vi "Run_old01.vi"(8 "error in (no error)":errorcluster, 11 "Channel in":refnum<class "Channel.lvclass">) -> (0 "error out":errorcluster, 3 "Channel out":refnum<class "Channel.lvclass">)   [LabVIEW 2018, in "Channel.lvclass"]
uses:
  Channel.lvclass
  C:/Users/observer/Desktop/Sparc4GUI/SPARC4_GUI/Device/Device.lvclass
  Channel.lvclass/Channel.ctl
  Interface/Interface.lvclass/Interface.ctl
  Device/Device.lvclass/Device.ctl
  StateMachine/State Machine.lvclass
  Interface/Interface.lvclass
  Device/Device.lvclass
panel:
  out "resp RESUME":string
  out "resp PAUSE":string
  out "error out 2":errorcluster
  out "x = y?":T1
  out "resp ABORT":string
  out "resp STOP":string
  out "resposta do STATUS":string
  out "resp INIT":string
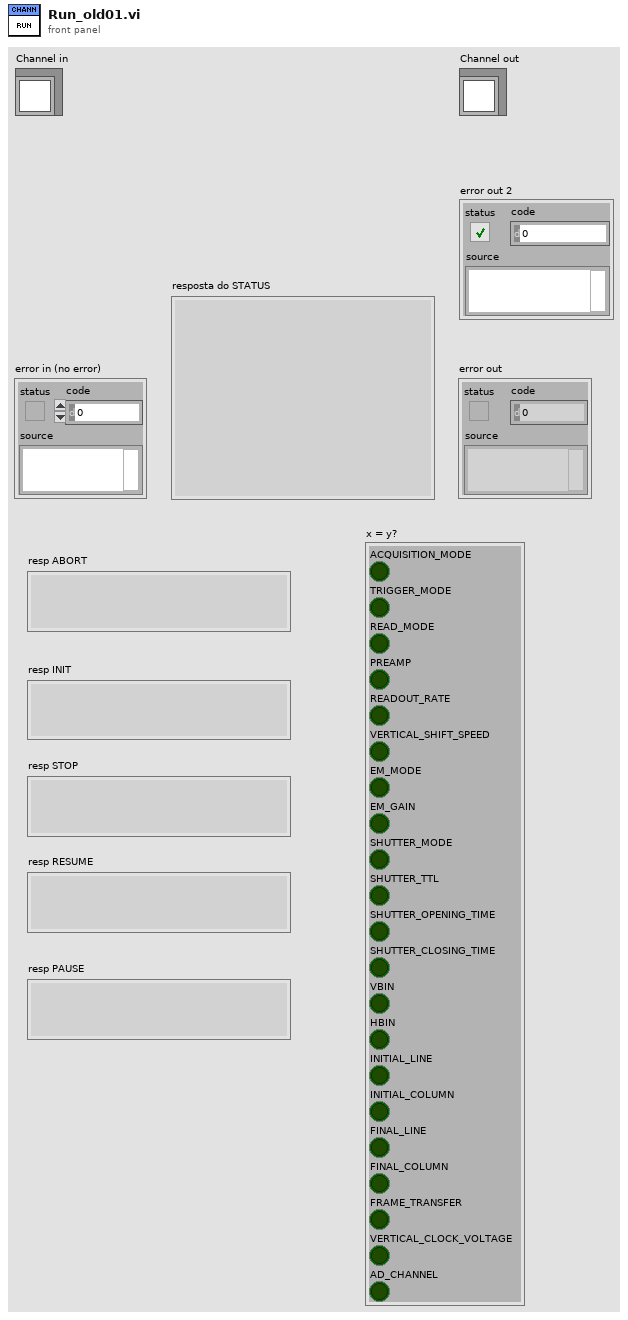
[diagram p1: front panel]
types:
  T1 = cluster{"ACQUISITION_MODE":bool, "TRIGGER_MODE":bool, "READ_MODE":bool, "PREAMP":bool, "READOUT_RATE":bool, "VERTICAL_SHIFT_SPEED":bool, "EM_MODE":bool, "EM_GAIN":bool, "SHUTTER_MODE":bool, "SHUTTER_TTL":bool, "SHUTTER_OPENING_TIME":bool, "SHUTTER_CLOSING_TIME":bool, "VBIN":bool, "HBIN":bool, "INITIAL_LINE":bool, "INITIAL_COLUMN":bool, "FINAL_LINE":bool, "FINAL_COLUMN":bool, "FRAME_TRANSFER":bool, "VERTICAL_CLOCK_VOLTAGE":bool, "AD_CHANNEL":bool}
  T2 = cluster{"ACQUISITION_MODE":u8, "TRIGGER_MODE":u8, "READ_MODE":u8, "PREAMP":u8, "READOUT_RATE":u8, "VERTICAL_SHIFT_SPEED":u8, "EM_MODE":u8, "EM_GAIN":u16, "SHUTTER_MODE":u8, "SHUTTER_TTL":u8, "SHUTTER_OPENING_TIME":u16, "SHUTTER_CLOSING_TIME":u16, "VBIN":u16, "HBIN":u16, "INITIAL_LINE":u16, "INITIAL_COLUMN":u16, "FINAL_LINE":u16, "FINAL_COLUMN":u16, "FRAME_TRANSFER":bool, "VERTICAL_CLOCK_VOLTAGE":u8, "AD_CHANNEL":u32}
  T3 = cluster{"Image Name":string, "Image Path":string, "#FRAMES":u32, "EXPTIME":dbl, "PREAMP":u8, "READOUT_RATE":u8, "VERTICAL_SHIFT_SPEED":u8, "ACQUISITION_MODE":u8, "READ_MODE":u8, "EM_MODE":u8, "EM_GAIN":u16, "SHUTTER_MODE":u8, "SHUTTER_TTL":u8, "SHUTTER_OPENNING_TIME":u16, "SHUTTER_CLOSING_TIME":u16, "VBIN":u16, "HBIN":u16, "INITIAL_LINE":u16, "INITIAL_COLUMN":u16, "FINAL_LINE":u16, "FINAL_COLUMN":u16, "Cooler ON/OFF":u16, "Set temperature":i8, "Exposições realizadas":u16, "Kinetic Serie Length":u32, "Number of Accumulations":u32, "Kinetic Cycle Time":u32, "FRAME_TRANSFER":bool, "VERTICAL_CLOCK_VOLTAGE":u8, "TRIGGER_MODE":u8, "Number of exp":u32, "AD_CHANNEL":u32}
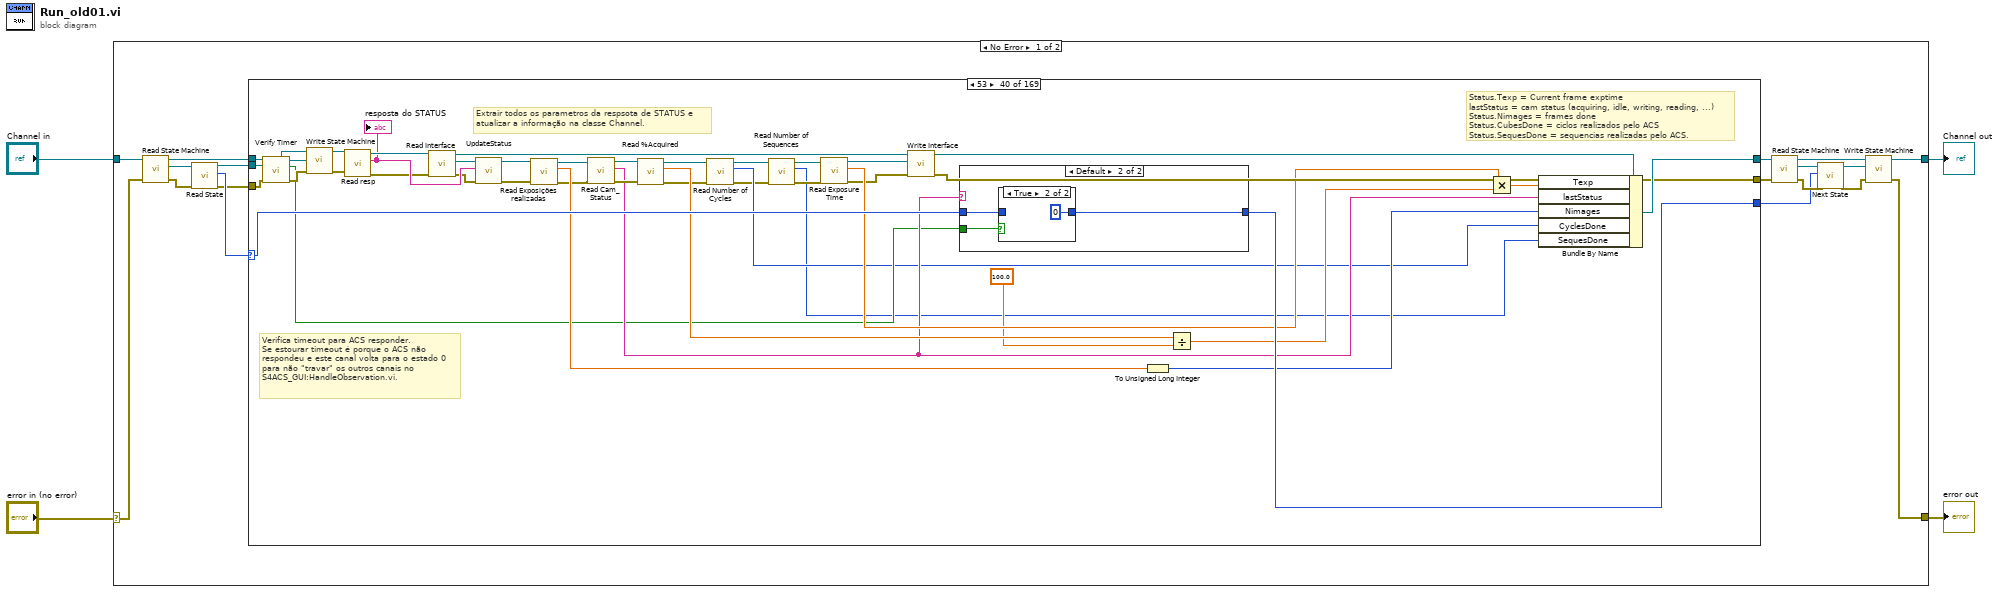
[diagram p0: block diagram]
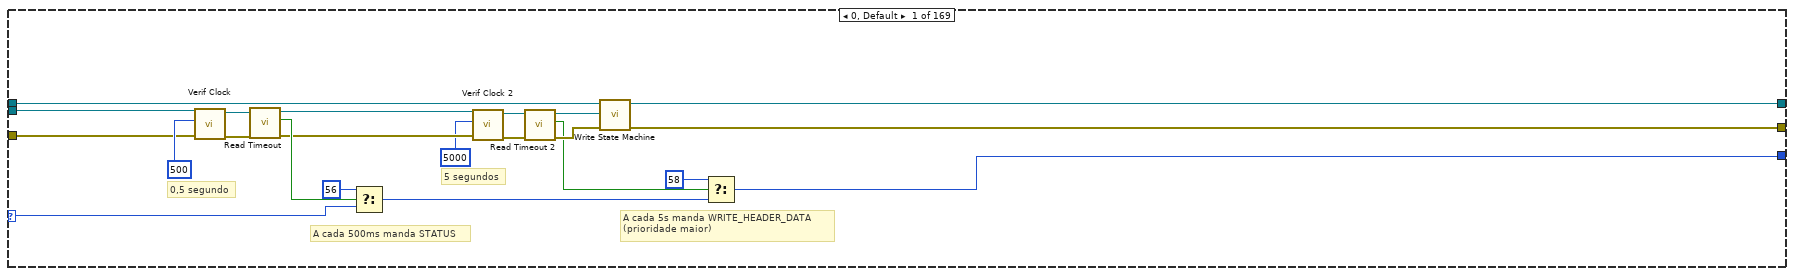
[diagram p2: hidden frame]
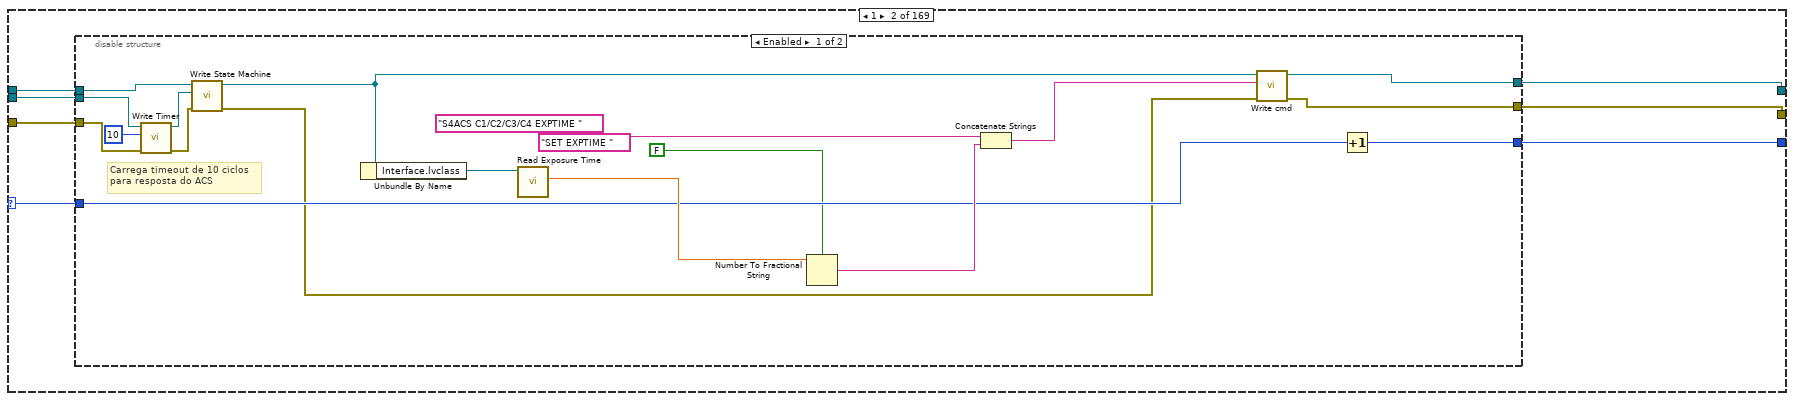
[diagram p3: hidden frame]
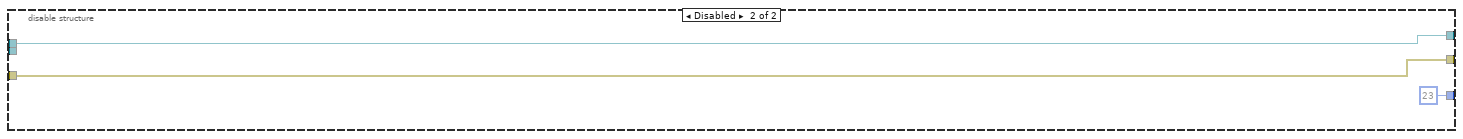
[diagram p4: hidden frame]
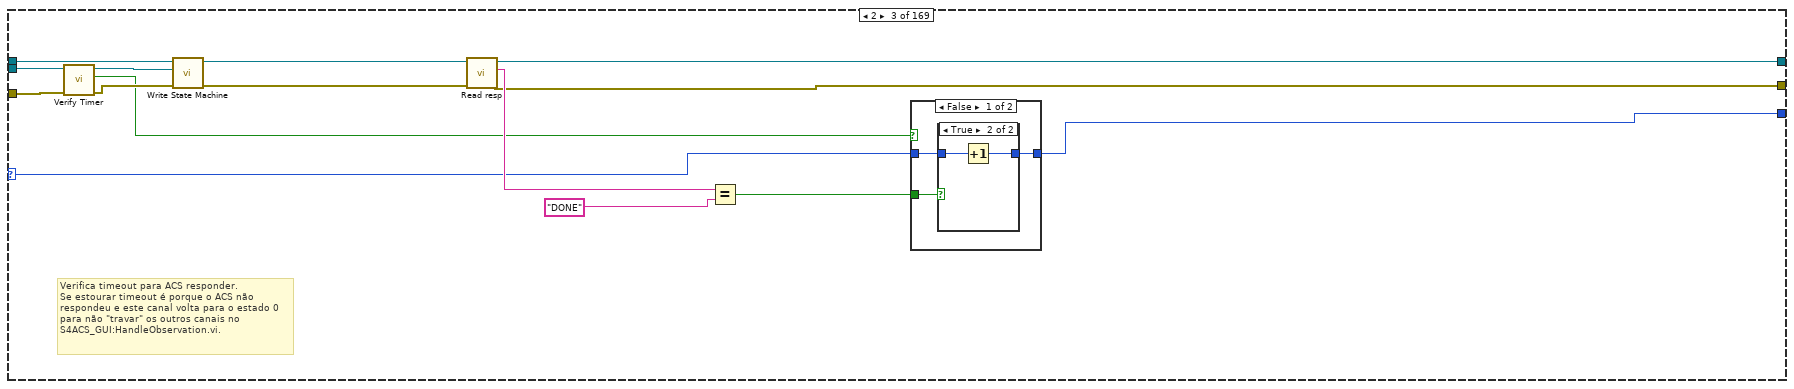
[diagram p5: hidden frame]
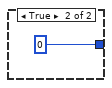
[diagram p7: hidden frame]
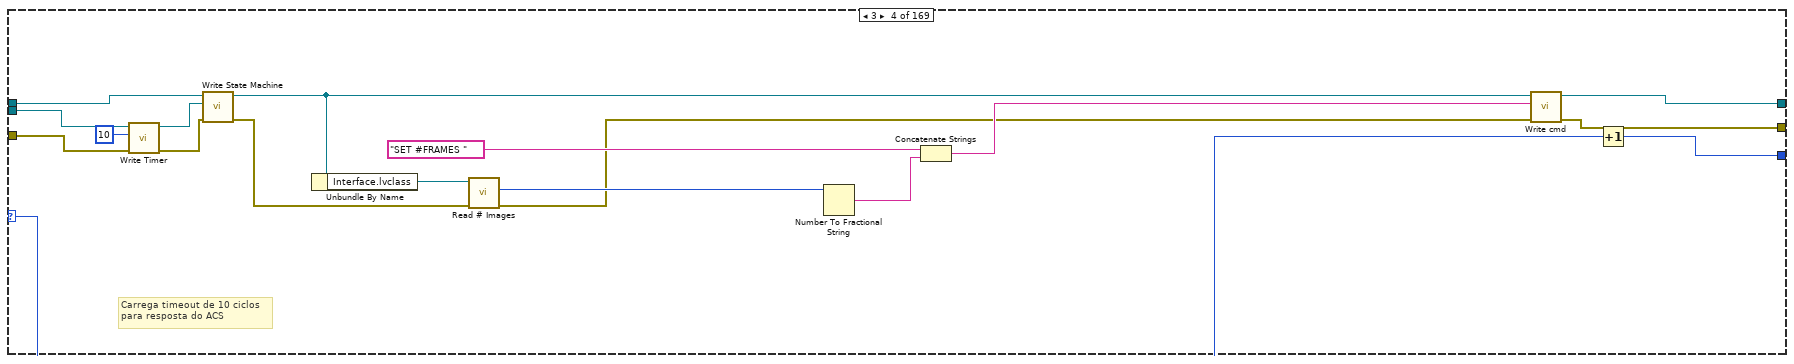
[diagram p8: hidden frame]
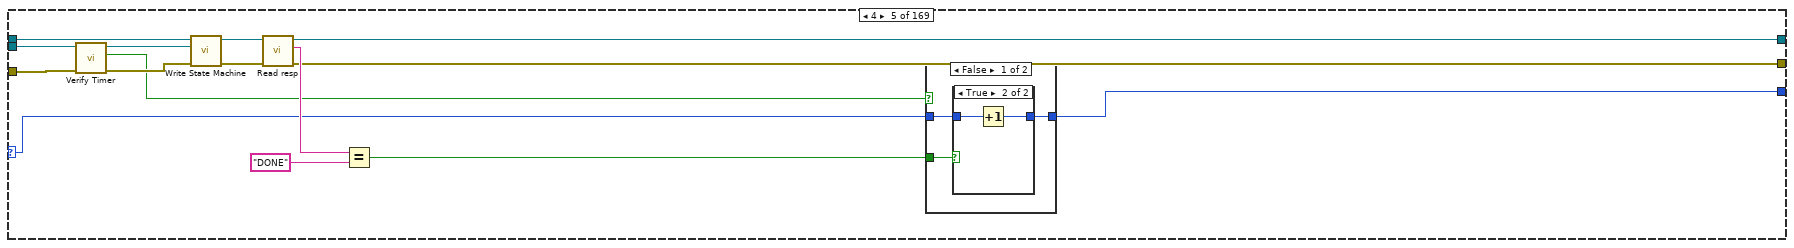
[diagram p9: hidden frame]
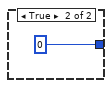
[diagram p11: hidden frame]
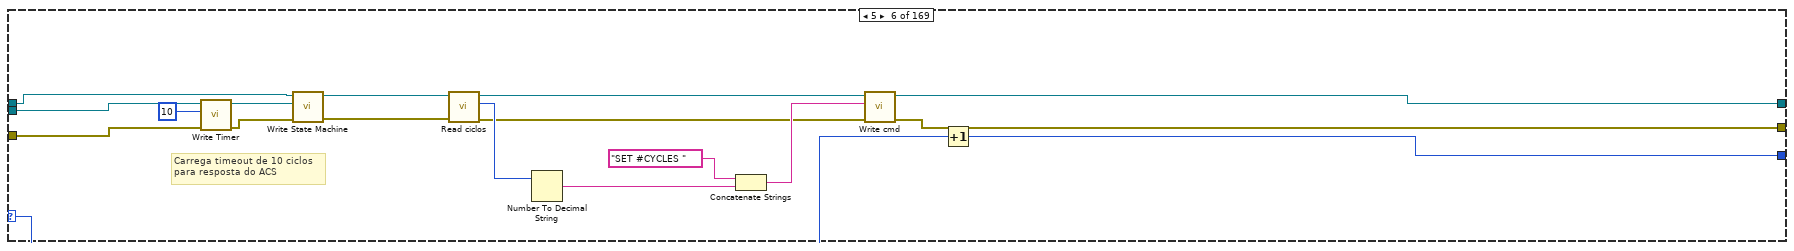
[diagram p12: hidden frame]
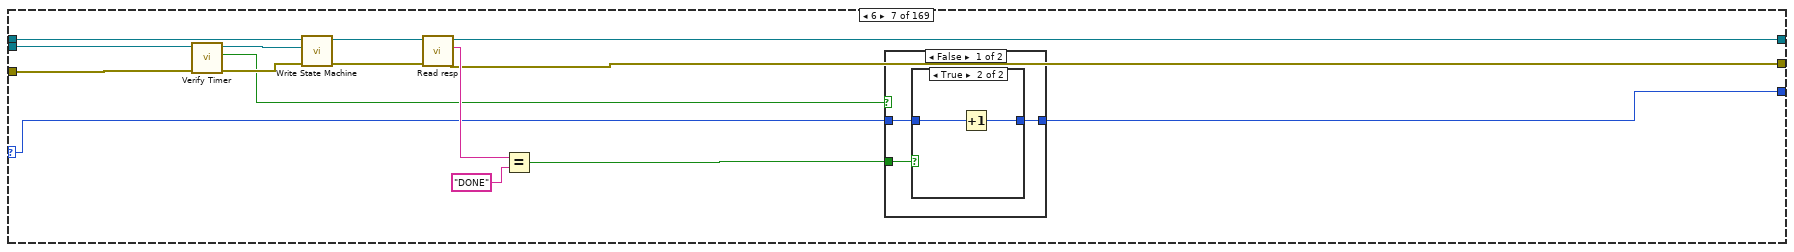
[diagram p13: hidden frame]
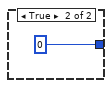
[diagram p15: hidden frame]
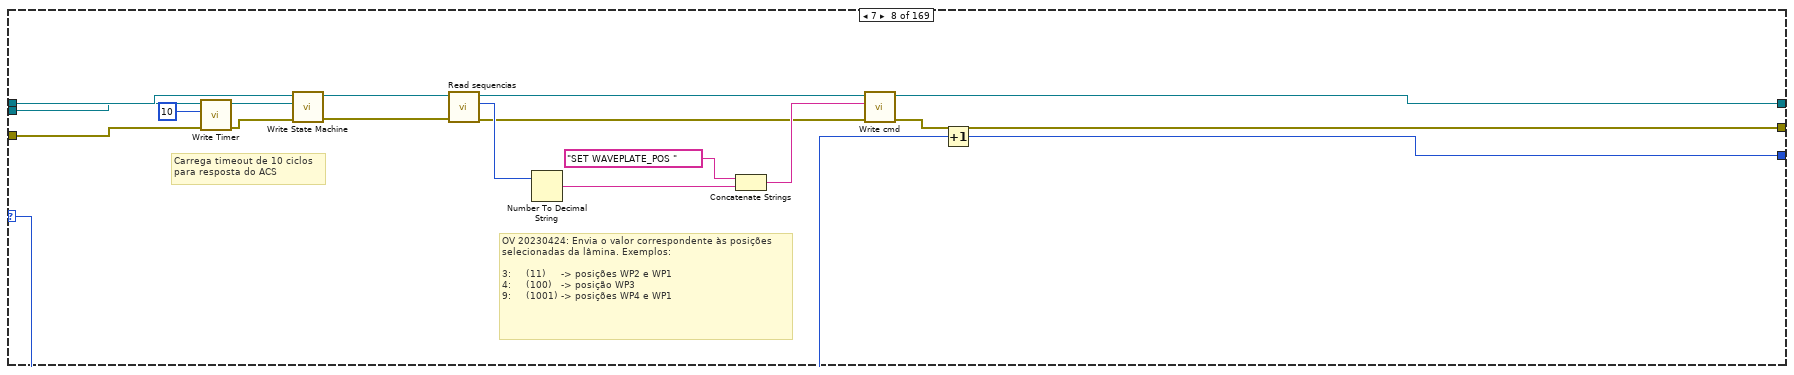
[diagram p16: hidden frame]
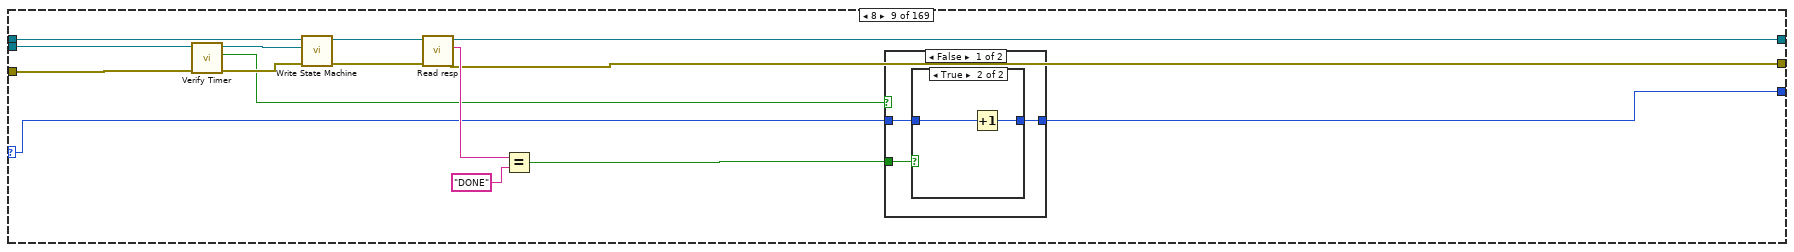
[diagram p17: hidden frame]
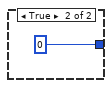
[diagram p19: hidden frame]
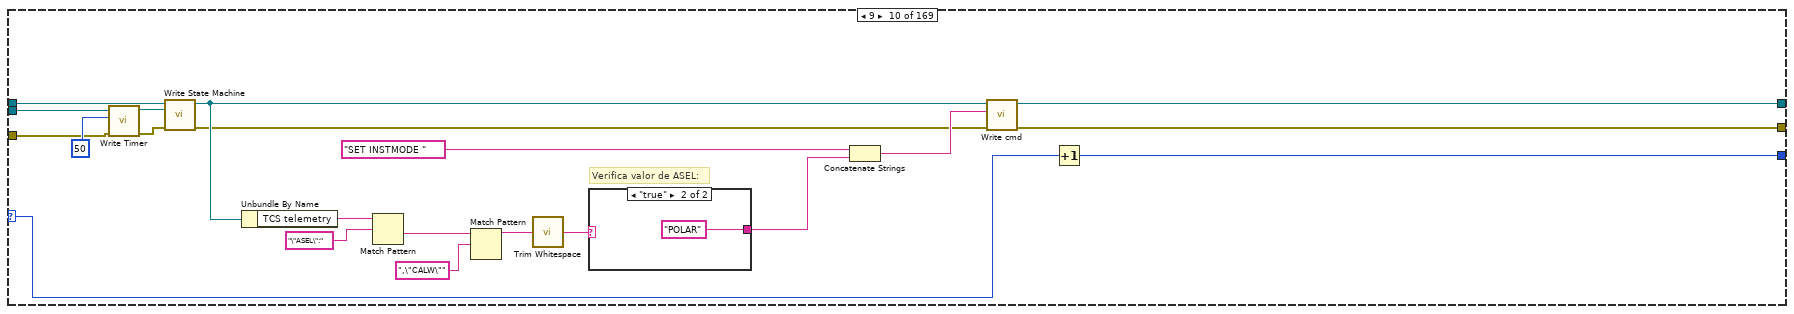
[diagram p20: hidden frame]
diagram:
  n1 = case shown="No Error" "error in (no error)" {
    selector: "error in (no error)" -> [w21 w2733]
    tunnel: [w6 w2733] -> w3
    tunnel: [w11 w2732] -> w1
    tunnel: "Channel in" -> [w22 w2732]
    frame No Error {
      n2 = call-dynamic "Read State Machine.vi"("error in (no error)"=w21, "Device in"=w22) -> ("error out"=w18:errorcluster, "State Machine.lvclass"=w20:refnum<class "State Machine.lvclass">, "Device out"=w16:refnum<class "Channel.lvclass">)  [unwired: 7 in]
      n3 = call-dynamic "Read State.vi"("error in (no error)"=w18, "State Machine in"=w20) -> ("error out"=w17:errorcluster, "State"=w19:i32, "State Machine out"=w5:refnum<class "State Machine.lvclass">)  [unwired: 7 in]
      n4 = case shown="53" w19 {
        selector: w19 -> [w39 w48 w74 w97 w114 w143 w155 w183 w195 w232 w240 w273 w288 w312 w320 w351 w359 w390 w398 w429 w437 w468 w481 w510 w516 w542 w554 w576 w592 w608 w633 w646 w682 w701 _ _ w763 w774 w788 w833 w851 w915 w973 w1021 _ _ w1112 w1144 w1173 w1185 w1199 w1204 w1264 w1286 w1322 w1328 w1342 w1350 w1364 w1371 w1382 _ w1397 w1408 w1428 w1448 w1468 w1488 w1508 w1528 w1548 w1568 _ w1588 w1596 w1609 w1622 w1638 w1646 w1659 w1673 w1685 w1693 w1706 w1719 w1731 w1739 w1752 w1765 w1777 w1785 w1798 w1811 w1823 w1831 w1844 w1857 w1869 w1877 w1890 w1903 w1915 w1923 w1936 w1949 w1961 w1969 w1982 w1995 w2011 w2019 w2032 w2045 w2057 w2065 w2078 w2091 w2103 w2111 w2124 w2137 w2149 w2157 w2170 w2183 w2195 w2203 w2216 w2229 w2241 w2249 w2262 w2275 w2287 w2295 w2308 w2321 w2333 w2341 w2354 w2367 w2379 w2387 w2400 w2413 w2425 w2433 w2446 w2459 w2471 w2479 w2492 w2505 w2521 w2529 w2542 w2555 w2567 w2577 w2590 w2603 w2617 w2625 w2638 w2651 w2664 w2676 w2701 w2713]
        tunnel: w17 -> [w35 w47 w80 w99 w118 w145 w157 w185 w197 w217 w242 w265 w286 w304 w326 w344 w365 w383 w404 w422 w443 w462 w487 w504 w522 w544 w556 w574 w584 w607 w628 w640 w692 w700 w722 w739 w756 w770 w782 w800 w847 w887 w965 w993 w1055 w1087 w1120 w1132 w1167 w1180 w1193 w1221 w1261 w1281 w1315 w1332 w1345 w1354 w1367 w1374 w1385 w1394 w1401 w1412 w1423 w1443 w1463 w1483 w1503 w1523 w1543 w1563 w1581 w1594 w1603 w1613 w1625 w1644 w1653 w1663 w1676 w1691 w1700 w1710 w1722 w1737 w1746 w1756 w1768 w1783 w1792 w1802 w1814 w1829 w1838 w1848 w1860 w1875 w1884 w1894 w1906 w1921 w1930 w1940 w1952 w1967 w1976 w1986 w1998 w2017 w2026 w2036 w2048 w2063 w2072 w2082 w2094 w2109 w2118 w2128 w2140 w2155 w2164 w2174 w2186 w2201 w2210 w2220 w2232 w2247 w2256 w2266 w2278 w2293 w2302 w2312 w2324 w2339 w2348 w2358 w2370 w2385 w2394 w2404 w2416 w2431 w2440 w2450 w2462 w2477 w2486 w2496 w2508 w2527 w2536 w2546 w2558 w2573 w2584 w2594 w2606 w2623 w2632 w2642 w2654 w2666 w2678 w2703 w2715]
        tunnel: [w34 w50 w84 w111 w124 w151 w164 w191 w204 w234 w249 w277 w289 w316 w329 w355 w368 w394 w407 w433 w446 w471 w490 w512 w525 w550 w563 w574 w596 w609 w635 w648 w691 w702 w727 w743 w764 w766 w790 w825 w853 w888 w960 w994 w1067 w1098 w1119 w1145 w1175 w1177 w1201 w1205 w1266 w1287 w1302 w1329 w1338 w1351 w1360 w1372 w1378 w1387 w1400 w1409 w1423 w1443 w1463 w1483 w1503 w1523 w1543 w1563 w1581 w1593 w1597 w1612 w1623 w1643 w1647 w1662 w1674 w1690 w1694 w1709 w1720 w1736 w1740 w1755 w1766 w1782 w1786 w1801 w1812 w1828 w1832 w1847 w1858 w1874 w1878 w1893 w1904 w1920 w1924 w1939 w1950 w1966 w1970 w1985 w1996 w2016 w2020 w2035 w2046 w2062 w2066 w2081 w2092 w2108 w2112 w2127 w2138 w2154 w2158 w2173 w2184 w2200 w2204 w2219 w2230 w2246 w2250 w2265 w2276 w2292 w2296 w2311 w2322 w2338 w2342 w2357 w2368 w2384 w2388 w2403 w2414 w2430 w2434 w2449 w2460 w2476 w2480 w2495 w2506 w2526 w2530 w2545 w2556 w2572 w2578 w2593 w2604 w2622 w2626 w2641 w2652 w2672 w2685 w2709 w2722] -> w7
        tunnel: w16 -> [w38 w45 w83 w100 w122 w146 w161 w186 w201 w219 w246 w267 w285 w306 w327 w346 w366 w385 w405 w424 w444 w464 w488 w506 w523 w545 w560 w573 w587 w606 w630 w643 w690 w699 w725 w740 w758 w773 w784 w803 w850 w885 w967 w987 w1066 w1097 w1114 w1136 w1168 w1181 w1194 w1222 w1260 w1284 w1316 w1333 w1344 w1355 w1366 w1375 w1384 w1395 w1399 w1413 w1421 w1441 w1461 w1481 w1501 w1521 w1541 w1561 w1583 w1592 w1604 w1611 w1626 w1642 w1654 w1661 w1677 w1689 w1701 w1708 w1723 w1735 w1747 w1754 w1769 w1781 w1793 w1800 w1815 w1827 w1839 w1846 w1861 w1873 w1885 w1892 w1907 w1919 w1931 w1938 w1953 w1965 w1977 w1984 w1999 w2015 w2027 w2034 w2049 w2061 w2073 w2080 w2095 w2107 w2119 w2126 w2141 w2153 w2165 w2172 w2187 w2199 w2211 w2218 w2233 w2245 w2257 w2264 w2279 w2291 w2303 w2310 w2325 w2337 w2349 w2356 w2371 w2383 w2395 w2402 w2417 w2429 w2441 w2448 w2463 w2475 w2487 w2494 w2509 w2525 w2537 w2544 w2559 w2571 w2585 w2592 w2607 w2621 w2633 w2640 w2655 w2667 w2682 w2704 w2719]
        tunnel: [w37 w51 w85 w112 w125 w152 w165 w192 w205 w235 w250 w278 w290 w317 w330 w356 w369 w395 w408 w434 w447 w472 w491 w513 w526 w551 w564 w573 w597 w610 w636 w651 w683 w703 w728 w744 w765 w767 w791 w832 w854 w914 w961 w1020 w1068 w1099 w1121 w1146 w1176 w1178 w1202 w1217 w1267 w1288 w1308 w1330 w1337 w1352 w1359 w1373 w1377 w1393 w1402 w1405 w1425 w1445 w1465 w1485 w1505 w1525 w1545 w1565 w1583 w1595 w1598 w1614 w1621 w1645 w1648 w1664 w1672 w1692 w1695 w1711 w1718 w1738 w1741 w1757 w1764 w1784 w1787 w1803 w1810 w1830 w1833 w1849 w1856 w1876 w1879 w1895 w1902 w1922 w1925 w1941 w1948 w1968 w1971 w1987 w1994 w2018 w2021 w2037 w2044 w2064 w2067 w2083 w2090 w2110 w2113 w2129 w2136 w2156 w2159 w2175 w2182 w2202 w2205 w2221 w2228 w2248 w2251 w2267 w2274 w2294 w2297 w2313 w2320 w2340 w2343 w2359 w2366 w2386 w2389 w2405 w2412 w2432 w2435 w2451 w2458 w2478 w2481 w2497 w2504 w2528 w2531 w2547 w2554 w2574 w2579 w2595 w2602 w2624 w2627 w2643 w2650 w2673 w2686 w2710 w2723] -> w14
        tunnel: [w33 w49 w73 w106 w113 w150 w156 w190 w196 w233 w241 w274 w291 w313 w318 w352 w357 w391 w396 w430 w435 w469 w479 w511 w514 w549 w555 w577 w593 w611 w634 w647 w684 w704 31 ("State") 0 ("State") w752 w775 w789 w834 w852 w916 w974 w1022 0 ("State") 54 ("State") w1111 w1147 w1174 w1186 w1200 w1203 w1265 w1289 w1323 w1331 w1343 w1353 w1365 w1371 w1383 w1386 w1398 w1410 w1420 w1440 w1460 w1480 w1500 w1520 w1540 w1560 u8 0 ("State") w1589 w1599 w1610 w1624 w1639 w1649 w1660 w1675 w1686 w1696 w1707 w1721 w1732 w1742 w1753 w1767 w1778 w1788 w1799 w1813 w1824 w1834 w1845 w1859 w1870 w1880 w1891 w1905 w1916 w1926 w1937 w1951 w1962 w1972 w1983 w1997 w2012 w2022 w2033 w2047 w2058 w2068 w2079 w2093 w2104 w2114 w2125 w2139 w2150 w2160 w2171 w2185 w2196 w2206 w2217 w2231 w2242 w2252 w2263 w2277 w2288 w2298 w2309 w2323 w2334 w2344 w2355 w2369 w2380 w2390 w2401 w2415 w2426 w2436 w2447 w2461 w2472 w2482 w2493 w2507 w2522 w2532 w2543 w2557 w2568 w2580 w2591 w2605 w2618 w2628 w2639 w2653 w2671 w2677 w2708 w2714] -> w8
        tunnel: w5 -> [w36 w46 w82 w101 w123 w144 w158 w184 w198 w215 w243 w269 w287 w301 w324 w340 w363 w379 w402 w418 w441 w460 w485 w503 w520 w543 w557 _ w586 w604 w629 w644 _ w697 w724 w741 w759 w772 w783 w805 w848 w886 w969 w992 w1056 w1088 w1116 w1137 w1170 w1182 w1196 w1223 w1262 w1285 w1317 _ _ _ _ _ _ w1389 _ _ _ _ _ _ _ _ _ _ _ _ _ _ _ _ _ _ _ _ _ _ _ _ _ _ _ _ _ _ _ _ _ _ _ _ _ _ _ _ _ _ _ _ _ _ _ _ _ _ _ _ _ _ _ _ _ _ _ _ _ _ _ _ _ _ _ _ _ _ _ _ _ _ _ _ _ _ _ _ _ _ _ _ _ _ _ _ _ _ _ _ _ _ _ _ _ _ _ _ _ _ _ w2665 w2679 w2702 w2716]
        frame 0, Default {
          # "5 segundos"
          # "A cada 5s manda WRITE_HEADER_DATA\n(prioridade maior)"
          # "A cada 500ms manda STATUS"
          # "0,5 segundo"
          n5 = call-dynamic "Verif Clock.vi"("error in (no error)"=w35, "period"=u32 500, "State Machine in"=w36) -> ("error out"=w42:errorcluster, "State Machine out"=w41:refnum<class "State Machine.lvclass">)  [unwired: 7 in]
          n6 = call-dynamic "Read Timeout.vi"("error in (no error)"=w42, "State Machine in"=w41) -> ("error out"=w27:errorcluster, "Timeout"=w43:bool, "State Machine out"=w30:refnum<class "State Machine.lvclass">)  [unwired: 7 in]
          n7 = Select(t=56 ("State"), s=w43, f=w39) -> (s? t:f=w31:i32)
          n8 = call-dynamic "Verif Clock 2.vi"("error in (no error)"=w27, "period"=u32 5000, "State Machine in"=w30) -> ("error out"=w26:errorcluster, "State Machine out"=w29:refnum<class "State Machine.lvclass">)  [unwired: 7 in]
          n9 = call-dynamic "Read Timeout 2.vi"("error in (no error)"=w26, "State Machine in"=w29) -> ("error out"=w25:errorcluster, "Timeout 2"=w23:bool, "State Machine out"=w28:refnum<class "State Machine.lvclass">)  [unwired: 7 in]
          n10 = call-dynamic "Write State Machine.vi"("error in (no error)"=w25, "State Machine.lvclass"=w28, "Device in"=w38) -> ("error out"=w34:errorcluster, "Device out"=w37:refnum<class "Channel.lvclass">)  [unwired: 7 in]
          n11 = Select(t=58 ("f"), s=w23, f=w31) -> (s? t:f=w33:i32)
        }
        frame 1 {
          n12 = disable-structure shown="Enabled" {
            disable-tunnel: [w69 w72] -> w51
            disable-tunnel: [w68 w71] -> w50
            disable-tunnel: [w63 23] -> w49
            disable-tunnel: w48 -> [w62 _]
            disable-tunnel: w47 -> [w59 w71]
            disable-tunnel: w46 -> [w58 _]
            disable-tunnel: w45 -> [w57 w72]
            frame Enabled {
              (unwired) "S4ACS C1/C2/C3/C4 EXPTIME " ("cmd")
              # "Carrega timeout de 10 ciclos\npara resposta do ACS"
              n13 = call-dynamic "Write Timer.vi"("error in (no error)"=w59, "Timer"=u32 10, "State Machine in"=w58) -> ("error out"=w53:errorcluster, "State Machine out"=w56:refnum<class "State Machine.lvclass">)  [unwired: 7 in]
              n14 = call-dynamic "Write State Machine.vi"("error in (no error)"=w53, "State Machine.lvclass"=w56, "Device in"=w57) -> ("error out"=w52:errorcluster, "Device out"=w55:refnum<class "Channel.lvclass">)  [unwired: 7 in]
              n15 = Unbundle By Name(w55) -> ("Interface.lvclass"=w67:refnum<class "Interface.lvclass">)
              n16 = call "Read Exposure Time.vi"("Interface in"=w67) -> ("Exposure Time"=w66:dbl)  [unwired: 8 in, 2 out]
              n17 = Number To Fractional String(use system decimal point (T)=FALSE, number=w66) -> (F-format string=w65:string)  [unwired: 2 in]
              n18 = Concatenate Strings("SET EXPTIME " ("cmd"), w65) -> (w64:string)
              n19 = call-dynamic "Write cmd.vi"("error in (no error)"=w52, "cmd"=w64, "Device in"=w55) -> ("error out"=w68:errorcluster, "Device out"=w69:refnum<class "Channel.lvclass">)  [unwired: 7 in]
              n20 = Increment(x=w62) -> (x+1=w63:i32)
            }
            frame Disabled {
            }
          }
        }
        frame 2 {
          # "Verifica timeout para ACS responder.\nSe estourar timeout é porque o ACS não \nrespondeu e este canal volta para o estado 0\npara não \"travar\" os outros canais no \nS4ACS_GUI:HandleObservation.vi."
          n21 = call "Verify Timer.vi"("error in (no error)"=w80, "State Machine in"=w82) -> ("error out"=w79:errorcluster, "timeout"=w75:bool, "State Machine out"=w81:refnum<class "State Machine.lvclass">)  [unwired: 7 in]
          n22 = call-dynamic "Write State Machine.vi"("error in (no error)"=w79, "State Machine.lvclass"=w81, "Device in"=w83) -> ("error out"=w78:errorcluster, "Device out"=w77:refnum<class "Channel.lvclass">)  [unwired: 7 in]
          n23 = call-dynamic "Read resp.vi"("error in (no error)"=w78, "Device in"=w77) -> ("error out"=w84:errorcluster, "resp"=w87:string, "Device out"=w85:refnum<class "Channel.lvclass">)  [unwired: 7 in]
          n24 = Equal?(x=w87, y="DONE") -> (x = y?=w76:bool)
          n25 = case shown="False" w75 {
            tunnel: [w89 0] -> w73
            tunnel: w74 -> [w90 _]
            tunnel: w76 -> [w88 _]
            frame False {
              n26 = case shown="True" w88 {
                tunnel: [w91 w92] -> w89
                tunnel: w90 -> [w91 w93]
                frame False {
                }
                frame True {
                  n27 = Increment(x=w93) -> (x+1=w92:i32)
                }
              }
            }
            frame True {
            }
          }
        }
        frame 3 {
          # "Carrega timeout de 10 ciclos\npara resposta do ACS"
          n28 = call-dynamic "Write Timer.vi"("error in (no error)"=w99, "Timer"=u32 10, "State Machine in"=w101) -> ("error out"=w102:errorcluster, "State Machine out"=w104:refnum<class "State Machine.lvclass">)  [unwired: 7 in]
          n29 = call-dynamic "Write State Machine.vi"("error in (no error)"=w102, "State Machine.lvclass"=w104, "Device in"=w100) -> ("error out"=w96:errorcluster, "Device out"=w98:refnum<class "Channel.lvclass">)  [unwired: 7 in]
          n30 = Unbundle By Name(w98) -> ("Interface.lvclass"=w110:refnum<class "Interface.lvclass">)
          n31 = call-dynamic "Read # Images.vi"("error in (no error)"=w96, "Interface in"=w110) -> ("error out"=w95:errorcluster, "# Images"=w109:u32)  [unwired: 7 in, 1 out]
          n32 = Number To Fractional String(number=w109) -> (F-format string=w108:string)  [unwired: 3 in]
          n33 = Concatenate Strings("SET #FRAMES " ("cmd"), w108) -> (w107:string)
          n34 = call-dynamic "Write cmd.vi"("error in (no error)"=w95, "cmd"=w107, "Device in"=w98) -> ("error out"=w111:errorcluster, "Device out"=w112:refnum<class "Channel.lvclass">)  [unwired: 7 in]
          n35 = Increment(x=w97) -> (x+1=w106:i32)
        }
        frame 4 {
          n36 = call "Verify Timer.vi"("error in (no error)"=w118, "State Machine in"=w123) -> ("error out"=w117:errorcluster, "timeout"=w116:bool, "State Machine out"=w119:refnum<class "State Machine.lvclass">)  [unwired: 7 in]
          n37 = call-dynamic "Write State Machine.vi"("error in (no error)"=w117, "State Machine.lvclass"=w119, "Device in"=w122) -> ("error out"=w120:errorcluster, "Device out"=w121:refnum<class "Channel.lvclass">)  [unwired: 7 in]
          n38 = call-dynamic "Read resp.vi"("error in (no error)"=w120, "Device in"=w121) -> ("error out"=w124:errorcluster, "resp"=w127:string, "Device out"=w125:refnum<class "Channel.lvclass">)  [unwired: 7 in]
          n39 = Equal?(x=w127, y="DONE") -> (x = y?=w115:bool)
          n40 = case shown="False" w116 {
            tunnel: [w129 0] -> w113
            tunnel: w114 -> [w130 _]
            tunnel: w115 -> [w128 _]
            frame False {
              n41 = case shown="True" w128 {
                tunnel: [w131 w132] -> w129
                tunnel: w130 -> [w131 w133]
                frame False {
                }
                frame True {
                  n42 = Increment(x=w133) -> (x+1=w132:i32)
                }
              }
            }
            frame True {
            }
          }
        }
        frame 5 {
          # "Carrega timeout de 10 ciclos\npara resposta do ACS"
          n43 = call-dynamic "Write Timer.vi"("error in (no error)"=w145, "Timer"=u32 10, "State Machine in"=w144) -> ("error out"=w147:errorcluster, "State Machine out"=w149:refnum<class "State Machine.lvclass">)  [unwired: 7 in]
          n44 = call-dynamic "Write State Machine.vi"("error in (no error)"=w147, "State Machine.lvclass"=w149, "Device in"=w146) -> ("error out"=w141:errorcluster, "Device out"=w142:refnum<class "Channel.lvclass">)  [unwired: 7 in]
          n45 = call-dynamic "Read ciclos.vi"("error in (no error)"=w141, "Channel in"=w142) -> ("error out"=w135:errorcluster, "ciclos"=w139:u32, "Channel out"=w140:refnum<class "Channel.lvclass">)  [unwired: 7 in]
          n46 = Number To Decimal String(number=w139) -> (decimal integer string=w137:string)  [unwired: 1 in]
          n47 = Concatenate Strings("SET #CYCLES " ("cmd"), w137) -> (w136:string)
          n48 = call-dynamic "Write cmd.vi"("error in (no error)"=w135, "cmd"=w136, "Device in"=w140) -> ("error out"=w151:errorcluster, "Device out"=w152:refnum<class "Channel.lvclass">)  [unwired: 7 in]
          n49 = Increment(x=w143) -> (x+1=w150:i32)
        }
        frame 6 {
          n50 = call "Verify Timer.vi"("error in (no error)"=w157, "State Machine in"=w158) -> ("error out"=w162:errorcluster, "timeout"=w154:bool, "State Machine out"=w163:refnum<class "State Machine.lvclass">)  [unwired: 7 in]
          n51 = call-dynamic "Write State Machine.vi"("error in (no error)"=w162, "State Machine.lvclass"=w163, "Device in"=w161) -> ("error out"=w159:errorcluster, "Device out"=w160:refnum<class "Channel.lvclass">)  [unwired: 7 in]
          n52 = call-dynamic "Read resp.vi"("error in (no error)"=w159, "Device in"=w160) -> ("error out"=w164:errorcluster, "resp"=w167:string, "Device out"=w165:refnum<class "Channel.lvclass">)  [unwired: 7 in]
          n53 = Equal?(x=w167, y="DONE") -> (x = y?=w153:bool)
          n54 = case shown="False" w154 {
            tunnel: [w169 0] -> w156
            tunnel: w155 -> [w170 _]
            tunnel: w153 -> [w168 _]
            frame False {
              n55 = case shown="True" w168 {
                tunnel: [w171 w172] -> w169
                tunnel: w170 -> [w171 w173]
                frame False {
                }
                frame True {
                  n56 = Increment(x=w173) -> (x+1=w172:i32)
                }
              }
            }
            frame True {
            }
          }
        }
        frame 7 {
          # "OV 20230424: Envia o valor correspondente às posições\nselecionadas da lâmina. Exemplos:\n\n3:     (11)     -> posições WP2 e WP1\n4:     (100)   -> posição WP3\n9:     (1001) -> posições WP4 e WP1"
          # "Carrega timeout de 10 ciclos\npara resposta do ACS"
          n57 = call-dynamic "Write Timer.vi"("error in (no error)"=w185, "Timer"=u32 10, "State Machine in"=w184) -> ("error out"=w187:errorcluster, "State Machine out"=w189:refnum<class "State Machine.lvclass">)  [unwired: 7 in]
          n58 = call-dynamic "Write State Machine.vi"("error in (no error)"=w187, "State Machine.lvclass"=w189, "Device in"=w186) -> ("error out"=w181:errorcluster, "Device out"=w182:refnum<class "Channel.lvclass">)  [unwired: 7 in]
          n59 = call-dynamic "Read sequencias.vi"("error in (no error)"=w181, "Channel in"=w182) -> ("error out"=w175:errorcluster, "sequencias"=w179:u32, "Channel out"=w180:refnum<class "Channel.lvclass">)  [unwired: 7 in]
          n60 = Number To Decimal String(number=w179) -> (decimal integer string=w177:string)  [unwired: 1 in]
          n61 = Concatenate Strings("SET WAVEPLATE_POS " ("cmd"), w177) -> (w176:string)
          n62 = call-dynamic "Write cmd.vi"("error in (no error)"=w175, "cmd"=w176, "Device in"=w180) -> ("error out"=w191:errorcluster, "Device out"=w192:refnum<class "Channel.lvclass">)  [unwired: 7 in]
          n63 = Increment(x=w183) -> (x+1=w190:i32)
        }
        frame 8 {
          n64 = call "Verify Timer.vi"("error in (no error)"=w197, "State Machine in"=w198) -> ("error out"=w202:errorcluster, "timeout"=w194:bool, "State Machine out"=w203:refnum<class "State Machine.lvclass">)  [unwired: 7 in]
          n65 = call-dynamic "Write State Machine.vi"("error in (no error)"=w202, "State Machine.lvclass"=w203, "Device in"=w201) -> ("error out"=w199:errorcluster, "Device out"=w200:refnum<class "Channel.lvclass">)  [unwired: 7 in]
          n66 = call-dynamic "Read resp.vi"("error in (no error)"=w199, "Device in"=w200) -> ("error out"=w204:errorcluster, "resp"=w207:string, "Device out"=w205:refnum<class "Channel.lvclass">)  [unwired: 7 in]
          n67 = Equal?(x=w207, y="DONE") -> (x = y?=w193:bool)
          n68 = case shown="False" w194 {
            tunnel: [w209 0] -> w196
            tunnel: w195 -> [w210 _]
            tunnel: w193 -> [w208 _]
            frame False {
              n69 = case shown="True" w208 {
                tunnel: [w211 w212] -> w209
                tunnel: w210 -> [w211 w213]
                frame False {
                }
                frame True {
                  n70 = Increment(x=w213) -> (x+1=w212:i32)
                }
              }
            }
            frame True {
            }
          }
        }
        frame 9 {
          # "Verifica valor de ASEL:"
          n71 = call-dynamic "Write Timer.vi"("error in (no error)"=w217, "Timer"=u32 50, "State Machine in"=w215) -> ("error out"=w222:errorcluster, "State Machine out"=w220:refnum<class "State Machine.lvclass">)  [unwired: 7 in]
          n72 = call-dynamic "Write State Machine.vi"("error in (no error)"=w222, "State Machine.lvclass"=w220, "Device in"=w219) -> ("error out"=w216:errorcluster, "Device out"=w218:refnum<class "Channel.lvclass">)  [unwired: 7 in]
          n73 = Unbundle By Name(w218) -> ("TCS telemetry"=w231:string)
          n74 = Match Pattern(string=w231, regular expression="\"ASEL\":") -> (after substring=w229:string)  [unwired: 1 in, 3 out]
          n75 = Match Pattern(string=w229, regular expression=",\"CALW\"") -> (before substring=w227:string)  [unwired: 1 in, 3 out]
          n76 = call <vilib>:"Trim Whitespace.vi"("string"=w227) -> ("trimmed string"=w226:string)  [unwired: 1 in]
          n77 = case shown="\"true\"" w226 {
            tunnel: ["PHOT" ("regular expression") "POLAR" ("regular expression")] -> w224
            frame "false", Default {
            }
            frame "true" {
            }
          }
          n78 = Concatenate Strings("SET INSTMODE " ("cmd"), w224) -> (w223:string)
          n79 = call-dynamic "Write cmd.vi"("error in (no error)"=w216, "cmd"=w223, "Device in"=w218) -> ("error out"=w234:errorcluster, "Device out"=w235:refnum<class "Channel.lvclass">)  [unwired: 7 in]
          n80 = Increment(x=w232) -> (x+1=w233:i32)
        }
        frame 10 {
          n81 = call "Verify Timer.vi"("error in (no error)"=w242, "State Machine in"=w243) -> ("error out"=w247:errorcluster, "timeout"=w239:bool, "State Machine out"=w248:refnum<class "State Machine.lvclass">)  [unwired: 7 in]
          n82 = call-dynamic "Write State Machine.vi"("error in (no error)"=w247, "State Machine.lvclass"=w248, "Device in"=w246) -> ("error out"=w244:errorcluster, "Device out"=w245:refnum<class "Channel.lvclass">)  [unwired: 7 in]
          n83 = call-dynamic "Read resp.vi"("error in (no error)"=w244, "Device in"=w245) -> ("error out"=w249:errorcluster, "resp"=w252:string, "Device out"=w250:refnum<class "Channel.lvclass">)  [unwired: 7 in]
          n84 = Equal?(x=w252, y="DONE") -> (x = y?=w238:bool)
          n85 = case shown="False" w239 {
            tunnel: [w254 0] -> w241
            tunnel: w240 -> [w255 _]
            tunnel: w238 -> [w253 _]
            frame False {
              n86 = case shown="True" w253 {
                tunnel: [w256 w257] -> w254
                tunnel: w255 -> [w256 w258]
                frame False {
                }
                frame True {
                  n87 = disable-structure shown="Enabled" {
                    disable-tunnel: w258 -> [w260 _]
                    disable-tunnel: [w259 29 ("State")] -> w257
                    frame Disabled {
                      n88 = Increment(x=w260) -> (x+1=w259:i32)
                    }
                    frame Enabled {
                    }
                  }
                }
              }
            }
            frame True {
            }
          }
        }
        frame 12 {
          # "suffix"
          n89 = call-dynamic "Write Timer.vi"("error in (no error)"=w265, "Timer"=u32 50, "State Machine in"=w269) -> ("error out"=w270:errorcluster, "State Machine out"=w263:refnum<class "State Machine.lvclass">)  [unwired: 7 in]
          n90 = call-dynamic "Write State Machine.vi"("error in (no error)"=w270, "State Machine.lvclass"=w263, "Device in"=w267) -> ("error out"=w264:errorcluster, "Device out"=w266:refnum<class "Channel.lvclass">)  [unwired: 7 in]
          n91 = Unbundle By Name(w266) -> ("Interface.lvclass"=w276:refnum<class "Interface.lvclass">)
          n92 = call-dynamic "Read Suffix.vi"("Interface in"=w276) -> ("Suffix"=w271:string)  [unwired: 8 in, 2 out]
          n93 = Concatenate Strings("SET SUFFIX " ("cmd"), w271) -> (w275:string)
          n94 = call-dynamic "Write cmd.vi"("error in (no error)"=w264, "cmd"=w275, "Device in"=w266) -> ("error out"=w277:errorcluster, "Device out"=w278:refnum<class "Channel.lvclass">)  [unwired: 7 in]
          n95 = Increment(x=w273) -> (x+1=w274:i32)
        }
        frame 13 {
          n96 = call "Verify Timer.vi"("error in (no error)"=w286, "State Machine in"=w287) -> ("error out"=w283:errorcluster, "timeout"=w280:bool, "State Machine out"=w284:refnum<class "State Machine.lvclass">)  [unwired: 7 in]
          n97 = call-dynamic "Write State Machine.vi"("error in (no error)"=w283, "State Machine.lvclass"=w284, "Device in"=w285) -> ("error out"=w282:errorcluster, "Device out"=w281:refnum<class "Channel.lvclass">)  [unwired: 7 in]
          n98 = call-dynamic "Read resp.vi"("error in (no error)"=w282, "Device in"=w281) -> ("error out"=w289:errorcluster, "resp"=w293:string, "Device out"=w290:refnum<class "Channel.lvclass">)  [unwired: 7 in]
          n99 = Equal?(x=w293, y="DONE") -> (x = y?=w279:bool)
          n100 = case shown="False" w280 {
            tunnel: [w295 0] -> w291
            tunnel: w288 -> [w296 _]
            tunnel: w279 -> [w294 _]
            frame False {
              n101 = case shown="True" w294 {
                tunnel: w296 -> [w297 w299]
                tunnel: [w297 w298] -> w295
                frame False {
                }
                frame True {
                  n102 = Increment(x=w299) -> (x+1=w298:i32)
                }
              }
            }
            frame True {
            }
          }
        }
        frame 14 {
          # "obstype"
          n103 = call-dynamic "Write Timer.vi"("error in (no error)"=w304, "Timer"=u32 50, "State Machine in"=w301) -> ("error out"=w309:errorcluster, "State Machine out"=w307:refnum<class "State Machine.lvclass">)  [unwired: 7 in]
          n104 = call-dynamic "Write State Machine.vi"("error in (no error)"=w309, "State Machine.lvclass"=w307, "Device in"=w306) -> ("error out"=w303:errorcluster, "Device out"=w305:refnum<class "Channel.lvclass">)  [unwired: 7 in]
          n105 = Unbundle By Name(w305) -> ("Interface.lvclass"=w315:refnum<class "Interface.lvclass">)
          n106 = call-dynamic "Read ObsType.vi"("error in (no error)"=w303, "Interface in"=w315) -> ("error out"=w302:errorcluster, "ObsType"=w310:string)  [unwired: 7 in, 1 out]
          n107 = Concatenate Strings("SET OBSTYPE " ("cmd"), w310) -> (w314:string)
          n108 = call-dynamic "Write cmd.vi"("error in (no error)"=w302, "cmd"=w314, "Device in"=w305) -> ("error out"=w316:errorcluster, "Device out"=w317:refnum<class "Channel.lvclass">)  [unwired: 7 in]
          n109 = Increment(x=w312) -> (x+1=w313:i32)
        }
        frame 15 {
          n110 = call "Verify Timer.vi"("error in (no error)"=w326, "State Machine in"=w324) -> ("error out"=w325:errorcluster, "timeout"=w321:bool, "State Machine out"=w328:refnum<class "State Machine.lvclass">)  [unwired: 7 in]
          n111 = call-dynamic "Write State Machine.vi"("error in (no error)"=w325, "State Machine.lvclass"=w328, "Device in"=w327) -> ("error out"=w322:errorcluster, "Device out"=w323:refnum<class "Channel.lvclass">)  [unwired: 7 in]
          n112 = call-dynamic "Read resp.vi"("error in (no error)"=w322, "Device in"=w323) -> ("error out"=w329:errorcluster, "resp"=w332:string, "Device out"=w330:refnum<class "Channel.lvclass">)  [unwired: 7 in]
          n113 = Equal?(x=w332, y="DONE") -> (x = y?=w319:bool)
          n114 = case shown="False" w321 {
            tunnel: [w334 0] -> w318
            tunnel: w320 -> [w335 _]
            tunnel: w319 -> [w333 _]
            frame False {
              n115 = case shown="True" w333 {
                tunnel: w335 -> [w336 w338]
                tunnel: [w336 w337] -> w334
                frame False {
                }
                frame True {
                  n116 = Increment(x=w338) -> (x+1=w337:i32)
                }
              }
            }
            frame True {
            }
          }
        }
        frame 16 {
          # "observer"
          n117 = call-dynamic "Write Timer.vi"("error in (no error)"=w344, "Timer"=u32 50, "State Machine in"=w340) -> ("error out"=w349:errorcluster, "State Machine out"=w347:refnum<class "State Machine.lvclass">)  [unwired: 7 in]
          n118 = call-dynamic "Write State Machine.vi"("error in (no error)"=w349, "State Machine.lvclass"=w347, "Device in"=w346) -> ("error out"=w343:errorcluster, "Device out"=w345:refnum<class "Channel.lvclass">)  [unwired: 7 in]
          n119 = Unbundle By Name(w345) -> ("Interface.lvclass"=w354:refnum<class "Interface.lvclass">)
          n120 = call-dynamic "Read Observer.vi"("error in (no error)"=w343, "Interface in"=w354) -> ("error out"=w342:errorcluster, "Observer"=w350:string)  [unwired: 7 in, 1 out]
          n121 = Concatenate Strings("SET OBSERVER " ("cmd"), w350) -> (w353:string)
          n122 = call-dynamic "Write cmd.vi"("error in (no error)"=w342, "cmd"=w353, "Device in"=w345) -> ("error out"=w355:errorcluster, "Device out"=w356:refnum<class "Channel.lvclass">)  [unwired: 7 in]
          n123 = Increment(x=w351) -> (x+1=w352:i32)
        }
        frame 17 {
          n124 = call "Verify Timer.vi"("error in (no error)"=w365, "State Machine in"=w363) -> ("error out"=w364:errorcluster, "timeout"=w360:bool, "State Machine out"=w367:refnum<class "State Machine.lvclass">)  [unwired: 7 in]
          n125 = call-dynamic "Write State Machine.vi"("error in (no error)"=w364, "State Machine.lvclass"=w367, "Device in"=w366) -> ("error out"=w361:errorcluster, "Device out"=w362:refnum<class "Channel.lvclass">)  [unwired: 7 in]
          n126 = call-dynamic "Read resp.vi"("error in (no error)"=w361, "Device in"=w362) -> ("error out"=w368:errorcluster, "resp"=w371:string, "Device out"=w369:refnum<class "Channel.lvclass">)  [unwired: 7 in]
          n127 = Equal?(x=w371, y="DONE") -> (x = y?=w358:bool)
          n128 = case shown="False" w360 {
            tunnel: [w373 0] -> w357
            tunnel: w359 -> [w374 _]
            tunnel: w358 -> [w372 _]
            frame False {
              n129 = case shown="True" w372 {
                tunnel: w374 -> [w375 w377]
                tunnel: [w375 w376] -> w373
                frame False {
                }
                frame True {
                  n130 = Increment(x=w377) -> (x+1=w376:i32)
                }
              }
            }
            frame True {
            }
          }
        }
        frame 18 {
          # "comment"
          n131 = call-dynamic "Write Timer.vi"("error in (no error)"=w383, "Timer"=u32 50, "State Machine in"=w379) -> ("error out"=w388:errorcluster, "State Machine out"=w386:refnum<class "State Machine.lvclass">)  [unwired: 7 in]
          n132 = call-dynamic "Write State Machine.vi"("error in (no error)"=w388, "State Machine.lvclass"=w386, "Device in"=w385) -> ("error out"=w382:errorcluster, "Device out"=w384:refnum<class "Channel.lvclass">)  [unwired: 7 in]
          n133 = Unbundle By Name(w384) -> ("Interface.lvclass"=w393:refnum<class "Interface.lvclass">)
          n134 = call-dynamic "Read Comments.vi"("error in (no error)"=w382, "Interface in"=w393) -> ("error out"=w381:errorcluster, "Comments"=w389:string)  [unwired: 7 in, 1 out]
          n135 = Concatenate Strings("SET COMMENT " ("cmd"), w389) -> (w392:string)
          n136 = call-dynamic "Write cmd.vi"("error in (no error)"=w381, "cmd"=w392, "Device in"=w384) -> ("error out"=w394:errorcluster, "Device out"=w395:refnum<class "Channel.lvclass">)  [unwired: 7 in]
          n137 = Increment(x=w390) -> (x+1=w391:i32)
        }
        frame 19 {
          n138 = call "Verify Timer.vi"("error in (no error)"=w404, "State Machine in"=w402) -> ("error out"=w403:errorcluster, "timeout"=w399:bool, "State Machine out"=w406:refnum<class "State Machine.lvclass">)  [unwired: 7 in]
          n139 = call-dynamic "Write State Machine.vi"("error in (no error)"=w403, "State Machine.lvclass"=w406, "Device in"=w405) -> ("error out"=w400:errorcluster, "Device out"=w401:refnum<class "Channel.lvclass">)  [unwired: 7 in]
          n140 = call-dynamic "Read resp.vi"("error in (no error)"=w400, "Device in"=w401) -> ("error out"=w407:errorcluster, "resp"=w410:string, "Device out"=w408:refnum<class "Channel.lvclass">)  [unwired: 7 in]
          n141 = Equal?(x=w410, y="DONE") -> (x = y?=w397:bool)
          n142 = case shown="False" w399 {
            tunnel: [w412 0] -> w396
            tunnel: w398 -> [w413 _]
            tunnel: w397 -> [w411 _]
            frame False {
              n143 = case shown="True" w411 {
                tunnel: w413 -> [w414 w416]
                tunnel: [w414 w415] -> w412
                frame False {
                }
                frame True {
                  n144 = Increment(x=w416) -> (x+1=w415:i32)
                }
              }
            }
            frame True {
            }
          }
        }
        frame 20 {
          # "object"
          n145 = call-dynamic "Write Timer.vi"("error in (no error)"=w422, "Timer"=u32 50, "State Machine in"=w418) -> ("error out"=w427:errorcluster, "State Machine out"=w425:refnum<class "State Machine.lvclass">)  [unwired: 7 in]
          n146 = call-dynamic "Write State Machine.vi"("error in (no error)"=w427, "State Machine.lvclass"=w425, "Device in"=w424) -> ("error out"=w421:errorcluster, "Device out"=w423:refnum<class "Channel.lvclass">)  [unwired: 7 in]
          n147 = Unbundle By Name(w423) -> ("Interface.lvclass"=w432:refnum<class "Interface.lvclass">)
          n148 = call-dynamic "Read Object.vi"("error in (no error)"=w421, "Interface in"=w432) -> ("error out"=w420:errorcluster, "Object"=w428:string)  [unwired: 7 in, 1 out]
          n149 = Concatenate Strings("SET OBJECT " ("cmd"), w428) -> (w431:string)
          n150 = call-dynamic "Write cmd.vi"("error in (no error)"=w420, "cmd"=w431, "Device in"=w423) -> ("error out"=w433:errorcluster, "Device out"=w434:refnum<class "Channel.lvclass">)  [unwired: 7 in]
          n151 = Increment(x=w429) -> (x+1=w430:i32)
        }
        frame 21 {
          n152 = call "Verify Timer.vi"("error in (no error)"=w443, "State Machine in"=w441) -> ("error out"=w442:errorcluster, "timeout"=w438:bool, "State Machine out"=w445:refnum<class "State Machine.lvclass">)  [unwired: 7 in]
          n153 = call-dynamic "Write State Machine.vi"("error in (no error)"=w442, "State Machine.lvclass"=w445, "Device in"=w444) -> ("error out"=w439:errorcluster, "Device out"=w440:refnum<class "Channel.lvclass">)  [unwired: 7 in]
          n154 = call-dynamic "Read resp.vi"("error in (no error)"=w439, "Device in"=w440) -> ("error out"=w446:errorcluster, "resp"=w449:string, "Device out"=w447:refnum<class "Channel.lvclass">)  [unwired: 7 in]
          n155 = Equal?(x=w449, y="DONE") -> (x = y?=w436:bool)
          n156 = case shown="False" w438 {
            tunnel: [w451 0] -> w435
            tunnel: w437 -> [w452 _]
            tunnel: w436 -> [w450 _]
            frame False {
              n157 = case shown="True" w450 {
                tunnel: w452 -> [w453 w455]
                tunnel: [w453 w454] -> w451
                frame False {
                }
                frame True {
                  n158 = Increment(x=w455) -> (x+1=w454:i32)
                }
              }
            }
            frame True {
            }
          }
        }
        frame 22 {
          # "filter"
          n159 = call-dynamic "Write Timer.vi"("error in (no error)"=w462, "Timer"=u32 50, "State Machine in"=w460) -> ("error out"=w467:errorcluster, "State Machine out"=w465:refnum<class "State Machine.lvclass">)  [unwired: 7 in]
          n160 = call-dynamic "Write State Machine.vi"("error in (no error)"=w467, "State Machine.lvclass"=w465, "Device in"=w464) -> ("error out"=w457:errorcluster, "Device out"=w463:refnum<class "Channel.lvclass">)  [unwired: 7 in]
          n161 = Unbundle By Name(w463) -> ("Filter"=w459:u8)
          n162 = case shown="0, Default" w459 {
            tunnel: ["U" ("cmd") "B" ("cmd") "V" ("cmd") "R" ("cmd") "I" ("cmd") "CLEAR" ("cmd")] -> w458
            frame 1 {
            }
            frame 2 {
            }
            frame 3 {
            }
            frame 4 {
            }
            frame 5 {
            }
            frame 0, Default {
            }
          }
          n163 = Concatenate Strings("SET FILTER " ("cmd"), w458) -> (w470:string)
          n164 = call-dynamic "Write cmd.vi"("error in (no error)"=w457, "cmd"=w470, "Device in"=w463) -> ("error out"=w471:errorcluster, "Device out"=w472:refnum<class "Channel.lvclass">)  [unwired: 7 in]
          n165 = Increment(x=w468) -> (x+1=w469:i32)
        }
        frame 23 {
          n166 = call "Verify Timer.vi"("error in (no error)"=w487, "State Machine in"=w485) -> ("error out"=w486:errorcluster, "timeout"=w482:bool, "State Machine out"=w489:refnum<class "State Machine.lvclass">)  [unwired: 7 in]
          n167 = call-dynamic "Write State Machine.vi"("error in (no error)"=w486, "State Machine.lvclass"=w489, "Device in"=w488) -> ("error out"=w483:errorcluster, "Device out"=w484:refnum<class "Channel.lvclass">)  [unwired: 7 in]
          n168 = call-dynamic "Read resp.vi"("error in (no error)"=w483, "Device in"=w484) -> ("error out"=w490:errorcluster, "resp"=w493:string, "Device out"=w491:refnum<class "Channel.lvclass">)  [unwired: 7 in]
          n169 = Equal?(x=w493, y="DONE") -> (x = y?=w480:bool)
          n170 = case shown="False" w482 {
            tunnel: [w495 0] -> w479
            tunnel: w481 -> [w496 _]
            tunnel: w480 -> [w494 _]
            frame False {
              n171 = case shown="True" w494 {
                tunnel: w496 -> [w497 w499]
                tunnel: [w497 w498] -> w495
                frame False {
                }
                frame True {
                  n172 = Increment(x=w499) -> (x+1=w498:i32)
                }
              }
            }
            frame True {
            }
          }
        }
        frame 24 {
          n173 = call-dynamic "Write Timer.vi"("error in (no error)"=w504, "Timer"=u32 50, "State Machine in"=w503) -> ("error out"=w509:errorcluster, "State Machine out"=w507:refnum<class "State Machine.lvclass">)  [unwired: 7 in]
          n174 = call-dynamic "Write State Machine.vi"("error in (no error)"=w509, "State Machine.lvclass"=w507, "Device in"=w506) -> ("error out"=w502:errorcluster, "Device out"=w505:refnum<class "Channel.lvclass">)  [unwired: 7 in]
          n175 = call-dynamic "Write cmd.vi"("error in (no error)"=w502, "cmd"="SET CTRLINTE S4GUI", "Device in"=w505) -> ("error out"=w512:errorcluster, "Device out"=w513:refnum<class "Channel.lvclass">)  [unwired: 7 in]
          n176 = Increment(x=w510) -> (x+1=w511:i32)
        }
        frame 25 {
          n177 = call "Verify Timer.vi"("error in (no error)"=w522, "State Machine in"=w520) -> ("error out"=w521:errorcluster, "timeout"=w517:bool, "State Machine out"=w524:refnum<class "State Machine.lvclass">)  [unwired: 7 in]
          n178 = call-dynamic "Write State Machine.vi"("error in (no error)"=w521, "State Machine.lvclass"=w524, "Device in"=w523) -> ("error out"=w518:errorcluster, "Device out"=w519:refnum<class "Channel.lvclass">)  [unwired: 7 in]
          n179 = call-dynamic "Read resp.vi"("error in (no error)"=w518, "Device in"=w519) -> ("error out"=w525:errorcluster, "resp"=w528:string, "Device out"=w526:refnum<class "Channel.lvclass">)  [unwired: 7 in]
          n180 = Equal?(x=w528, y="DONE") -> (x = y?=w515:bool)
          n181 = case shown="False" w517 {
            tunnel: [w530 0] -> w514
            tunnel: w516 -> [w531 _]
            tunnel: w515 -> [w529 _]
            frame False {
              n182 = case shown="True" w529 {
                tunnel: w531 -> [w532 w534]
                tunnel: [w532 w533] -> w530
                frame False {
                }
                frame True {
                  n183 = Increment(x=w534) -> (x+1=w533:i32)
                }
              }
            }
            frame True {
            }
          }
        }
        frame 26 {
          # "Carrega timeout de 50 ciclos\npara resposta do ACS"
          n184 = call-dynamic "Write Timer.vi"("error in (no error)"=w544, "Timer"=u32 50, "State Machine in"=w543) -> ("error out"=w546:errorcluster, "State Machine out"=w548:refnum<class "State Machine.lvclass">)  [unwired: 7 in]
          n185 = call-dynamic "Write State Machine.vi"("error in (no error)"=w546, "State Machine.lvclass"=w548, "Device in"=w545) -> ("error out"=w538:errorcluster, "Device out"=w537:refnum<class "Channel.lvclass">)  [unwired: 7 in]
          n186 = Unbundle By Name(w537) -> ("rotator"=w536:dbl)
          n187 = Number To Fractional String(number=w536) -> (F-format string=w540:string)  [unwired: 3 in]
          n188 = Concatenate Strings("SET INSTROT " ("cmd"), w540) -> (w539:string)
          n189 = call-dynamic "Write cmd.vi"("error in (no error)"=w538, "cmd"=w539, "Device in"=w537) -> ("error out"=w550:errorcluster, "Device out"=w551:refnum<class "Channel.lvclass">)  [unwired: 7 in]
          n190 = Increment(x=w542) -> (x+1=w549:i32)
        }
        frame 27 {
          n191 = call "Verify Timer.vi"("error in (no error)"=w556, "State Machine in"=w557) -> ("error out"=w561:errorcluster, "timeout"=w553:bool, "State Machine out"=w562:refnum<class "State Machine.lvclass">)  [unwired: 7 in]
          n192 = call-dynamic "Write State Machine.vi"("error in (no error)"=w561, "State Machine.lvclass"=w562, "Device in"=w560) -> ("error out"=w558:errorcluster, "Device out"=w559:refnum<class "Channel.lvclass">)  [unwired: 7 in]
          n193 = call-dynamic "Read resp.vi"("error in (no error)"=w558, "Device in"=w559) -> ("error out"=w563:errorcluster, "resp"=w566:string, "Device out"=w564:refnum<class "Channel.lvclass">)  [unwired: 7 in]
          n194 = Equal?(x=w566, y="DONE") -> (x = y?=w552:bool)
          n195 = case shown="False" w553 {
            tunnel: [w568 0] -> w555
            tunnel: w554 -> [w569 _]
            tunnel: w552 -> [w567 _]
            frame False {
              n196 = case shown="True" w567 {
                tunnel: [w570 300 ("State")] -> w568
                tunnel: w569 -> [w570 _]
                frame False {
                }
                frame True {
                  # "continua a\nsequencia de\ncomandos SET\nem 300..."
                }
              }
            }
            frame True {
            }
          }
        }
        frame 29 {
          n197 = Unbundle By Name(w573) -> ("expose"=w575:bool)
          n198 = case shown="False" w575 {
            tunnel: [u8 0 ("State") u8 50 ("State")] -> w577
            tunnel: w576 -> [_ _]
            frame False {
            }
            frame True {
            }
          }
        }
        frame 30 {
          n199 = call-dynamic "Write Timer.vi"("error in (no error)"=w584, "Timer"=u32 50, "State Machine in"=w586) -> ("error out"=w583:errorcluster, "State Machine out"=w585:refnum<class "State Machine.lvclass">)  [unwired: 7 in]
          n200 = call-dynamic "Write State Machine.vi"("error in (no error)"=w583, "State Machine.lvclass"=w585, "Device in"=w587) -> ("error out"=w581:errorcluster, "Device out"=w582:refnum<class "Channel.lvclass">)  [unwired: 7 in]
          n201 = Unbundle By Name(w582) -> ("Interface.lvclass"=w595:refnum<class "Interface.lvclass">)
          n202 = call-dynamic "Read Cooler ON_OFF.vi"("error in (no error)"=w581, "Interface in"=w595) -> ("error out"=w580:errorcluster, "Cooler ON/OFF"=w590:i16)  [unwired: 7 in, 1 out]
          n203 = case shown="0" w590 {
            tunnel: ["1" "0"] -> w589
            frame 0 {
              (unwired) "ON"
              # "Se COOLER desligado, manda ligar."
            }
            frame 1, Default {
              (unwired) "OFF"
              # "Se COOLER ligado, manda desligar."
            }
          }
          n204 = Concatenate Strings("SET COOLER_POWER_STATUS " ("cmd"), w589) -> (w594:string)
          n205 = call-dynamic "Write cmd.vi"("error in (no error)"=w580, "cmd"=w594, "Device in"=w582) -> ("error out"=w596:errorcluster, "Device out"=w597:refnum<class "Channel.lvclass">)  [unwired: 7 in]
          n206 = Increment(x=w592) -> (x+1=w593:i32)
        }
        frame 31 {
          n207 = call "Verify Timer.vi"("error in (no error)"=w607, "State Machine in"=w604) -> ("error out"=w602:errorcluster, "timeout"=w600:bool, "State Machine out"=w603:refnum<class "State Machine.lvclass">)  [unwired: 7 in]
          n208 = call-dynamic "Write State Machine.vi"("error in (no error)"=w602, "State Machine.lvclass"=w603, "Device in"=w606) -> ("error out"=w601:errorcluster, "Device out"=w605:refnum<class "Channel.lvclass">)  [unwired: 7 in]
          n209 = call-dynamic "Read resp.vi"("error in (no error)"=w601, "Device in"=w605) -> ("error out"=w609:errorcluster, "resp"=w614:string, "Device out"=w610:refnum<class "Channel.lvclass">)  [unwired: 7 in]
          n210 = Equal?(x=w614, y="DONE") -> (x = y?=w612:bool)
          n211 = case shown="False" w600 {
            tunnel: w612 -> [w617 _]
            tunnel: [w616 w621] -> w611
            tunnel: w608 -> [w615 _]
            frame False {
              n212 = case shown="True" w617 {
                tunnel: [w618 w619] -> w616
                tunnel: w615 -> [w618 w620]
                frame False {
                }
                frame True {
                  n213 = Increment(x=w620) -> (x+1=w619:i32)
                }
              }
            }
            frame True {
              n214 = disable-structure shown="Enabled" {
                disable-tunnel: [0 ("State") 12 ("State")] -> w621
                frame Disabled {
                }
                frame Enabled {
                  # "12: configura os\nparametros por comando\nSET"
                }
              }
            }
          }
        }
        frame 32 {
          n215 = call-dynamic "Write Timer.vi"("error in (no error)"=w628, "Timer"=u32 50, "State Machine in"=w629) -> ("error out"=w631:errorcluster, "State Machine out"=w626:refnum<class "State Machine.lvclass">)  [unwired: 7 in]
          n216 = call-dynamic "Write State Machine.vi"("error in (no error)"=w631, "State Machine.lvclass"=w626, "Device in"=w630) -> ("error out"=w624:errorcluster, "Device out"=w625:refnum<class "Channel.lvclass">)  [unwired: 7 in]
          n217 = call-dynamic "Write cmd.vi"("error in (no error)"=w624, "cmd"="GET COOLER_POWER_STATUS ", "Device in"=w625) -> ("error out"=w635:errorcluster, "Device out"=w636:refnum<class "Channel.lvclass">)  [unwired: 7 in]
          n218 = Increment(x=w633) -> (x+1=w634:i32)
        }
        frame 33 {
          n219 = call "Verify Timer.vi"("error in (no error)"=w640, "State Machine in"=w644) -> ("error out"=w639:errorcluster, "timeout"=w638:bool, "State Machine out"=w641:refnum<class "State Machine.lvclass">)  [unwired: 7 in]
          n220 = call-dynamic "Write State Machine.vi"("error in (no error)"=w639, "State Machine.lvclass"=w641, "Device in"=w643) -> ("error out"=w637:errorcluster, "Device out"=w642:refnum<class "Channel.lvclass">)  [unwired: 7 in]
          n221 = call-dynamic "Read resp.vi"("error in (no error)"=w637, "Device in"=w642) -> ("error out"=w649:errorcluster, "resp"=w645:string, "Device out"=w650:refnum<class "Channel.lvclass">)  [unwired: 7 in]
          n222 = case shown="True" w638 {
            tunnel: [w658 w679] -> w651
            tunnel: w650 -> [w657 w679]
            tunnel: w649 -> [w656 w678]
            tunnel: [w655 w678] -> w648
            tunnel: [w654 w677] -> w647
            tunnel: w646 -> [w653 _]
            tunnel: w645 -> [w652 _]
            frame False {
              n223 = case shown="Default" w652 {
                selector: w652 -> [_ w670]
                tunnel: [w661 w666] -> w658
                tunnel: w657 -> [w661 w674]
                tunnel: w656 -> [w660 w672]
                tunnel: [w660 w664] -> w655
                tunnel: [w659 w671] -> w654
                tunnel: w653 -> [w659 _]
                frame Default {
                }
                frame "0", "1" {
                  n224 = Decimal String To Number(string=w670) -> (number=w669:i32)  [unwired: 2 in, 1 out]
                  n225 = Unbundle By Name(w674) -> ("Interface.lvclass"=w673:refnum<class "Interface.lvclass">)
                  n226 = To Word Integer(number=w669) -> (16bit integer=w668:i16)
                  n227 = call-dynamic "Write Cooler ON_OFF.vi"("error in (no error)"=w672, "Cooler ON/OFF"=w668, "Interface in"=w673) -> ("error out"=w665:errorcluster, "Interface out"=w663:refnum<class "Interface.lvclass">)  [unwired: 7 in]
                  n228 = Bundle By Name(cluster=w674, "Interface.lvclass"=w663) -> (w667:refnum<class "Channel.lvclass">)
                  n229 = disable-structure shown="Enabled" {
                    disable-tunnel: [0 ("State") 12 ("State")] -> w671
                    frame Disabled {
                    }
                    frame Enabled {
                      # "12: configura os\nparametros por comando\nSET"
                    }
                  }
                  n230 = call-dynamic "Save Temp.vi"("error in (no error)"=w665, "temp file"="lasttemp.cfg", "Channel in"=w667) -> ("error out"=w664:errorcluster, "Channel out"=w666:refnum<class "Channel.lvclass">)  [unwired: 7 in]
                }
              }
            }
            frame True {
              n231 = disable-structure shown="Enabled" {
                disable-tunnel: [0 ("State") 12 ("State")] -> w677
                frame Disabled {
                }
                frame Enabled {
                  # "12: configura os\nparametros por comando\nSET"
                }
              }
            }
          }
        }
        frame 35 {
          n232 = Unbundle By Name(w690) -> ("Interface.lvclass"=w689:refnum<class "Interface.lvclass">)
          n233 = call-dynamic "Read Temperature.vi"("Interface in"=w689) -> ("Temperature"=w686:i8)  [unwired: 8 in, 2 out]
          n234 = Number To Decimal String(number=w686) -> (decimal integer string=w685:string)  [unwired: 1 in]
          n235 = Concatenate Strings("SET TEMP " ("cmd"), w685) -> (w688:string)
          n236 = call-dynamic "Write cmd.vi"("error in (no error)"=w692, "cmd"=w688, "Device in"=w690) -> ("error out"=w691:errorcluster, "Device out"=w683:refnum<class "Channel.lvclass">)  [unwired: 7 in]
          n237 = Increment(x=w682) -> (x+1=w684:i32)
        }
        frame 36 {
          n238 = call "Verify Timer.vi"("error in (no error)"=w700, "State Machine in"=w697) -> ("error out"=w695:errorcluster, "timeout"=w693:bool, "State Machine out"=w696:refnum<class "State Machine.lvclass">)  [unwired: 7 in]
          n239 = call-dynamic "Write State Machine.vi"("error in (no error)"=w695, "State Machine.lvclass"=w696, "Device in"=w699) -> ("error out"=w694:errorcluster, "Device out"=w698:refnum<class "Channel.lvclass">)  [unwired: 7 in]
          n240 = call-dynamic "Read resp.vi"("error in (no error)"=w694, "Device in"=w698) -> ("error out"=w702:errorcluster, "resp"=w707:string, "Device out"=w703:refnum<class "Channel.lvclass">)  [unwired: 7 in]
          n241 = Equal?(x=w707, y="DONE") -> (x = y?=w705:bool)
          n242 = case shown="False" w693 {
            tunnel: w705 -> [w710 _]
            tunnel: [w709 w714] -> w704
            tunnel: w701 -> [w708 _]
            frame False {
              n243 = case shown="False" w710 {
                tunnel: [w711 w712] -> w709
                tunnel: w708 -> [w711 w713]
                frame False {
                }
                frame True {
                  # "OV 2022-11-16: Ao setar a temperatura, liga \nautomaticamente o COLLER."
                  n244 = Increment(x=w713) -> (x+1=w712:i32)
                }
              }
            }
            frame True {
              n245 = disable-structure shown="Enabled" {
                disable-tunnel: [0 ("State") 12 ("State")] -> w714
                frame Disabled {
                }
                frame Enabled {
                  # "12: configura os\nparametros por comando\nSET"
                }
              }
            }
          }
        }
        frame 37 {
          # "Liga COOLER"
          n246 = call-dynamic "Write Timer.vi"("error in (no error)"=w722, "Timer"=u32 50, "State Machine in"=w724) -> ("error out"=w721:errorcluster, "State Machine out"=w723:refnum<class "State Machine.lvclass">)  [unwired: 7 in]
          n247 = call-dynamic "Write State Machine.vi"("error in (no error)"=w721, "State Machine.lvclass"=w723, "Device in"=w725) -> ("error out"=w719:errorcluster, "Device out"=w718:refnum<class "Channel.lvclass">)  [unwired: 7 in]
          n248 = call-dynamic "Write cmd.vi"("error in (no error)"=w719, "cmd"="SET COOLER_POWER_STATUS 1", "Device in"=w718) -> ("error out"=w727:errorcluster, "Device out"=w728:refnum<class "Channel.lvclass">)  [unwired: 7 in]
        }
        frame 40 {
          n249 = disable-structure shown="Enabled" {
            disable-tunnel: [w749 w751] -> w742
            disable-tunnel: w741 -> [w747 w751]
            disable-tunnel: w739 -> [w746 w750]
            disable-tunnel: [w745 w750] -> w738
            frame Disabled {
              # "Carrega timeout de 10 ciclos\npara resposta do ACS"
              n250 = call-dynamic "Write Timer.vi"("error in (no error)"=w746, "Timer"=u32 10, "State Machine in"=w747) -> ("error out"=w745:errorcluster, "State Machine out"=w749:refnum<class "State Machine.lvclass">)  [unwired: 7 in]
            }
            frame Enabled {
            }
          }
          n251 = call-dynamic "Write State Machine.vi"("error in (no error)"=w738, "State Machine.lvclass"=w742, "Device in"=w740) -> ("error out"=w737:errorcluster, "Device out"=w734:refnum<class "Channel.lvclass">)  [unwired: 7 in]
          n252 = Unbundle By Name(w734) -> ("wait_expose"=w733:bool)
          n253 = Select(t="ON", s=w733, f="OFF") -> (s? t:f=w730:string)
          n254 = Concatenate Strings("WAIT_EXPOSE_COMMAND " ("cmd"), w730) -> (w729:string)
          n255 = call-dynamic "Write cmd.vi"("error in (no error)"=w737, "cmd"=w729, "Device in"=w734) -> ("error out"=w743:errorcluster, "Device out"=w744:refnum<class "Channel.lvclass">)  [unwired: 7 in]
        }
        frame 50 {
          (unwired) "S4ACS C1/C2/C3/C4 EXPOSE " ("cmd")
          # "OV 2023-05-18:\nVai direto para o pedido\nde STATUS (sem a pausa \nde 10 ciclos)"
          # "Carrega timeout de 10 ciclos\npara resposta do ACS"
          n256 = call-dynamic "Write Timer.vi"("error in (no error)"=w756, "Timer"=u32 10, "State Machine in"=w759) -> ("error out"=w755:errorcluster, "State Machine out"=w761:refnum<class "State Machine.lvclass">)  [unwired: 7 in]
          n257 = call-dynamic "Write State Machine.vi"("error in (no error)"=w755, "State Machine.lvclass"=w761, "Device in"=w758) -> ("error out"=w754:errorcluster, "Device out"=w757:refnum<class "Channel.lvclass">)  [unwired: 7 in]
          n258 = call-dynamic "Write cmd.vi"("error in (no error)"=w754, "cmd"="EXPOSE", "Device in"=w757) -> ("error out"=w764:errorcluster, "Device out"=w765:refnum<class "Channel.lvclass">)  [unwired: 7 in]
          n259 = Increment(x=w763) -> (x+1=w753:i32)
          n260 = Increment(x=w753) -> (x+1=w752:i32)
        }
        frame 51 {
          # "Verifica timeout para ACS responder.\nSe estourar timeout é porque o ACS não \nrespondeu e este canal volta para o estado 0\npara não \"travar\" os outros canais no \nS4ACS_GUI:HandleObservation.vi."
          n261 = call "Verify Timer.vi"("error in (no error)"=w770, "State Machine in"=w772) -> ("error out"=w769:errorcluster, "timeout"=w768:bool, "State Machine out"=w771:refnum<class "State Machine.lvclass">)  [unwired: 7 in]
          n262 = call-dynamic "Write State Machine.vi"("error in (no error)"=w769, "State Machine.lvclass"=w771, "Device in"=w773) -> ("error out"=w766:errorcluster, "Device out"=w767:refnum<class "Channel.lvclass">)  [unwired: 7 in]
          n263 = case shown="True" w768 {
            tunnel: [w776 w777] -> w775
            tunnel: w774 -> [w776 w778]
            frame False {
            }
            frame True {
              n264 = Increment(x=w778) -> (x+1=w777:i32)
            }
          }
        }
        frame 52 {
          (unwired) "S4ACS C1/C2/C3/C4 STATUS " ("cmd")
          # "Carrega timeout de 200 ciclos\npara resposta do ACS"
          n265 = call-dynamic "Write Timer.vi"("error in (no error)"=w782, "Timer"=u32 200, "State Machine in"=w783) -> ("error out"=w785:errorcluster, "State Machine out"=w786:refnum<class "State Machine.lvclass">)  [unwired: 7 in]
          n266 = call-dynamic "Write State Machine.vi"("error in (no error)"=w785, "State Machine.lvclass"=w786, "Device in"=w784) -> ("error out"=w781:errorcluster, "Device out"=w779:refnum<class "Channel.lvclass">)  [unwired: 7 in]
          n267 = call-dynamic "Write cmd.vi"("error in (no error)"=w781, "cmd"="STATUS", "Device in"=w779) -> ("error out"=w790:errorcluster, "Device out"=w791:refnum<class "Channel.lvclass">)  [unwired: 7 in]
          n268 = Increment(x=w788) -> (x+1=w789:i32)
        }
        frame 53 {
          # "Status.Texp = Current frame exptime\nlastStatus = cam status (acquiring, idle, writing, reading, ...)\nStatus.Nimages = frames done\nStatus.CubesDone = ciclos realizados pelo ACS\nStatus.SequesDone = sequencias realizadas pelo ACS."
          # "Verifica timeout para ACS responder.\nSe estourar timeout é porque o ACS não \nrespondeu e este canal volta para o estado 0\npara não \"travar\" os outros canais no \nS4ACS_GUI:HandleObservation.vi."
          # "Extrair todos os parametros da respsota de STATUS e\natualizar a informação na classe Channel."
          n269 = call "Verify Timer.vi"("error in (no error)"=w800, "State Machine in"=w805) -> ("error out"=w806:errorcluster, "timeout"=w804:bool, "State Machine out"=w807:refnum<class "State Machine.lvclass">)  [unwired: 7 in]
          n270 = call-dynamic "Write State Machine.vi"("error in (no error)"=w806, "State Machine.lvclass"=w807, "Device in"=w803) -> ("error out"=w801:errorcluster, "Device out"=w802:refnum<class "Channel.lvclass">)  [unwired: 7 in]
          n271 = call-dynamic "Read resp.vi"("error in (no error)"=w801, "Device in"=w802) -> ("error out"=w827:errorcluster, "resp"=w828:string, "Device out"=w831:refnum<class "Channel.lvclass">)  [unwired: 7 in]
          "resposta do STATUS" <- w828
          n272 = call-dynamic "Read Interface.vi"("error in (no error)"=w827, "Channel in"=w831) -> ("error out"=w826:errorcluster, "Interface.lvclass"=w829:refnum<class "Interface.lvclass">, "Channel out"=w830:refnum<class "Channel.lvclass">)  [unwired: 7 in]
          n273 = call-dynamic "UpdateStatus.vi"("error in (no error)"=w826, "status"=w828, "Interface in"=w829) -> ("error out"=w813:errorcluster, "Interface out"=w816:refnum<class "Interface.lvclass">)  [unwired: 7 in]
          n274 = call-dynamic "Read Exposições realizadas.vi"("error in (no error)"=w813, "Interface in"=w816) -> ("error out"=w812:errorcluster, "Exposições realizadas"=w814:dbl, "Interface out"=w815:refnum<class "Interface.lvclass">)  [unwired: 7 in]
          n275 = call-dynamic "Read Cam_Status.vi"("error in (no error)"=w812, "Interface in"=w815) -> ("error out"=w822:errorcluster, "Cam_Status"=w808:string, "Interface out"=w823:refnum<class "Interface.lvclass">)  [unwired: 7 in]
          n276 = call-dynamic "Read %Acquired.vi"("error in (no error)"=w822, "Interface in"=w823) -> ("error out"=w798:errorcluster, "% Acquired"=w819:dbl, "Interface out"=w799:refnum<class "Interface.lvclass">)  [unwired: 7 in]
          n277 = call-dynamic "Read Number of Cycles.vi"("error in (no error)"=w798, "Interface in"=w799) -> ("error out"=w794:errorcluster, "Number of Cycles"=w797:u32, "Interface out"=w796:refnum<class "Interface.lvclass">)  [unwired: 7 in]
          n278 = call-dynamic "Read Number of Sequences.vi"("error in (no error)"=w794, "Interface in"=w796) -> ("error out"=w793:errorcluster, "Number of Sequences"=w792:u32, "Interface out"=w795:refnum<class "Interface.lvclass">)  [unwired: 7 in]
          n279 = call "Read Exposure Time.vi"("error in (no error)"=w793, "Interface in"=w795) -> ("error out"=w810:errorcluster, "Exposure Time"=w821:dbl, "Interface out"=w809:refnum<class "Interface.lvclass">)  [unwired: 7 in]
          n280 = call-dynamic "Write Interface.vi"("error in (no error)"=w810, "Interface.lvclass"=w809, "Channel in"=w830) -> ("error out"=w825:errorcluster, "Channel out"=w824:refnum<class "Channel.lvclass">)  [unwired: 7 in]
          n281 = case shown="Default" w808 {
            tunnel: [w835 w838] -> w834
            tunnel: w833 -> [w836 w839]
            tunnel: w804 -> [_ w837]
            frame "ACTIVE", "WAITING EXPOSE COMMAND" {
              n282 = Increment(x=w836) -> (x+1=w835:i32)
            }
            frame Default {
              n283 = case shown="True" w837 {
                tunnel: w839 -> [w840 _]
                tunnel: [w840 0] -> w838
                frame False {
                }
                frame True {
                }
              }
            }
          }
          n284 = To Unsigned Long Integer(number=w814) -> (unsigned 32bit integer=w811:u32)
          n285 = Divide(x=w819, y=100.0) -> (x/y=w817:dbl)
          n286 = Multiply(x=w821, y=w817) -> (x*y=w820:dbl)
          n287 = Bundle By Name(cluster=w824, "Texp"=w820, "lastStatus"=w808, "Nimages"=w811, "CyclesDone"=w797, "SequesDone"=w792) -> (w832:refnum<class "Channel.lvclass">)
        }
        frame 54 {
          # "Verifica o timeout de 5s para enviar\ntelemetria para o ACS."
          n288 = call-dynamic "Verif Clock.vi"("error in (no error)"=w847, "period"=u32 5000, "State Machine in"=w848) -> ("error out"=w845:errorcluster, "State Machine out"=w846:refnum<class "State Machine.lvclass">)  [unwired: 7 in]
          n289 = call-dynamic "Read Timeout.vi"("error in (no error)"=w845, "State Machine in"=w846) -> ("error out"=w842:errorcluster, "Timeout"=w844:bool, "State Machine out"=w843:refnum<class "State Machine.lvclass">)  [unwired: 7 in]
          n290 = case shown="True" w844 {
            tunnel: [w867 w870] -> w854
            tunnel: [w866 w868] -> w853
            tunnel: [w865 59] -> w852
            tunnel: w851 -> [w864 _]
            tunnel: w850 -> [w861 w872]
            tunnel: w843 -> [w858 w871]
            tunnel: w842 -> [w857 w869]
            frame False {
              # "Carrega timeout de 10 ciclos x 20ms = 200ms\npara resposta do ACS"
              n291 = call-dynamic "Write Timer.vi"("error in (no error)"=w857, "Timer"=u32 10, "State Machine in"=w858) -> ("error out"=w855:errorcluster, "State Machine out"=w856:refnum<class "State Machine.lvclass">)  [unwired: 7 in]
              n292 = call-dynamic "Write State Machine.vi"("error in (no error)"=w855, "State Machine.lvclass"=w856, "Device in"=w861) -> ("error out"=w859:errorcluster, "Device out"=w860:refnum<class "Channel.lvclass">)  [unwired: 7 in]
              n293 = call-dynamic "Write cmd.vi"("error in (no error)"=w859, "cmd"="STATUS", "Device in"=w860) -> ("error out"=w866:errorcluster, "Device out"=w867:refnum<class "Channel.lvclass">)  [unwired: 7 in]
              n294 = Increment(x=w864) -> (x+1=w865:i32)
            }
            frame True {
              # "Estourou timeout de 5s:\nDesvia para enviar dados de \nTELEMETRIA a cada 5s (estado 59)"
              n295 = call-dynamic "Write State Machine.vi"("error in (no error)"=w869, "State Machine.lvclass"=w871, "Device in"=w872) -> ("error out"=w868:errorcluster, "Device out"=w870:refnum<class "Channel.lvclass">)  [unwired: 7 in]
            }
          }
        }
        frame 55 {
          # "Status.Texp = Current frame exptime\nlastStatus = cam status (acquiring, idle, writing, reading, ...)\nStatus.Nimages = frames done\nStatus.CubesDone = ciclos realizados pelo ACS\nStatus.SequesDone = sequencias realizadas pelo ACS."
          # "Extrair todos os parametros da respsota de STATUS e\natualizar a informação na classe Channel."
          n296 = call "Verify Timer.vi"("error in (no error)"=w887, "State Machine in"=w886) -> ("error out"=w883:errorcluster, "timeout"=w882:bool, "State Machine out"=w884:refnum<class "State Machine.lvclass">)  [unwired: 7 in]
          n297 = call-dynamic "Read resp.vi"("error in (no error)"=w883, "Device in"=w885) -> ("error out"=w909:errorcluster, "resp"=w910:string, "Device out"=w913:refnum<class "Channel.lvclass">)  [unwired: 7 in]
          n298 = call-dynamic "Read Interface.vi"("error in (no error)"=w909, "Channel in"=w913) -> ("error out"=w908:errorcluster, "Interface.lvclass"=w911:refnum<class "Interface.lvclass">, "Channel out"=w912:refnum<class "Channel.lvclass">)  [unwired: 7 in]
          n299 = call-dynamic "UpdateStatus.vi"("error in (no error)"=w908, "status"=w910, "Interface in"=w911) -> ("error out"=w895:errorcluster, "Interface out"=w898:refnum<class "Interface.lvclass">)  [unwired: 7 in]
          n300 = call-dynamic "Read Exposições realizadas.vi"("error in (no error)"=w895, "Interface in"=w898) -> ("error out"=w894:errorcluster, "Exposições realizadas"=w896:dbl, "Interface out"=w897:refnum<class "Interface.lvclass">)  [unwired: 7 in]
          n301 = call-dynamic "Read Cam_Status.vi"("error in (no error)"=w894, "Interface in"=w897) -> ("error out"=w905:errorcluster, "Cam_Status"=w892:string, "Interface out"=w907:refnum<class "Interface.lvclass">)  [unwired: 7 in]
          n302 = call-dynamic "Read %Acquired.vi"("error in (no error)"=w905, "Interface in"=w907) -> ("error out"=w904:errorcluster, "% Acquired"=w901:dbl, "Interface out"=w906:refnum<class "Interface.lvclass">)  [unwired: 7 in]
          n303 = call "Read Exposure Time.vi"("error in (no error)"=w904, "Interface in"=w906) -> ("error out"=w880:errorcluster, "Exposure Time"=w903:dbl, "Interface out"=w881:refnum<class "Interface.lvclass">)  [unwired: 7 in]
          n304 = call-dynamic "Read Number of Cycles.vi"("error in (no error)"=w880, "Interface in"=w881) -> ("error out"=w877:errorcluster, "Number of Cycles"=w879:u32, "Interface out"=w878:refnum<class "Interface.lvclass">)  [unwired: 7 in]
          n305 = call-dynamic "Read Number of Sequences.vi"("error in (no error)"=w877, "Interface in"=w878) -> ("error out"=w876:errorcluster, "Number of Sequences"=w874:u32, "Interface out"=w875:refnum<class "Interface.lvclass">)  [unwired: 7 in]
          n306 = call-dynamic "Write Interface.vi"("error in (no error)"=w876, "Interface.lvclass"=w875, "Channel in"=w912) -> ("error out"=w891:errorcluster, "Channel out"=w890:refnum<class "Channel.lvclass">)  [unwired: 7 in]
          n307 = case shown="\"ACQUISITION ABORTED\", \"IDLE\"" w892 {
            tunnel: [32 ("State") w932 w946] -> w916
            tunnel: w915 -> [_ w933 w947]
            tunnel: w891 -> [w923 w928 w944]
            tunnel: [w920 w930 w941] -> w889
            tunnel: w890 -> [w921 w931 w945]
            tunnel: [w917 w927 w938] -> w888
            tunnel: w884 -> [w924 w929 w943]
            tunnel: w882 -> [_ w926 w937]
            frame "ACQUISITION ABORTED", "IDLE" {
              # "250x20ms=5s"
              n308 = call-dynamic "Write Timer.vi"("error in (no error)"=w923, "Timer"=u32 250, "State Machine in"=w924) -> ("error out"=w918:errorcluster, "State Machine out"=w919:refnum<class "State Machine.lvclass">)  [unwired: 7 in]
              n309 = call-dynamic "Write State Machine.vi"("error in (no error)"=w918, "State Machine.lvclass"=w919, "Device in"=w921) -> ("error out"=w917:errorcluster, "Device out"=w920:refnum<class "Channel.lvclass">)  [unwired: 7 in]
            }
            frame Default {
              # "STATUS DETECTOR = ACTIVE or WAITING EXPOSE COMMAND"
              n310 = case shown="True" w926 {
                tunnel: w933 -> [w934 w936]
                tunnel: [w934 w935] -> w932
                frame False {
                }
                frame True {
                  n311 = Decrement(x=w936) -> (x-1=w935:i32)
                }
              }
              n312 = call-dynamic "Write State Machine.vi"("error in (no error)"=w928, "State Machine.lvclass"=w929, "Device in"=w931) -> ("error out"=w927:errorcluster, "Device out"=w930:refnum<class "Channel.lvclass">)  [unwired: 7 in]
            }
            frame "" {
              # "STATUS=\"\"\nACS parado"
              n313 = case shown="False" w937 {
                tunnel: w947 -> [w948 _]
                tunnel: [w948 0] -> w946
                tunnel: w945 -> [w951 w954]
                tunnel: [w951 w954] -> w942
                tunnel: w944 -> [w950 w955]
                tunnel: [w950 w952] -> w939
                tunnel: w943 -> [w949 w957]
                tunnel: [w949 w953] -> w940
                frame False {
                }
                frame True {
                  n314 = call-dynamic "Write Timer.vi"("error in (no error)"=w955, "Timer"=u32 250, "State Machine in"=w957) -> ("error out"=w952:errorcluster, "State Machine out"=w953:refnum<class "State Machine.lvclass">)  [unwired: 7 in]
                }
              }
              n315 = call-dynamic "Write State Machine.vi"("error in (no error)"=w939, "State Machine.lvclass"=w940, "Device in"=w942) -> ("error out"=w938:errorcluster, "Device out"=w941:refnum<class "Channel.lvclass">)  [unwired: 7 in]
            }
          }
          n316 = To Unsigned Long Integer(number=w896) -> (unsigned 32bit integer=w893:u32)
          n317 = Divide(x=w901, y=100.0) -> (x/y=w899:dbl)
          n318 = Multiply(x=w903, y=w899) -> (x*y=w902:dbl)
          n319 = Bundle By Name(cluster=w889, "Texp"=w902, "lastStatus"=w892, "Nimages"=w893, "CyclesDone"=w879, "SequesDone"=w874) -> (w914:refnum<class "Channel.lvclass">)
        }
        frame 56 {
          # "Pedido de STATUS para verificar conexão com ACS"
          # "Carrega timeout de 10 ciclos \n(20 x 20ms = 0.4s) \npara resposta do ACS"
          n320 = call-dynamic "Write Timer.vi"("error in (no error)"=w965, "Timer"=u32 20, "State Machine in"=w969) -> ("error out"=w970:errorcluster, "State Machine out"=w971:refnum<class "State Machine.lvclass">)  [unwired: 7 in]
          n321 = call-dynamic "Write State Machine.vi"("error in (no error)"=w970, "State Machine.lvclass"=w971, "Device in"=w967) -> ("error out"=w964:errorcluster, "Device out"=w966:refnum<class "Channel.lvclass">)  [unwired: 7 in]
          n322 = call-dynamic "Write cmd.vi"("error in (no error)"=w964, "cmd"="STATUS", "Device in"=w966) -> ("error out"=w962:errorcluster, "Device out"=w963:refnum<class "Channel.lvclass">)  [unwired: 7 in]
          n323 = Increment(x=w973) -> (x+1=w974:i32)
          n324 = call "Write connected.vi"("error in (no error)"=w962, "connected"=FALSE, "Device in"=w963) -> ("error out"=w960:errorcluster, "Device out"=w961:refnum<class "Channel.lvclass">)  [unwired: 7 in]
        }
        frame 57 {
          # "Status.Texp = Current frame exptime\nlastStatus = cam status (acquiring, idle, writing, reading, ...)\nStatus.Nimages = frames done\nStatus.CubesDone = ciclos realizados pelo ACS\nStatus.SequesDone = sequencias realizadas pelo ACS."
          # "Extrair todos os parametros da respsota de STATUS e\natualizar a informação na classe Channel."
          n325 = call "Verify Timer.vi"("error in (no error)"=w993, "State Machine in"=w992) -> ("error out"=w989:errorcluster, "State Machine out"=w991:refnum<class "State Machine.lvclass">)  [unwired: 7 in, 1 out]
          n326 = call-dynamic "Read Timeout.vi"("error in (no error)"=w989, "State Machine in"=w991) -> ("error out"=w984:errorcluster, "Timeout"=w988:bool, "State Machine out"=w990:refnum<class "State Machine.lvclass">)  [unwired: 7 in]
          n327 = call "Read connected.vi"("error in (no error)"=w984, "Device in"=w987) -> ("error out"=w985:errorcluster, "connected"=w983:bool, "Device out"=w986:refnum<class "Channel.lvclass">)  [unwired: 7 in]
          n328 = call-dynamic "Read resp.vi"("error in (no error)"=w985, "Device in"=w986) -> ("error out"=w1015:errorcluster, "resp"=w1016:string, "Device out"=w1019:refnum<class "Channel.lvclass">)  [unwired: 7 in]
          n329 = call-dynamic "Read Interface.vi"("error in (no error)"=w1015, "Channel in"=w1019) -> ("error out"=w1014:errorcluster, "Interface.lvclass"=w1017:refnum<class "Interface.lvclass">, "Channel out"=w1018:refnum<class "Channel.lvclass">)  [unwired: 7 in]
          n330 = call-dynamic "UpdateStatus.vi"("error in (no error)"=w1014, "status"=w1016, "Interface in"=w1017) -> ("error out"=w1001:errorcluster, "Interface out"=w1004:refnum<class "Interface.lvclass">)  [unwired: 7 in]
          n331 = call-dynamic "Read Exposições realizadas.vi"("error in (no error)"=w1001, "Interface in"=w1004) -> ("error out"=w1000:errorcluster, "Exposições realizadas"=w1002:dbl, "Interface out"=w1003:refnum<class "Interface.lvclass">)  [unwired: 7 in]
          n332 = call-dynamic "Read Cam_Status.vi"("error in (no error)"=w1000, "Interface in"=w1003) -> ("error out"=w1011:errorcluster, "Cam_Status"=w998:string, "Interface out"=w1013:refnum<class "Interface.lvclass">)  [unwired: 7 in]
          n333 = call-dynamic "Read %Acquired.vi"("error in (no error)"=w1011, "Interface in"=w1013) -> ("error out"=w1010:errorcluster, "% Acquired"=w1007:dbl, "Interface out"=w1012:refnum<class "Interface.lvclass">)  [unwired: 7 in]
          n334 = call "Read Exposure Time.vi"("error in (no error)"=w1010, "Interface in"=w1012) -> ("error out"=w981:errorcluster, "Exposure Time"=w1009:dbl, "Interface out"=w982:refnum<class "Interface.lvclass">)  [unwired: 7 in]
          n335 = call-dynamic "Read Number of Cycles.vi"("error in (no error)"=w981, "Interface in"=w982) -> ("error out"=w977:errorcluster, "Number of Cycles"=w980:u32, "Interface out"=w979:refnum<class "Interface.lvclass">)  [unwired: 7 in]
          n336 = call-dynamic "Read Number of Sequences.vi"("error in (no error)"=w977, "Interface in"=w979) -> ("error out"=w976:errorcluster, "Number of Sequences"=w975:u32, "Interface out"=w978:refnum<class "Interface.lvclass">)  [unwired: 7 in]
          n337 = call-dynamic "Write Interface.vi"("error in (no error)"=w976, "Interface.lvclass"=w978, "Channel in"=w1018) -> ("error out"=w997:errorcluster, "Channel out"=w996:refnum<class "Channel.lvclass">)  [unwired: 7 in]
          n338 = case shown="True" w983 {
            tunnel: [w1025 w1042] -> w1022
            tunnel: w1021 -> [w1026 w1043]
            tunnel: w997 -> [w1023 w1040]
            tunnel: [w1028 w1037] -> w995
            tunnel: w996 -> [w1029 w1041]
            tunnel: [w1027 w1034] -> w994
            tunnel: w990 -> [w1024 w1039]
            tunnel: w988 -> [_ w1033]
            frame True {
              # "Conneted=T\nACS respondeu"
              n339 = disable-structure shown="Enabled" {
                disable-tunnel: w1026 -> [w1031 _]
                disable-tunnel: [w1030 0] -> w1025
                frame Disabled {
                  n340 = Increment(x=w1031) -> (x+1=w1030:i32)
                }
                frame Enabled {
                }
              }
              n341 = call-dynamic "Write State Machine.vi"("error in (no error)"=w1023, "State Machine.lvclass"=w1024, "Device in"=w1029) -> ("error out"=w1027:errorcluster, "Device out"=w1028:refnum<class "Channel.lvclass">)  [unwired: 7 in]
            }
            frame False {
              # "Conneted=F\nACS não resp."
              n342 = case shown="True" w1033 {
                tunnel: w1043 -> [w1044 _]
                tunnel: [w1044 0] -> w1042
                tunnel: w1041 -> [w1047 w1050]
                tunnel: [w1047 w1050] -> w1038
                tunnel: w1040 -> [w1046 w1051]
                tunnel: [w1046 w1048] -> w1035
                tunnel: w1039 -> [w1045 w1053]
                tunnel: [w1045 w1049] -> w1036
                frame False {
                }
                frame True {
                  n343 = call-dynamic "Write Timer.vi"("error in (no error)"=w1051, "Timer"=u32 250, "State Machine in"=w1053) -> ("error out"=w1048:errorcluster, "State Machine out"=w1049:refnum<class "State Machine.lvclass">)  [unwired: 7 in]
                }
              }
              n344 = call-dynamic "Write State Machine.vi"("error in (no error)"=w1035, "State Machine.lvclass"=w1036, "Device in"=w1038) -> ("error out"=w1034:errorcluster, "Device out"=w1037:refnum<class "Channel.lvclass">)  [unwired: 7 in]
            }
          }
          n345 = Divide(x=w1007, y=100.0) -> (x/y=w1005:dbl)
          n346 = To Unsigned Long Integer(number=w1002) -> (unsigned 32bit integer=w999:u32)
          n347 = Multiply(x=w1009, y=w1005) -> (x*y=w1008:dbl)
          n348 = Bundle By Name(cluster=w995, "Texp"=w1008, "lastStatus"=w998, "Nimages"=w999, "CyclesDone"=w980, "SequesDone"=w975) -> (w1020:refnum<class "Channel.lvclass">)
        }
        frame 58 {
          w1059 = "}" ("regular expression")
          # "Passa valores da telemetria adquiridos do TCS"
          n349 = call-dynamic "Write State Machine.vi"("error in (no error)"=w1055, "State Machine.lvclass"=w1056, "Device in"=w1066) -> ("error out"=w1063:errorcluster, "Device out"=w1065:refnum<class "Channel.lvclass">)  [unwired: 7 in]
          n350 = Unbundle By Name(w1065) -> ("TCS telemetry"=w1060:string, "Filter"=w1062:u8)
          n351 = Match Pattern(string=w1060, regular expression=w1059) -> (before substring=w1058:string, match substring=w1057:string)  [unwired: 1 in, 2 out]
          n352 = Equal?(x=w1057, y=w1059) -> (x = y?=w1061:bool)
          n353 = case shown="True" w1061 {
            tunnel: [w1070 w1080] -> w1068
            tunnel: [w1069 w1079] -> w1067
            tunnel: w1065 -> [w1070 w1078]
            tunnel: w1063 -> [w1069 w1075]
            tunnel: w1062 -> [_ w1074]
            tunnel: w1058 -> [_ w1073]
            tunnel: w1057 -> [_ w1072]
            frame False {
            }
            frame True {
              (unwired) "\"CTRLINTE\":\"S4GUI\"}" ("string")
              (unwired) "\"FILTER\":\"" ("string")
              n354 = case shown="5" w1074 {
                tunnel: ["CLEAR\"," ("string") "U\"," ("string") "B\"," ("string") "V\"," ("string") "R\"," ("string") "S\"," ("string")] -> _
                frame 0, Default {
                }
                frame 1 {
                }
                frame 2 {
                }
                frame 3 {
                }
                frame 4 {
                }
                frame 5 {
                }
              }
              n355 = Concatenate Strings(w1073, w1072) -> (w1071:string)
              n356 = Concatenate Strings("WRITE_HEADER_DATA " ("cmd"), w1071) -> (w1076:string)
              n357 = call-dynamic "Write cmd.vi"("error in (no error)"=w1075, "cmd"=w1076, "Device in"=w1078) -> ("error out"=w1079:errorcluster, "Device out"=w1080:refnum<class "Channel.lvclass">)  [unwired: 7 in]
            }
          }
        }
        frame 59 {
          w1091 = "}" ("regular expression")
          # "Passa valores da telemetria adquiridos do TCS durante a aquisição do canal (estados 54 e 55)"
          n358 = call-dynamic "Write State Machine.vi"("error in (no error)"=w1087, "State Machine.lvclass"=w1088, "Device in"=w1097) -> ("error out"=w1094:errorcluster, "Device out"=w1096:refnum<class "Channel.lvclass">)  [unwired: 7 in]
          n359 = Unbundle By Name(w1096) -> ("TCS telemetry"=w1092:string)
          n360 = Match Pattern(string=w1092, regular expression=w1091) -> (before substring=w1090:string, match substring=w1089:string)  [unwired: 1 in, 2 out]
          n361 = Equal?(x=w1089, y=w1091) -> (x = y?=w1093:bool)
          n362 = case shown="True" w1093 {
            tunnel: [w1101 w1110] -> w1099
            tunnel: [w1100 w1109] -> w1098
            tunnel: w1096 -> [w1101 w1108]
            tunnel: w1094 -> [w1100 w1105]
            tunnel: w1090 -> [_ w1104]
            tunnel: w1089 -> [_ w1103]
            frame False {
            }
            frame True {
              n363 = Concatenate Strings(w1104, w1103) -> (w1102:string)
              n364 = Concatenate Strings("WRITE_HEADER_DATA " ("cmd"), w1102) -> (w1106:string)
              n365 = call-dynamic "Write cmd.vi"("error in (no error)"=w1105, "cmd"=w1106, "Device in"=w1108) -> ("error out"=w1109:errorcluster, "Device out"=w1110:refnum<class "Channel.lvclass">)  [unwired: 7 in]
            }
          }
        }
        frame 60 {
          # "Carrega timeout de 5 ciclos\npara resposta do ACS"
          n366 = call-dynamic "Write Timer.vi"("Timer"=u32 5, "State Machine in"=w1116) -> ("error out"=w1117:errorcluster, "State Machine out"=w1115:refnum<class "State Machine.lvclass">)  [unwired: 8 in]
          n367 = call-dynamic "Write State Machine.vi"("error in (no error)"=w1117, "State Machine.lvclass"=w1115, "Device in"=w1114) -> ("Device out"=w1113:refnum<class "Channel.lvclass">)  [unwired: 7 in, 1 out]
          n368 = disable-structure shown="Enabled" {
            disable-tunnel: [w1128 w1130] -> w1121
            disable-tunnel: w1120 -> [w1127 w1129]
            disable-tunnel: [w1126 w1129] -> w1119
            disable-tunnel: w1113 -> [w1124 w1130]
            disable-tunnel: w1112 -> [w1123 _]
            disable-tunnel: [w1122 62] -> w1111
            frame Disabled {
              n369 = Increment(x=w1123) -> (x+1=w1122:i32)
              n370 = call-dynamic "Write cmd.vi"("error in (no error)"=w1127, "cmd"="INIT", "Device in"=w1124) -> ("error out"=w1126:errorcluster, "Device out"=w1128:refnum<class "Channel.lvclass">)  [unwired: 7 in]
            }
            frame Enabled {
            }
          }
        }
        frame 61 {
          w1141 = "INITIALIZATION"
          # "Verifica timeout para ACS responder.\nSe estourar timeout é porque o ACS não \nrespondeu e este canal volta para o estado 0\npara não \"travar\" os outros canais no \nS4ACS_GUI:HandleObservation.vi."
          n371 = call "Verify Timer.vi"("error in (no error)"=w1132, "State Machine in"=w1137) -> ("error out"=w1138:errorcluster, "timeout"=w1133:bool, "State Machine out"=w1139:refnum<class "State Machine.lvclass">)  [unwired: 7 in]
          n372 = call-dynamic "Write State Machine.vi"("error in (no error)"=w1138, "State Machine.lvclass"=w1139, "Device in"=w1136) -> ("error out"=w1134:errorcluster, "Device out"=w1135:refnum<class "Channel.lvclass">)  [unwired: 7 in]
          n373 = call-dynamic "Read resp.vi"("error in (no error)"=w1134, "Device in"=w1135) -> ("error out"=w1145:errorcluster, "resp"=w1143:string, "Device out"=w1146:refnum<class "Channel.lvclass">)  [unwired: 7 in]
          "resp INIT" <- w1143
          n374 = Match Pattern(string=w1143, regular expression=w1141) -> (match substring=w1142:string)  [unwired: 1 in, 3 out]
          n375 = Equal?(x=w1142, y=w1141) -> (x = y?=w1140:bool)
          n376 = case shown="True" w1140 {
            tunnel: [w1148 w1153] -> w1147
            tunnel: w1144 -> [w1149 w1154]
            tunnel: w1133 -> [w1150 _]
            frame False {
              n377 = case shown="False" w1150 {
                tunnel: [w1151 0 ("State")] -> w1148
                tunnel: w1149 -> [w1151 _]
                frame False {
                }
                frame True {
                }
              }
            }
            frame True {
              n378 = disable-structure shown="Enabled" {
                disable-tunnel: w1154 -> [w1156 _]
                disable-tunnel: [w1155 54] -> w1153
                frame Disabled {
                  n379 = Increment(x=w1156) -> (x+1=w1155:i32)
                }
                frame Enabled {
                  # "debug:\nNão deve enviar\n WRITE_SETUP para o \nACS antigo"
                }
              }
            }
          }
        }
        frame 62 {
          # "Carrega timeout de 50 ciclos\npara resposta do ACS"
          n380 = call-dynamic "Write Timer.vi"("error in (no error)"=w1167, "Timer"=u32 50, "State Machine in"=w1170) -> ("error out"=w1171:errorcluster, "State Machine out"=w1169:refnum<class "State Machine.lvclass">)  [unwired: 7 in]
          n381 = call-dynamic "Write State Machine.vi"("error in (no error)"=w1171, "State Machine.lvclass"=w1169, "Device in"=w1168) -> ("error out"=w1164:errorcluster, "Device out"=w1166:refnum<class "Channel.lvclass">)  [unwired: 7 in]
          n382 = Unbundle By Name(w1166) -> ("Interface.lvclass"=w1165:refnum<class "Interface.lvclass">)
          n383 = call-dynamic "Get CCD_Config.vi"("error in (no error)"=w1164, "Interface in"=w1165) -> ("error out"=w1159:errorcluster, "output cluster"=w1161:T2)  [unwired: 7 in, 1 out]
          n384 = Flatten To JSON(anything=w1161, error in (no error)=w1159) -> (JSON string=w1160:string, 11:w1158:errorcluster)  [unwired: 1 in]
          n385 = Concatenate Strings("WRITE_SETUP " ("cmd"), w1160) -> (w1162:string)
          n386 = call-dynamic "Write cmd.vi"("error in (no error)"=w1158, "cmd"=w1162, "Device in"=w1166) -> ("error out"=w1175:errorcluster, "Device out"=w1176:refnum<class "Channel.lvclass">)  [unwired: 7 in]
          n387 = Increment(x=w1173) -> (x+1=w1174:i32)
        }
        frame 63 {
          # "Não há resposta para o comando WRTITE_SETUP\nQuando estourar timeout vai para o estado 64 para \nobter o STATUS do ACS."
          n388 = call "Verify Timer.vi"("error in (no error)"=w1180, "State Machine in"=w1182) -> ("error out"=w1183:errorcluster, "timeout"=w1179:bool, "State Machine out"=w1184:refnum<class "State Machine.lvclass">)  [unwired: 7 in]
          n389 = call-dynamic "Write State Machine.vi"("error in (no error)"=w1183, "State Machine.lvclass"=w1184, "Device in"=w1181) -> ("error out"=w1177:errorcluster, "Device out"=w1178:refnum<class "Channel.lvclass">)  [unwired: 7 in]
          n390 = case shown="False" w1179 {
            tunnel: [w1187 w1188] -> w1186
            tunnel: w1185 -> [w1187 w1189]
            frame False {
            }
            frame True {
              n391 = Increment(x=w1189) -> (x+1=w1188:i32)
            }
          }
        }
        frame 64 {
          # "Carrega timeout de 50 ciclos\npara resposta do ACS"
          n392 = call-dynamic "Write Timer.vi"("error in (no error)"=w1193, "Timer"=u32 50, "State Machine in"=w1196) -> ("error out"=w1197:errorcluster, "State Machine out"=w1195:refnum<class "State Machine.lvclass">)  [unwired: 7 in]
          n393 = call-dynamic "Write State Machine.vi"("error in (no error)"=w1197, "State Machine.lvclass"=w1195, "Device in"=w1194) -> ("error out"=w1190:errorcluster, "Device out"=w1192:refnum<class "Channel.lvclass">)  [unwired: 7 in]
          n394 = call-dynamic "Write cmd.vi"("error in (no error)"=w1190, "cmd"="READ_SETUP ", "Device in"=w1192) -> ("error out"=w1201:errorcluster, "Device out"=w1202:refnum<class "Channel.lvclass">)  [unwired: 7 in]
          n395 = Increment(x=w1199) -> (x+1=w1200:i32)
        }
        frame 65 {
          n396 = call "Verify Timer.vi"("error in (no error)"=w1221, "State Machine in"=w1223) -> ("error out"=w1224:errorcluster, "timeout"=w1207:bool, "State Machine out"=w1225:refnum<class "State Machine.lvclass">)  [unwired: 7 in]
          n397 = call-dynamic "Write State Machine.vi"("error in (no error)"=w1224, "State Machine.lvclass"=w1225, "Device in"=w1222) -> ("error out"=w1219:errorcluster, "Device out"=w1220:refnum<class "Channel.lvclass">)  [unwired: 7 in]
          n398 = call-dynamic "Read resp.vi"("error in (no error)"=w1219, "Device in"=w1220) -> ("error out"=w1213:errorcluster, "resp"=w1211:string, "Device out"=w1218:refnum<class "Channel.lvclass">)  [unwired: 7 in]
          n399 = Unbundle By Name(w1218) -> ("Interface.lvclass"=w1214:refnum<class "Interface.lvclass">)
          n400 = call-dynamic "Get CCD_Config.vi"("error in (no error)"=w1213, "Interface in"=w1214) -> ("error out"=w1215:errorcluster, "output cluster"=w1212:T2, "Interface out"=w1216:refnum<class "Interface.lvclass">)  [unwired: 7 in]
          n401 = case shown="True" w1207 {
            tunnel: w1216 -> [w1228 w1239]
            tunnel: w1215 -> [w1227 w1238]
            tunnel: w1212 -> [_ w1241]
            tunnel: w1211 -> [_ w1232]
            tunnel: [w1228 w1237] -> w1209
            tunnel: [w1227 w1236] -> w1210
            tunnel: [T1 {"ACQUISITION_MODE"=FALSE, "TRIGGER_MODE"=FALSE, "READ_MODE"=FALSE, "PREAMP"=FALSE, "READOUT_RATE"=FALSE, "VERTICAL_SHIFT_SPEED"=FALSE, "EM_MODE"=FALSE, "EM_GAIN"=FALSE, "SHUTTER_MODE"=FALSE, "SHUTTER_TTL"=FALSE, "SHUTTER_OPENING_TIME"=FALSE, "SHUTTER_CLOSING_TIME"=FALSE, "VBIN"=FALSE, "HBIN"=FALSE, "INITIAL_LINE"=FALSE, "INITIAL_COLUMN"=FALSE, "FINAL_LINE"=FALSE, "FINAL_COLUMN"=FALSE, "FRAME_TRANSFER"=FALSE, "VERTICAL_CLOCK_VOLTAGE"=FALSE, "AD_CHANNEL"=FALSE} ("x = y?") w1240] -> w1208
            tunnel: w1204 -> [w1226 w1231]
            tunnel: [w1226 w1230] -> w1203
            frame False {
            }
            frame True {
              w1233 = "\"HBIN\"" ("regular expression")
              n402 = Match Pattern(string=w1232, regular expression=w1233) -> (match substring=w1234:string)  [unwired: 1 in, 3 out]
              n403 = Equal?(x=w1233, y=w1234) -> (x = y?=w1235:bool)
              n404 = case shown="True" w1235 {
                tunnel: w1241 -> [_ w1253]
                tunnel: [T1 {"ACQUISITION_MODE"=FALSE, "TRIGGER_MODE"=FALSE, "READ_MODE"=FALSE, "PREAMP"=FALSE, "READOUT_RATE"=FALSE, "VERTICAL_SHIFT_SPEED"=FALSE, "EM_MODE"=FALSE, "EM_GAIN"=FALSE, "SHUTTER_MODE"=FALSE, "SHUTTER_TTL"=FALSE, "SHUTTER_OPENING_TIME"=FALSE, "SHUTTER_CLOSING_TIME"=FALSE, "VBIN"=FALSE, "HBIN"=FALSE, "INITIAL_LINE"=FALSE, "INITIAL_COLUMN"=FALSE, "FINAL_LINE"=FALSE, "FINAL_COLUMN"=FALSE, "FRAME_TRANSFER"=FALSE, "VERTICAL_CLOCK_VOLTAGE"=FALSE, "AD_CHANNEL"=FALSE} ("x = y?") w1252] -> w1240
                tunnel: w1239 -> [w1244 w1251]
                tunnel: w1238 -> [w1243 w1250]
                tunnel: [w1244 w1249] -> w1237
                tunnel: [w1243 w1248] -> w1236
                tunnel: w1232 -> [_ w1245]
                frame False {
                }
                frame True {
                  n405 = Unflatten From JSON(JSON string=w1245, type and defaults=w1253) -> (value=w1247:T2, error out=→"error out 2":errorcluster)  [unwired: 5 in]
                  n406 = call-dynamic "Set CCD_Config.vi"("error in (no error)"=w1250, "input cluster"=w1247, "Interface in"=w1251) -> ("error out"=w1248:errorcluster, "Interface out"=w1249:refnum<class "Interface.lvclass">)  [unwired: 7 in]
                  n407 = Equal?(x=w1247, y=w1253) -> (x = y?=w1252:T1)
                }
              }
              n408 = Increment(x=w1231) -> (x+1=w1230:i32)
            }
          }
          "x = y?" <- w1208
          n409 = call "Write Checked Params.vi"("error in (no error)"=w1210, "Checked Params"=w1208, "Interface in"=w1209) -> ("error out"=w1205:errorcluster, "Interface out"=w1206:refnum<class "Interface.lvclass">)  [unwired: 7 in]
          n410 = Bundle By Name(cluster=w1218, "Interface.lvclass"=w1206) -> (w1217:refnum<class "Channel.lvclass">)
        }
        frame 66 {
          # "O valor do COOLER aqui\nfoi carregado no Acquistion:Init.vi"
          # "Se COOLER=0\n        SET COLLERPOWER_STATUS 0\n        AVANÇA ESTADO\n        VAI PRA 0\nSe COOLER=1:\n      DESVIA PARA Estado 35"
          # "Carrega timeout de 50 ciclos\npara resposta do ACS"
          n411 = call-dynamic "Write Timer.vi"("error in (no error)"=w1261, "Timer"=u32 50, "State Machine in"=w1262) -> ("error out"=w1259:errorcluster, "State Machine out"=w1258:refnum<class "State Machine.lvclass">)  [unwired: 7 in]
          n412 = call-dynamic "Write State Machine.vi"("error in (no error)"=w1259, "State Machine.lvclass"=w1258, "Device in"=w1260) -> ("error out"=w1257:errorcluster, "Device out"=w1256:refnum<class "Channel.lvclass">)  [unwired: 7 in]
          n413 = Unbundle By Name(w1256) -> ("Interface.lvclass"=w1255:refnum<class "Interface.lvclass">)
          n414 = call-dynamic "Read Cooler ON_OFF.vi"("Interface in"=w1255) -> ("Cooler ON/OFF"=w1254:i16)  [unwired: 8 in, 2 out]
          n415 = case shown="1" w1254 {
            tunnel: [w1270 w1277] -> w1267
            tunnel: [w1269 w1276] -> w1266
            tunnel: [35 w1275] -> w1265
            tunnel: w1264 -> [_ w1274]
            tunnel: w1257 -> [w1269 w1272]
            tunnel: w1256 -> [w1270 w1271]
            frame 1 {
              # "Se COOLER foi carregado com 1 na inicialização.\ndesvia para 35 para setar a temperatura e ligar o COOLER."
            }
            frame 0, Default {
              n416 = Increment(x=w1274) -> (x+1=w1275:i32)
              n417 = call-dynamic "Write cmd.vi"("error in (no error)"=w1272, "cmd"="SET COOLER_POWER_STATUS 0", "Device in"=w1271) -> ("error out"=w1276:errorcluster, "Device out"=w1277:refnum<class "Channel.lvclass">)  [unwired: 7 in]
            }
          }
        }
        frame 67 {
          n418 = call "Verify Timer.vi"("error in (no error)"=w1281, "State Machine in"=w1285) -> ("error out"=w1280:errorcluster, "timeout"=w1278:bool, "State Machine out"=w1282:refnum<class "State Machine.lvclass">)  [unwired: 7 in]
          n419 = call-dynamic "Write State Machine.vi"("error in (no error)"=w1280, "State Machine.lvclass"=w1282, "Device in"=w1284) -> ("error out"=w1279:errorcluster, "Device out"=w1283:refnum<class "Channel.lvclass">)  [unwired: 7 in]
          n420 = call-dynamic "Read resp.vi"("error in (no error)"=w1279, "Device in"=w1283) -> ("error out"=w1287:errorcluster, "resp"=w1292:string, "Device out"=w1288:refnum<class "Channel.lvclass">)  [unwired: 7 in]
          n421 = Equal?(x=w1292, y="DONE") -> (x = y?=w1290:bool)
          n422 = case shown="True" w1290 {
            tunnel: [w1293 w1298] -> w1289
            tunnel: w1286 -> [w1294 _]
            tunnel: w1278 -> [w1295 _]
            frame False {
              n423 = case shown="True" w1295 {
                tunnel: [w1296 0 ("State")] -> w1293
                tunnel: w1294 -> [w1296 _]
                frame False {
                }
                frame True {
                }
              }
            }
            frame True {
              n424 = disable-structure shown="Enabled" {
                disable-tunnel: [54 ("State") 32 ("State")] -> w1298
                frame Disabled {
                }
                frame Enabled {
                  # "Lê COOLER e \nvai pra 0."
                }
              }
            }
          }
        }
        frame 70 {
          w1301 = "" ("resp")
          # "Carrega timeout de 5 ciclos\npara resposta do ACS"
          n425 = call-dynamic "Write Timer.vi"("error in (no error)"=w1315, "Timer"=u32 5, "State Machine in"=w1317) -> ("error out"=w1319:errorcluster, "State Machine out"=w1318:refnum<class "State Machine.lvclass">)  [unwired: 7 in]
          n426 = call-dynamic "Write State Machine.vi"("error in (no error)"=w1319, "State Machine.lvclass"=w1318, "Device in"=w1316) -> ("error out"=w1314:errorcluster, "Device out"=w1313:refnum<class "Channel.lvclass">)  [unwired: 7 in]
          n427 = call-dynamic "Write cmd.vi"("error in (no error)"=w1314, "cmd"="STOP_ACQUISITION", "Device in"=w1313) -> ("error out"=w1311:errorcluster, "Device out"=w1312:refnum<class "Channel.lvclass">)  [unwired: 7 in]
          n428 = call-dynamic "Write resp.vi"("error in (no error)"=w1311, "resp"=w1301, "Device in"=w1312) -> ("error out"=w1307:errorcluster, "Device out"=w1310:refnum<class "Channel.lvclass">)  [unwired: 7 in]
          n429 = call-dynamic "Read Interface.vi"("error in (no error)"=w1307, "Channel in"=w1310) -> ("error out"=w1306:errorcluster, "Interface.lvclass"=w1305:refnum<class "Interface.lvclass">, "Channel out"=w1309:refnum<class "Channel.lvclass">)  [unwired: 7 in]
          n430 = call-dynamic "UpdateStatus.vi"("error in (no error)"=w1306, "status"=w1301, "Interface in"=w1305) -> ("error out"=w1303:errorcluster, "Interface out"=w1304:refnum<class "Interface.lvclass">)  [unwired: 7 in]
          n431 = call-dynamic "Write Interface.vi"("error in (no error)"=w1303, "Interface.lvclass"=w1304, "Channel in"=w1309) -> ("error out"=w1302:errorcluster, "Channel out"=w1308:refnum<class "Channel.lvclass">)  [unwired: 7 in]
          n432 = Increment(x=w1322) -> (x+1=w1323:i32)
        }
        frame 71 {
          w1325 = "DONE"
          n433 = call-dynamic "Read resp.vi"("error in (no error)"=w1332, "Device in"=w1333) -> ("error out"=w1329:errorcluster, "resp"=w1327:string, "Device out"=w1330:refnum<class "Channel.lvclass">)  [unwired: 7 in]
          "resp STOP" <- w1327
          n434 = Match Pattern(string=w1327, regular expression=w1325) -> (match substring=w1326:string)  [unwired: 1 in, 3 out]
          n435 = Equal?(x=w1326, y=w1325) -> ()  [unwired: 1 out]
          n436 = case shown="True" TRUE {
            tunnel: [w1334 52 ("State")] -> w1331
            tunnel: w1328 -> [w1334 _]
            frame False {
            }
            frame True {
            }
          }
        }
        frame 80 {
          n437 = call-dynamic "Write cmd.vi"("error in (no error)"=w1345, "cmd"="ABORT_ACQUISITION", "Device in"=w1344) -> ("error out"=w1339:errorcluster, "Device out"=w1340:refnum<class "Channel.lvclass">)  [unwired: 7 in]
          n438 = call-dynamic "Write resp.vi"("error in (no error)"=w1339, "resp"="", "Device in"=w1340) -> ("error out"=w1338:errorcluster, "Device out"=w1337:refnum<class "Channel.lvclass">)  [unwired: 7 in]
          n439 = Increment(x=w1342) -> (x+1=w1343:i32)
        }
        frame 81 {
          w1347 = "DONE"
          n440 = call-dynamic "Read resp.vi"("error in (no error)"=w1354, "Device in"=w1355) -> ("error out"=w1351:errorcluster, "resp"=w1349:string, "Device out"=w1352:refnum<class "Channel.lvclass">)  [unwired: 7 in]
          "resp ABORT" <- w1349
          n441 = Match Pattern(string=w1349, regular expression=w1347) -> (match substring=w1348:string)  [unwired: 1 in, 3 out]
          n442 = Equal?(x=w1348, y=w1347) -> ()  [unwired: 1 out]
          n443 = case shown="True" TRUE {
            tunnel: [w1356 52 ("State")] -> w1353
            tunnel: w1350 -> [w1356 _]
            frame False {
            }
            frame True {
            }
          }
        }
        frame 90 {
          n444 = call-dynamic "Write cmd.vi"("error in (no error)"=w1367, "cmd"="PAUSE_ACQUISITION", "Device in"=w1366) -> ("error out"=w1361:errorcluster, "Device out"=w1362:refnum<class "Channel.lvclass">)  [unwired: 7 in]
          n445 = call-dynamic "Write resp.vi"("error in (no error)"=w1361, "resp"="", "Device in"=w1362) -> ("error out"=w1360:errorcluster, "Device out"=w1359:refnum<class "Channel.lvclass">)  [unwired: 7 in]
          n446 = Increment(x=w1364) -> (x+1=w1365:i32)
        }
        frame 91 {
          w1368 = "DONE"
          n447 = call-dynamic "Read resp.vi"("error in (no error)"=w1374, "Device in"=w1375) -> ("error out"=w1372:errorcluster, "resp"=w1370:string, "Device out"=w1373:refnum<class "Channel.lvclass">)  [unwired: 7 in]
          "resp PAUSE" <- w1370
          n448 = Match Pattern(string=w1370, regular expression=w1368) -> (match substring=w1369:string)  [unwired: 1 in, 3 out]
          n449 = Equal?(x=w1369, y=w1368) -> ()  [unwired: 1 out]
        }
        frame 96 {
          n450 = call-dynamic "Write cmd.vi"("error in (no error)"=w1385, "cmd"="RESUME_ACQUISITION", "Device in"=w1384) -> ("error out"=w1379:errorcluster, "Device out"=w1380:refnum<class "Channel.lvclass">)  [unwired: 7 in]
          n451 = call-dynamic "Write resp.vi"("error in (no error)"=w1379, "resp"="", "Device in"=w1380) -> ("error out"=w1378:errorcluster, "Device out"=w1377:refnum<class "Channel.lvclass">)  [unwired: 7 in]
          n452 = Increment(x=w1382) -> (x+1=w1383:i32)
        }
        frame 97 {
          w1390 = "DONE"
          n453 = call-dynamic "Read resp.vi"("error in (no error)"=w1394, "Device in"=w1395) -> ("error out"=w1388:errorcluster, "resp"=w1392:string, "Device out"=w1393:refnum<class "Channel.lvclass">)  [unwired: 7 in]
          "resp RESUME" <- w1392
          n454 = Match Pattern(string=w1392, regular expression=w1390) -> (match substring=w1391:string)  [unwired: 1 in, 3 out]
          n455 = Equal?(x=w1391, y=w1390) -> ()  [unwired: 1 out]
          n456 = call-dynamic "Read Return State.vi"("error in (no error)"=w1388, "State Machine in"=w1389) -> ("error out"=w1387:errorcluster, "Return State"=w1386:i32)  [unwired: 7 in, 1 out]
        }
        frame 100 {
          (unwired) "S4ACS C1/C2/C3/C4 NIMAGES " ("cmd")
          n457 = call-dynamic "Write cmd.vi"("error in (no error)"=w1401, "cmd"="INIT", "Device in"=w1399) -> ("error out"=w1400:errorcluster, "Device out"=w1402:refnum<class "Channel.lvclass">)  [unwired: 7 in]
          n458 = Increment(x=w1397) -> (x+1=w1398:i32)
        }
        frame 101 {
          w1404 = "\r\n"
          n459 = call-dynamic "Read resp.vi"("error in (no error)"=w1412, "Device in"=w1413) -> ("error out"=w1409:errorcluster, "resp"=w1403:string, "Device out"=w1406:refnum<class "Channel.lvclass">)  [unwired: 7 in]
          n460 = Match Pattern(string=w1403, regular expression=w1404) -> (match substring=w1407:string)  [unwired: 1 in, 3 out]
          n461 = Equal?(x=w1407, y=w1404) -> (x = y?=w1411:bool)
          n462 = case shown="False" w1411 {
            tunnel: [w1414 u8 0] -> w1410
            tunnel: w1408 -> [w1414 _]
            tunnel: w1406 -> [w1415 w1419]
            tunnel: [w1415 w1418] -> w1405
            tunnel: w1403 -> [_ w1417]
            frame False {
            }
            frame True {
              n463 = Bundle By Name(cluster=w1419, "lastStatus"=w1417) -> (w1418:refnum<class "Channel.lvclass">)
            }
          }
        }
        frame 102 {
          w1427 = "EXPTIME "
          n464 = Unbundle By Name(w1421) -> ("lastStatus"=w1422:string)
          n465 = Match Pattern(string=w1422, regular expression=w1427) -> (match substring=w1426:string, after substring=w1424:string)  [unwired: 1 in, 2 out]
          n466 = Equal?(x=w1426, y=w1427) -> (x = y?=w1430:bool)
          n467 = case shown="True" w1430 {
            tunnel: [w1431 w1433] -> w1429
            tunnel: w1428 -> [w1431 w1433]
            tunnel: w1421 -> [w1432 w1439]
            tunnel: [w1432 w1437] -> w1425
            tunnel: w1424 -> [_ w1435]
            frame False {
            }
            frame True {
              n468 = call <vilib>:"Space Constant.vi"() -> ("String"=w1436:string)
              n469 = Match Pattern(string=w1435, regular expression=w1436) -> (before substring=w1434:string)  [unwired: 1 in, 3 out]
              n470 = Fract/Exp String To Number(string=w1434) -> (number=w1438:dbl)  [unwired: 3 in, 1 out]
              n471 = Bundle By Name(cluster=w1439, "Texp"=w1438) -> (w1437:refnum<class "Channel.lvclass">)
            }
          }
          n472 = Increment(x=w1429) -> (x+1=w1420:i32)
        }
        frame 103 {
          w1447 = "NIMAGES "
          n473 = Unbundle By Name(w1441) -> ("lastStatus"=w1442:string)
          n474 = Match Pattern(string=w1442, regular expression=w1447) -> (match substring=w1446:string, after substring=w1444:string)  [unwired: 1 in, 2 out]
          n475 = Equal?(x=w1446, y=w1447) -> (x = y?=w1450:bool)
          n476 = case shown="True" w1450 {
            tunnel: [w1451 w1453] -> w1449
            tunnel: w1448 -> [w1451 w1453]
            tunnel: w1441 -> [w1452 w1459]
            tunnel: [w1452 w1457] -> w1445
            tunnel: w1444 -> [_ w1455]
            frame False {
            }
            frame True {
              n477 = call <vilib>:"Space Constant.vi"() -> ("String"=w1456:string)
              n478 = Match Pattern(string=w1455, regular expression=w1456) -> (before substring=w1454:string)  [unwired: 1 in, 3 out]
              n479 = Fract/Exp String To Number(string=w1454) -> (number=w1458:dbl)  [unwired: 3 in, 1 out]
              n480 = Bundle By Name(cluster=w1459, "Nimages"=w1458) -> (w1457:refnum<class "Channel.lvclass">)
            }
          }
          n481 = Increment(x=w1449) -> (x+1=w1440:i32)
        }
        frame 104 {
          w1467 = "INITIAL_LINE "
          n482 = Unbundle By Name(w1461) -> ("lastStatus"=w1462:string)
          n483 = Match Pattern(string=w1462, regular expression=w1467) -> (match substring=w1466:string, after substring=w1464:string)  [unwired: 1 in, 2 out]
          n484 = Equal?(x=w1466, y=w1467) -> (x = y?=w1470:bool)
          n485 = case shown="True" w1470 {
            tunnel: [w1471 w1473] -> w1469
            tunnel: w1468 -> [w1471 w1473]
            tunnel: w1461 -> [w1472 w1479]
            tunnel: [w1472 w1477] -> w1465
            tunnel: w1464 -> [_ w1475]
            frame False {
            }
            frame True {
              n486 = call <vilib>:"Space Constant.vi"() -> ("String"=w1476:string)
              n487 = Match Pattern(string=w1475, regular expression=w1476) -> (before substring=w1474:string)  [unwired: 1 in, 3 out]
              n488 = Fract/Exp String To Number(string=w1474) -> (number=w1478:dbl)  [unwired: 3 in, 1 out]
              n489 = Bundle By Name(cluster=w1479, "InitialLine"=w1478) -> (w1477:refnum<class "Channel.lvclass">)
            }
          }
          n490 = Increment(x=w1469) -> (x+1=w1460:i32)
        }
        frame 105 {
          w1487 = "FINAL_LINE "
          n491 = Unbundle By Name(w1481) -> ("lastStatus"=w1482:string)
          n492 = Match Pattern(string=w1482, regular expression=w1487) -> (match substring=w1486:string, after substring=w1484:string)  [unwired: 1 in, 2 out]
          n493 = Equal?(x=w1486, y=w1487) -> (x = y?=w1490:bool)
          n494 = case shown="True" w1490 {
            tunnel: [w1491 w1493] -> w1489
            tunnel: w1488 -> [w1491 w1493]
            tunnel: w1481 -> [w1492 w1499]
            tunnel: [w1492 w1497] -> w1485
            tunnel: w1484 -> [_ w1495]
            frame False {
            }
            frame True {
              n495 = call <vilib>:"Space Constant.vi"() -> ("String"=w1496:string)
              n496 = Match Pattern(string=w1495, regular expression=w1496) -> (before substring=w1494:string)  [unwired: 1 in, 3 out]
              n497 = Fract/Exp String To Number(string=w1494) -> (number=w1498:dbl)  [unwired: 3 in, 1 out]
              n498 = Bundle By Name(cluster=w1499, "FinalLine"=w1498) -> (w1497:refnum<class "Channel.lvclass">)
            }
          }
          n499 = Increment(x=w1489) -> (x+1=w1480:i32)
        }
        frame 106 {
          w1507 = "INITIAL_COLUMN "
          n500 = Unbundle By Name(w1501) -> ("lastStatus"=w1502:string)
          n501 = Match Pattern(string=w1502, regular expression=w1507) -> (match substring=w1506:string, after substring=w1504:string)  [unwired: 1 in, 2 out]
          n502 = Equal?(x=w1506, y=w1507) -> (x = y?=w1510:bool)
          n503 = case shown="True" w1510 {
            tunnel: [w1511 w1513] -> w1509
            tunnel: w1508 -> [w1511 w1513]
            tunnel: w1501 -> [w1512 w1519]
            tunnel: [w1512 w1517] -> w1505
            tunnel: w1504 -> [_ w1515]
            frame False {
            }
            frame True {
              n504 = call <vilib>:"Space Constant.vi"() -> ("String"=w1516:string)
              n505 = Match Pattern(string=w1515, regular expression=w1516) -> (before substring=w1514:string)  [unwired: 1 in, 3 out]
              n506 = Fract/Exp String To Number(string=w1514) -> (number=w1518:dbl)  [unwired: 3 in, 1 out]
              n507 = Bundle By Name(cluster=w1519, "InitialColumn"=w1518) -> (w1517:refnum<class "Channel.lvclass">)
            }
          }
          n508 = Increment(x=w1509) -> (x+1=w1500:i32)
        }
        frame 107 {
          w1527 = "FINAL_COLUMN "
          n509 = Unbundle By Name(w1521) -> ("lastStatus"=w1522:string)
          n510 = Match Pattern(string=w1522, regular expression=w1527) -> (match substring=w1526:string, after substring=w1524:string)  [unwired: 1 in, 2 out]
          n511 = Equal?(x=w1526, y=w1527) -> (x = y?=w1530:bool)
          n512 = case shown="True" w1530 {
            tunnel: [w1531 w1533] -> w1529
            tunnel: w1528 -> [w1531 w1533]
            tunnel: w1521 -> [w1532 w1539]
            tunnel: [w1532 w1537] -> w1525
            tunnel: w1524 -> [_ w1535]
            frame False {
            }
            frame True {
              n513 = call <vilib>:"Space Constant.vi"() -> ("String"=w1536:string)
              n514 = Match Pattern(string=w1535, regular expression=w1536) -> (before substring=w1534:string)  [unwired: 1 in, 3 out]
              n515 = Fract/Exp String To Number(string=w1534) -> (number=w1538:dbl)  [unwired: 3 in, 1 out]
              n516 = Bundle By Name(cluster=w1539, "FinalColumn"=w1538) -> (w1537:refnum<class "Channel.lvclass">)
            }
          }
          n517 = Increment(x=w1529) -> (x+1=w1520:i32)
        }
        frame 108 {
          w1547 = "EM_GAIN "
          n518 = Unbundle By Name(w1541) -> ("lastStatus"=w1542:string)
          n519 = Match Pattern(string=w1542, regular expression=w1547) -> (match substring=w1546:string, after substring=w1544:string)  [unwired: 1 in, 2 out]
          n520 = Equal?(x=w1546, y=w1547) -> (x = y?=w1550:bool)
          n521 = case shown="True" w1550 {
            tunnel: [w1551 w1553] -> w1549
            tunnel: w1548 -> [w1551 w1553]
            tunnel: w1541 -> [w1552 w1559]
            tunnel: [w1552 w1557] -> w1545
            tunnel: w1544 -> [_ w1555]
            frame False {
            }
            frame True {
              n522 = call <vilib>:"Space Constant.vi"() -> ("String"=w1556:string)
              n523 = Match Pattern(string=w1555, regular expression=w1556) -> (before substring=w1554:string)  [unwired: 1 in, 3 out]
              n524 = Fract/Exp String To Number(string=w1554) -> (number=w1558:dbl)  [unwired: 3 in, 1 out]
              n525 = Bundle By Name(cluster=w1559, "EmGain"=w1558) -> (w1557:refnum<class "Channel.lvclass">)
            }
          }
          n526 = Increment(x=w1549) -> (x+1=w1540:i32)
        }
        frame 109 {
          w1567 = "COOLER "
          n527 = Unbundle By Name(w1561) -> ("lastStatus"=w1562:string)
          n528 = Match Pattern(string=w1562, regular expression=w1567) -> (match substring=w1566:string, after substring=w1564:string)  [unwired: 1 in, 2 out]
          n529 = Equal?(x=w1566, y=w1567) -> (x = y?=w1570:bool)
          n530 = case shown="True" w1570 {
            tunnel: [w1571 w1573] -> w1569
            tunnel: w1568 -> [w1571 w1573]
            tunnel: w1561 -> [w1572 w1580]
            tunnel: [w1572 w1579] -> w1565
            tunnel: w1564 -> [_ w1577]
            frame False {
            }
            frame True {
              n531 = call <vilib>:"Space Constant.vi"() -> ("String"=w1578:string)
              n532 = Match Pattern(string=w1577, regular expression=w1578) -> (before substring=w1576:string)  [unwired: 1 in, 3 out]
              n533 = Equal?(x=w1576, y="ON") -> (x = y?=w1574:bool)
              n534 = Bundle By Name(cluster=w1580, "Cooler Off"=w1574) -> (w1579:refnum<class "Channel.lvclass">)
            }
          }
          n535 = Increment(x=w1569) -> (x+1=w1560:i32)
        }
        frame 110 {
        }
        frame 200 {
          n536 = Unbundle By Name(w1592) -> ("Interface.lvclass"=w1591:refnum<class "Interface.lvclass">)
          n537 = call "Read Camera Setup.vi"("Interface in"=w1591) -> ("Camera Setup"=w1585:T3)  [unwired: 8 in, 2 out]
          n538 = Unbundle By Name(w1585) -> ("EXPTIME"=w1584:dbl)
          n539 = Number To Fractional String(number=w1584) -> (F-format string=w1586:string)  [unwired: 3 in]
          n540 = Concatenate Strings("SET EXPTIME " ("cmd"), w1586) -> (w1590:string)
          n541 = call-dynamic "Write cmd.vi"("error in (no error)"=w1594, "cmd"=w1590, "Device in"=w1592) -> ("error out"=w1593:errorcluster, "Device out"=w1595:refnum<class "Channel.lvclass">)  [unwired: 7 in]
          n542 = Increment(x=w1588) -> (x+1=w1589:i32)
        }
        frame 201 {
          n543 = call-dynamic "Read resp.vi"("error in (no error)"=w1603, "Device in"=w1604) -> ("error out"=w1597:errorcluster, "resp"=w1602:string, "Device out"=w1598:refnum<class "Channel.lvclass">)  [unwired: 7 in]
          n544 = Equal?(x=w1602, y="DONE") -> (x = y?=w1600:bool)
          n545 = case shown="True" w1600 {
            tunnel: [w1605 w1606] -> w1599
            tunnel: w1596 -> [w1605 w1607]
            frame False {
            }
            frame True {
              n546 = Increment(x=w1607) -> (x+1=w1606:i32)
            }
          }
        }
        frame 202 {
          n547 = call-dynamic "Write cmd.vi"("error in (no error)"=w1613, "cmd"="GET EXPTIME", "Device in"=w1611) -> ("error out"=w1612:errorcluster, "Device out"=w1614:refnum<class "Channel.lvclass">)  [unwired: 7 in]
          n548 = Increment(x=w1609) -> (x+1=w1610:i32)
        }
        frame 203 {
          n549 = call-dynamic "Read resp.vi"("error in (no error)"=w1625, "Device in"=w1626) -> ("error out"=w1623:errorcluster, "resp"=w1618:string, "Device out"=w1621:refnum<class "Channel.lvclass">)  [unwired: 7 in]
          n550 = Fract/Exp String To Number(string=w1618) -> (number=w1615:dbl)  [unwired: 3 in, 1 out]
          n551 = Unbundle By Name(w1621) -> ("Interface.lvclass"=w1620:refnum<class "Interface.lvclass">)
          n552 = call "Read Camera Setup.vi"("Interface in"=w1620) -> ("Camera Setup"=w1619:T3)  [unwired: 8 in, 2 out]
          n553 = Unbundle By Name(w1619) -> ("EXPTIME"=w1616:dbl)
          n554 = Equal?(x=w1616, y=w1615) -> (x = y?=w1617:bool)
          n555 = disable-structure shown="Enabled" {
            disable-tunnel: [w1629 224 ("State")] -> w1624
            disable-tunnel: w1622 -> [w1628 _]
            disable-tunnel: w1617 -> [w1627 _]
            frame Disabled {
              n556 = case shown="True" w1627 {
                tunnel: [w1630 w1631] -> w1629
                tunnel: w1628 -> [w1630 w1632]
                frame False {
                }
                frame True {
                  n557 = Increment(x=w1632) -> (x+1=w1631:i32)
                }
              }
            }
            frame Enabled {
            }
          }
        }
        frame 204 {
          n558 = Unbundle By Name(w1642) -> ("Interface.lvclass"=w1641:refnum<class "Interface.lvclass">)
          n559 = call "Read Camera Setup.vi"("Interface in"=w1641) -> ("Camera Setup"=w1635:T3)  [unwired: 8 in, 2 out]
          n560 = Unbundle By Name(w1635) -> ("#FRAMES"=w1634:u32)
          n561 = Number To Fractional String(number=w1634) -> (F-format string=w1636:string)  [unwired: 3 in]
          n562 = Concatenate Strings("SET #FRAMES " ("cmd"), w1636) -> (w1640:string)
          n563 = call-dynamic "Write cmd.vi"("error in (no error)"=w1644, "cmd"=w1640, "Device in"=w1642) -> ("error out"=w1643:errorcluster, "Device out"=w1645:refnum<class "Channel.lvclass">)  [unwired: 7 in]
          n564 = Increment(x=w1638) -> (x+1=w1639:i32)
        }
        frame 205 {
          n565 = call-dynamic "Read resp.vi"("error in (no error)"=w1653, "Device in"=w1654) -> ("error out"=w1647:errorcluster, "resp"=w1652:string, "Device out"=w1648:refnum<class "Channel.lvclass">)  [unwired: 7 in]
          n566 = Equal?(x=w1652, y="DONE") -> (x = y?=w1650:bool)
          n567 = case shown="True" w1650 {
            tunnel: [w1655 w1656] -> w1649
            tunnel: w1646 -> [w1655 w1657]
            frame False {
            }
            frame True {
              n568 = Increment(x=w1657) -> (x+1=w1656:i32)
            }
          }
        }
        frame 206 {
          n569 = call-dynamic "Write cmd.vi"("error in (no error)"=w1663, "cmd"="GET #FRAMES", "Device in"=w1661) -> ("error out"=w1662:errorcluster, "Device out"=w1664:refnum<class "Channel.lvclass">)  [unwired: 7 in]
          n570 = Increment(x=w1659) -> (x+1=w1660:i32)
        }
        frame 207 {
          n571 = call-dynamic "Read resp.vi"("error in (no error)"=w1676, "Device in"=w1677) -> ("error out"=w1674:errorcluster, "resp"=w1669:string, "Device out"=w1672:refnum<class "Channel.lvclass">)  [unwired: 7 in]
          n572 = Decimal String To Number(string=w1669) -> (number=w1667:i32)  [unwired: 2 in, 1 out]
          n573 = Unbundle By Name(w1672) -> ("Interface.lvclass"=w1671:refnum<class "Interface.lvclass">)
          n574 = call "Read Camera Setup.vi"("Interface in"=w1671) -> ("Camera Setup"=w1670:T3)  [unwired: 8 in, 2 out]
          n575 = To Unsigned Long Integer(number=w1667) -> (unsigned 32bit integer=w1665:u32)
          n576 = Unbundle By Name(w1670) -> ("#FRAMES"=w1666:u32)
          n577 = Equal?(x=w1666, y=w1665) -> (x = y?=w1668:bool)
          n578 = case shown="True" w1668 {
            tunnel: [w1678 w1679] -> w1675
            tunnel: w1673 -> [w1678 w1680]
            frame False {
            }
            frame True {
              n579 = Increment(x=w1680) -> (x+1=w1679:i32)
            }
          }
        }
        frame 208 {
          n580 = Unbundle By Name(w1689) -> ("Interface.lvclass"=w1688:refnum<class "Interface.lvclass">)
          n581 = call "Read Camera Setup.vi"("Interface in"=w1688) -> ("Camera Setup"=w1682:T3)  [unwired: 8 in, 2 out]
          n582 = Unbundle By Name(w1682) -> ("TRIGGER_MODE"=w1681:u8)
          n583 = Number To Fractional String(number=w1681) -> (F-format string=w1683:string)  [unwired: 3 in]
          n584 = Concatenate Strings("SET TRIGGER_MODE " ("cmd"), w1683) -> (w1687:string)
          n585 = call-dynamic "Write cmd.vi"("error in (no error)"=w1691, "cmd"=w1687, "Device in"=w1689) -> ("error out"=w1690:errorcluster, "Device out"=w1692:refnum<class "Channel.lvclass">)  [unwired: 7 in]
          n586 = Increment(x=w1685) -> (x+1=w1686:i32)
        }
        frame 209 {
          n587 = call-dynamic "Read resp.vi"("error in (no error)"=w1700, "Device in"=w1701) -> ("error out"=w1694:errorcluster, "resp"=w1699:string, "Device out"=w1695:refnum<class "Channel.lvclass">)  [unwired: 7 in]
          n588 = Equal?(x=w1699, y="DONE") -> (x = y?=w1697:bool)
          n589 = case shown="True" w1697 {
            tunnel: [w1702 w1703] -> w1696
            tunnel: w1693 -> [w1702 w1704]
            frame False {
            }
            frame True {
              n590 = Increment(x=w1704) -> (x+1=w1703:i32)
            }
          }
        }
        frame 210 {
          n591 = call-dynamic "Write cmd.vi"("error in (no error)"=w1710, "cmd"="GET TRIGGER_MODE", "Device in"=w1708) -> ("error out"=w1709:errorcluster, "Device out"=w1711:refnum<class "Channel.lvclass">)  [unwired: 7 in]
          n592 = Increment(x=w1706) -> (x+1=w1707:i32)
        }
        frame 211 {
          n593 = call-dynamic "Read resp.vi"("error in (no error)"=w1722, "Device in"=w1723) -> ("error out"=w1720:errorcluster, "resp"=w1715:string, "Device out"=w1718:refnum<class "Channel.lvclass">)  [unwired: 7 in]
          n594 = Fract/Exp String To Number(string=w1715) -> (number=w1713:dbl)  [unwired: 3 in, 1 out]
          n595 = Unbundle By Name(w1718) -> ("Interface.lvclass"=w1717:refnum<class "Interface.lvclass">)
          n596 = call "Read Camera Setup.vi"("Interface in"=w1717) -> ("Camera Setup"=w1716:T3)  [unwired: 8 in, 2 out]
          n597 = Unbundle By Name(w1716) -> ("TRIGGER_MODE"=w1712:u8)
          n598 = Equal?(x=w1712, y=w1713) -> (x = y?=w1714:bool)
          n599 = case shown="False" w1714 {
            tunnel: [w1724 w1725] -> w1721
            tunnel: w1719 -> [w1724 w1726]
            frame False {
            }
            frame True {
              n600 = Increment(x=w1726) -> (x+1=w1725:i32)
            }
          }
        }
        frame 212 {
          n601 = Unbundle By Name(w1735) -> ("Interface.lvclass"=w1734:refnum<class "Interface.lvclass">)
          n602 = call "Read Camera Setup.vi"("Interface in"=w1734) -> ("Camera Setup"=w1728:T3)  [unwired: 8 in, 2 out]
          n603 = Unbundle By Name(w1728) -> ("READ_MODE"=w1727:u8)
          n604 = Number To Fractional String(number=w1727) -> (F-format string=w1729:string)  [unwired: 3 in]
          n605 = Concatenate Strings("SET READ_MODE " ("cmd"), w1729) -> (w1733:string)
          n606 = call-dynamic "Write cmd.vi"("error in (no error)"=w1737, "cmd"=w1733, "Device in"=w1735) -> ("error out"=w1736:errorcluster, "Device out"=w1738:refnum<class "Channel.lvclass">)  [unwired: 7 in]
          n607 = Increment(x=w1731) -> (x+1=w1732:i32)
        }
        frame 213 {
          n608 = call-dynamic "Read resp.vi"("error in (no error)"=w1746, "Device in"=w1747) -> ("error out"=w1740:errorcluster, "resp"=w1745:string, "Device out"=w1741:refnum<class "Channel.lvclass">)  [unwired: 7 in]
          n609 = Equal?(x=w1745, y="DONE") -> (x = y?=w1743:bool)
          n610 = case shown="True" w1743 {
            tunnel: [w1748 w1749] -> w1742
            tunnel: w1739 -> [w1748 w1750]
            frame False {
            }
            frame True {
              n611 = Increment(x=w1750) -> (x+1=w1749:i32)
            }
          }
        }
        frame 214 {
          n612 = call-dynamic "Write cmd.vi"("error in (no error)"=w1756, "cmd"="GET READ_MODE", "Device in"=w1754) -> ("error out"=w1755:errorcluster, "Device out"=w1757:refnum<class "Channel.lvclass">)  [unwired: 7 in]
          n613 = Increment(x=w1752) -> (x+1=w1753:i32)
        }
        frame 215 {
          n614 = call-dynamic "Read resp.vi"("error in (no error)"=w1768, "Device in"=w1769) -> ("error out"=w1766:errorcluster, "resp"=w1761:string, "Device out"=w1764:refnum<class "Channel.lvclass">)  [unwired: 7 in]
          n615 = Fract/Exp String To Number(string=w1761) -> (number=w1759:dbl)  [unwired: 3 in, 1 out]
          n616 = Unbundle By Name(w1764) -> ("Interface.lvclass"=w1763:refnum<class "Interface.lvclass">)
          n617 = call "Read Camera Setup.vi"("Interface in"=w1763) -> ("Camera Setup"=w1762:T3)  [unwired: 8 in, 2 out]
          n618 = Unbundle By Name(w1762) -> ("READ_MODE"=w1758:u8)
          n619 = Equal?(x=w1758, y=w1759) -> (x = y?=w1760:bool)
          n620 = case shown="True" w1760 {
            tunnel: [w1770 w1771] -> w1767
            tunnel: w1765 -> [w1770 w1772]
            frame False {
            }
            frame True {
              n621 = Increment(x=w1772) -> (x+1=w1771:i32)
            }
          }
        }
        frame 216 {
          n622 = Unbundle By Name(w1781) -> ("Interface.lvclass"=w1780:refnum<class "Interface.lvclass">)
          n623 = call "Read Camera Setup.vi"("Interface in"=w1780) -> ("Camera Setup"=w1774:T3)  [unwired: 8 in, 2 out]
          n624 = Unbundle By Name(w1774) -> ("READOUT_RATE"=w1773:u8)
          n625 = Number To Fractional String(number=w1773) -> (F-format string=w1775:string)  [unwired: 3 in]
          n626 = Concatenate Strings("SET READOUT_RATE " ("cmd"), w1775) -> (w1779:string)
          n627 = call-dynamic "Write cmd.vi"("error in (no error)"=w1783, "cmd"=w1779, "Device in"=w1781) -> ("error out"=w1782:errorcluster, "Device out"=w1784:refnum<class "Channel.lvclass">)  [unwired: 7 in]
          n628 = Increment(x=w1777) -> (x+1=w1778:i32)
        }
        frame 217 {
          n629 = call-dynamic "Read resp.vi"("error in (no error)"=w1792, "Device in"=w1793) -> ("error out"=w1786:errorcluster, "resp"=w1791:string, "Device out"=w1787:refnum<class "Channel.lvclass">)  [unwired: 7 in]
          n630 = Equal?(x=w1791, y="DONE") -> (x = y?=w1789:bool)
          n631 = case shown="True" w1789 {
            tunnel: [w1794 w1795] -> w1788
            tunnel: w1785 -> [w1794 w1796]
            frame False {
            }
            frame True {
              n632 = Increment(x=w1796) -> (x+1=w1795:i32)
            }
          }
        }
        frame 218 {
          n633 = call-dynamic "Write cmd.vi"("error in (no error)"=w1802, "cmd"="GET READOUT_RATE", "Device in"=w1800) -> ("error out"=w1801:errorcluster, "Device out"=w1803:refnum<class "Channel.lvclass">)  [unwired: 7 in]
          n634 = Increment(x=w1798) -> (x+1=w1799:i32)
        }
        frame 219 {
          n635 = call-dynamic "Read resp.vi"("error in (no error)"=w1814, "Device in"=w1815) -> ("error out"=w1812:errorcluster, "resp"=w1807:string, "Device out"=w1810:refnum<class "Channel.lvclass">)  [unwired: 7 in]
          n636 = Fract/Exp String To Number(string=w1807) -> (number=w1805:dbl)  [unwired: 3 in, 1 out]
          n637 = Unbundle By Name(w1810) -> ("Interface.lvclass"=w1809:refnum<class "Interface.lvclass">)
          n638 = call "Read Camera Setup.vi"("Interface in"=w1809) -> ("Camera Setup"=w1808:T3)  [unwired: 8 in, 2 out]
          n639 = Unbundle By Name(w1808) -> ("READOUT_RATE"=w1804:u8)
          n640 = Equal?(x=w1804, y=w1805) -> (x = y?=w1806:bool)
          n641 = case shown="True" w1806 {
            tunnel: [w1816 w1817] -> w1813
            tunnel: w1811 -> [w1816 w1818]
            frame False {
            }
            frame True {
              n642 = Increment(x=w1818) -> (x+1=w1817:i32)
            }
          }
        }
        frame 220 {
          n643 = Unbundle By Name(w1827) -> ("Interface.lvclass"=w1826:refnum<class "Interface.lvclass">)
          n644 = call "Read Camera Setup.vi"("Interface in"=w1826) -> ("Camera Setup"=w1820:T3)  [unwired: 8 in, 2 out]
          n645 = Unbundle By Name(w1820) -> ("VERTICAL_SHIFT_SPEED"=w1819:u8)
          n646 = Number To Fractional String(number=w1819) -> (F-format string=w1821:string)  [unwired: 3 in]
          n647 = Concatenate Strings("SET VERTICAL_SHIFT_SPEED " ("cmd"), w1821) -> (w1825:string)
          n648 = call-dynamic "Write cmd.vi"("error in (no error)"=w1829, "cmd"=w1825, "Device in"=w1827) -> ("error out"=w1828:errorcluster, "Device out"=w1830:refnum<class "Channel.lvclass">)  [unwired: 7 in]
          n649 = Increment(x=w1823) -> (x+1=w1824:i32)
        }
        frame 221 {
          n650 = call-dynamic "Read resp.vi"("error in (no error)"=w1838, "Device in"=w1839) -> ("error out"=w1832:errorcluster, "resp"=w1837:string, "Device out"=w1833:refnum<class "Channel.lvclass">)  [unwired: 7 in]
          n651 = Equal?(x=w1837, y="DONE") -> (x = y?=w1835:bool)
          n652 = case shown="True" w1835 {
            tunnel: [w1840 w1841] -> w1834
            tunnel: w1831 -> [w1840 w1842]
            frame False {
            }
            frame True {
              n653 = Increment(x=w1842) -> (x+1=w1841:i32)
            }
          }
        }
        frame 222 {
          n654 = call-dynamic "Write cmd.vi"("error in (no error)"=w1848, "cmd"="GET VERTICAL_SHIFT_SPEED", "Device in"=w1846) -> ("error out"=w1847:errorcluster, "Device out"=w1849:refnum<class "Channel.lvclass">)  [unwired: 7 in]
          n655 = Increment(x=w1844) -> (x+1=w1845:i32)
        }
        frame 223 {
          n656 = call-dynamic "Read resp.vi"("error in (no error)"=w1860, "Device in"=w1861) -> ("error out"=w1858:errorcluster, "resp"=w1853:string, "Device out"=w1856:refnum<class "Channel.lvclass">)  [unwired: 7 in]
          n657 = Fract/Exp String To Number(string=w1853) -> (number=w1851:dbl)  [unwired: 3 in, 1 out]
          n658 = Unbundle By Name(w1856) -> ("Interface.lvclass"=w1855:refnum<class "Interface.lvclass">)
          n659 = call "Read Camera Setup.vi"("Interface in"=w1855) -> ("Camera Setup"=w1854:T3)  [unwired: 8 in, 2 out]
          n660 = Unbundle By Name(w1854) -> ("VERTICAL_SHIFT_SPEED"=w1850:u8)
          n661 = Equal?(x=w1850, y=w1851) -> (x = y?=w1852:bool)
          n662 = case shown="True" w1852 {
            tunnel: [w1862 w1863] -> w1859
            tunnel: w1857 -> [w1862 w1864]
            frame False {
            }
            frame True {
              n663 = Increment(x=w1864) -> (x+1=w1863:i32)
            }
          }
        }
        frame 224 {
          n664 = Unbundle By Name(w1873) -> ("Interface.lvclass"=w1872:refnum<class "Interface.lvclass">)
          n665 = call "Read Camera Setup.vi"("Interface in"=w1872) -> ("Camera Setup"=w1866:T3)  [unwired: 8 in, 2 out]
          n666 = Unbundle By Name(w1866) -> ("PREAMP"=w1865:u8)
          n667 = Number To Fractional String(number=w1865) -> (F-format string=w1867:string)  [unwired: 3 in]
          n668 = Concatenate Strings("SET PREAMP " ("cmd"), w1867) -> (w1871:string)
          n669 = call-dynamic "Write cmd.vi"("error in (no error)"=w1875, "cmd"=w1871, "Device in"=w1873) -> ("error out"=w1874:errorcluster, "Device out"=w1876:refnum<class "Channel.lvclass">)  [unwired: 7 in]
          n670 = Increment(x=w1869) -> (x+1=w1870:i32)
        }
        frame 225 {
          n671 = call-dynamic "Read resp.vi"("error in (no error)"=w1884, "Device in"=w1885) -> ("error out"=w1878:errorcluster, "resp"=w1883:string, "Device out"=w1879:refnum<class "Channel.lvclass">)  [unwired: 7 in]
          n672 = Equal?(x=w1883, y="DONE") -> (x = y?=w1881:bool)
          n673 = case shown="True" w1881 {
            tunnel: [w1886 w1887] -> w1880
            tunnel: w1877 -> [w1886 w1888]
            frame False {
            }
            frame True {
              n674 = Increment(x=w1888) -> (x+1=w1887:i32)
            }
          }
        }
        frame 226 {
          n675 = call-dynamic "Write cmd.vi"("error in (no error)"=w1894, "cmd"="GET PREAMP", "Device in"=w1892) -> ("error out"=w1893:errorcluster, "Device out"=w1895:refnum<class "Channel.lvclass">)  [unwired: 7 in]
          n676 = Increment(x=w1890) -> (x+1=w1891:i32)
        }
        frame 227 {
          n677 = call-dynamic "Read resp.vi"("error in (no error)"=w1906, "Device in"=w1907) -> ("error out"=w1904:errorcluster, "resp"=w1899:string, "Device out"=w1902:refnum<class "Channel.lvclass">)  [unwired: 7 in]
          n678 = Fract/Exp String To Number(string=w1899) -> (number=w1897:dbl)  [unwired: 3 in, 1 out]
          n679 = Unbundle By Name(w1902) -> ("Interface.lvclass"=w1901:refnum<class "Interface.lvclass">)
          n680 = call "Read Camera Setup.vi"("Interface in"=w1901) -> ("Camera Setup"=w1900:T3)  [unwired: 8 in, 2 out]
          n681 = Unbundle By Name(w1900) -> ("PREAMP"=w1896:u8)
          n682 = Equal?(x=w1896, y=w1897) -> (x = y?=w1898:bool)
          n683 = case shown="True" w1898 {
            tunnel: [w1908 w1909] -> w1905
            tunnel: w1903 -> [w1908 w1910]
            frame False {
            }
            frame True {
              n684 = Increment(x=w1910) -> (x+1=w1909:i32)
            }
          }
        }
        frame 228 {
          n685 = Unbundle By Name(w1919) -> ("Interface.lvclass"=w1918:refnum<class "Interface.lvclass">)
          n686 = call "Read Camera Setup.vi"("Interface in"=w1918) -> ("Camera Setup"=w1912:T3)  [unwired: 8 in, 2 out]
          n687 = Unbundle By Name(w1912) -> ("EM_MODE"=w1911:u8)
          n688 = Number To Fractional String(number=w1911) -> (F-format string=w1913:string)  [unwired: 3 in]
          n689 = Concatenate Strings("SET EM_MODE " ("cmd"), w1913) -> (w1917:string)
          n690 = call-dynamic "Write cmd.vi"("error in (no error)"=w1921, "cmd"=w1917, "Device in"=w1919) -> ("error out"=w1920:errorcluster, "Device out"=w1922:refnum<class "Channel.lvclass">)  [unwired: 7 in]
          n691 = Increment(x=w1915) -> (x+1=w1916:i32)
        }
        frame 229 {
          n692 = call-dynamic "Read resp.vi"("error in (no error)"=w1930, "Device in"=w1931) -> ("error out"=w1924:errorcluster, "resp"=w1929:string, "Device out"=w1925:refnum<class "Channel.lvclass">)  [unwired: 7 in]
          n693 = Equal?(x=w1929, y="DONE") -> (x = y?=w1927:bool)
          n694 = case shown="True" w1927 {
            tunnel: [w1932 w1933] -> w1926
            tunnel: w1923 -> [w1932 w1934]
            frame False {
            }
            frame True {
              n695 = Increment(x=w1934) -> (x+1=w1933:i32)
            }
          }
        }
        frame 230 {
          n696 = call-dynamic "Write cmd.vi"("error in (no error)"=w1940, "cmd"="GET EM_MODE", "Device in"=w1938) -> ("error out"=w1939:errorcluster, "Device out"=w1941:refnum<class "Channel.lvclass">)  [unwired: 7 in]
          n697 = Increment(x=w1936) -> (x+1=w1937:i32)
        }
        frame 231 {
          n698 = call-dynamic "Read resp.vi"("error in (no error)"=w1952, "Device in"=w1953) -> ("error out"=w1950:errorcluster, "resp"=w1945:string, "Device out"=w1948:refnum<class "Channel.lvclass">)  [unwired: 7 in]
          n699 = Fract/Exp String To Number(string=w1945) -> (number=w1943:dbl)  [unwired: 3 in, 1 out]
          n700 = Unbundle By Name(w1948) -> ("Interface.lvclass"=w1947:refnum<class "Interface.lvclass">)
          n701 = call "Read Camera Setup.vi"("Interface in"=w1947) -> ("Camera Setup"=w1946:T3)  [unwired: 8 in, 2 out]
          n702 = Unbundle By Name(w1946) -> ("EM_MODE"=w1942:u8)
          n703 = Equal?(x=w1942, y=w1943) -> (x = y?=w1944:bool)
          n704 = case shown="True" w1944 {
            tunnel: [w1954 w1955] -> w1951
            tunnel: w1949 -> [w1954 w1956]
            frame False {
            }
            frame True {
              n705 = Increment(x=w1956) -> (x+1=w1955:i32)
            }
          }
        }
        frame 232 {
          n706 = Unbundle By Name(w1965) -> ("Interface.lvclass"=w1964:refnum<class "Interface.lvclass">)
          n707 = call "Read Camera Setup.vi"("Interface in"=w1964) -> ("Camera Setup"=w1958:T3)  [unwired: 8 in, 2 out]
          n708 = Unbundle By Name(w1958) -> ("EM_GAIN"=w1957:u16)
          n709 = Number To Fractional String(number=w1957) -> (F-format string=w1959:string)  [unwired: 3 in]
          n710 = Concatenate Strings("SET EM_GAIN " ("cmd"), w1959) -> (w1963:string)
          n711 = call-dynamic "Write cmd.vi"("error in (no error)"=w1967, "cmd"=w1963, "Device in"=w1965) -> ("error out"=w1966:errorcluster, "Device out"=w1968:refnum<class "Channel.lvclass">)  [unwired: 7 in]
          n712 = Increment(x=w1961) -> (x+1=w1962:i32)
        }
        frame 233 {
          n713 = call-dynamic "Read resp.vi"("error in (no error)"=w1976, "Device in"=w1977) -> ("error out"=w1970:errorcluster, "resp"=w1975:string, "Device out"=w1971:refnum<class "Channel.lvclass">)  [unwired: 7 in]
          n714 = Equal?(x=w1975, y="DONE") -> (x = y?=w1973:bool)
          n715 = case shown="True" w1973 {
            tunnel: [w1978 w1979] -> w1972
            tunnel: w1969 -> [w1978 w1980]
            frame False {
            }
            frame True {
              n716 = Increment(x=w1980) -> (x+1=w1979:i32)
            }
          }
        }
        frame 234 {
          n717 = call-dynamic "Write cmd.vi"("error in (no error)"=w1986, "cmd"="GET EM_GAIN", "Device in"=w1984) -> ("error out"=w1985:errorcluster, "Device out"=w1987:refnum<class "Channel.lvclass">)  [unwired: 7 in]
          n718 = Increment(x=w1982) -> (x+1=w1983:i32)
        }
        frame 235 {
          n719 = call-dynamic "Read resp.vi"("error in (no error)"=w1998, "Device in"=w1999) -> ("error out"=w1996:errorcluster, "resp"=w1991:string, "Device out"=w1994:refnum<class "Channel.lvclass">)  [unwired: 7 in]
          n720 = Fract/Exp String To Number(string=w1991) -> (number=w1989:dbl)  [unwired: 3 in, 1 out]
          n721 = Unbundle By Name(w1994) -> ("Interface.lvclass"=w1993:refnum<class "Interface.lvclass">)
          n722 = call "Read Camera Setup.vi"("Interface in"=w1993) -> ("Camera Setup"=w1992:T3)  [unwired: 8 in, 2 out]
          n723 = Unbundle By Name(w1992) -> ("EM_GAIN"=w1988:u16)
          n724 = Equal?(x=w1988, y=w1989) -> (x = y?=w1990:bool)
          n725 = disable-structure shown="Enabled" {
            disable-tunnel: [w2002 264 ("State")] -> w1997
            disable-tunnel: w1995 -> [w2001 _]
            disable-tunnel: w1990 -> [w2000 _]
            frame Disabled {
              n726 = case shown="True" w2000 {
                tunnel: [w2003 w2004] -> w2002
                tunnel: w2001 -> [w2003 w2005]
                frame False {
                }
                frame True {
                  n727 = Increment(x=w2005) -> (x+1=w2004:i32)
                }
              }
            }
            frame Enabled {
            }
          }
        }
        frame 236 {
          n728 = Unbundle By Name(w2015) -> ("Interface.lvclass"=w2014:refnum<class "Interface.lvclass">)
          n729 = call "Read Camera Setup.vi"("Interface in"=w2014) -> ("Camera Setup"=w2008:T3)  [unwired: 8 in, 2 out]
          n730 = Unbundle By Name(w2008) -> ("ACQUISITION_MODE"=w2007:u8)
          n731 = Number To Fractional String(number=w2007) -> (F-format string=w2009:string)  [unwired: 3 in]
          n732 = Concatenate Strings("SET ACQUISITION_MODE " ("cmd"), w2009) -> (w2013:string)
          n733 = call-dynamic "Write cmd.vi"("error in (no error)"=w2017, "cmd"=w2013, "Device in"=w2015) -> ("error out"=w2016:errorcluster, "Device out"=w2018:refnum<class "Channel.lvclass">)  [unwired: 7 in]
          n734 = Increment(x=w2011) -> (x+1=w2012:i32)
        }
        frame 237 {
          n735 = call-dynamic "Read resp.vi"("error in (no error)"=w2026, "Device in"=w2027) -> ("error out"=w2020:errorcluster, "resp"=w2025:string, "Device out"=w2021:refnum<class "Channel.lvclass">)  [unwired: 7 in]
          n736 = Equal?(x=w2025, y="DONE") -> (x = y?=w2023:bool)
          n737 = case shown="True" w2023 {
            tunnel: [w2028 w2029] -> w2022
            tunnel: w2019 -> [w2028 w2030]
            frame False {
            }
            frame True {
              n738 = Increment(x=w2030) -> (x+1=w2029:i32)
            }
          }
        }
        frame 238 {
          n739 = call-dynamic "Write cmd.vi"("error in (no error)"=w2036, "cmd"="GET ACQUISITION_MODE", "Device in"=w2034) -> ("error out"=w2035:errorcluster, "Device out"=w2037:refnum<class "Channel.lvclass">)  [unwired: 7 in]
          n740 = Increment(x=w2032) -> (x+1=w2033:i32)
        }
        frame 239 {
          n741 = call-dynamic "Read resp.vi"("error in (no error)"=w2048, "Device in"=w2049) -> ("error out"=w2046:errorcluster, "resp"=w2041:string, "Device out"=w2044:refnum<class "Channel.lvclass">)  [unwired: 7 in]
          n742 = Fract/Exp String To Number(string=w2041) -> (number=w2039:dbl)  [unwired: 3 in, 1 out]
          n743 = Unbundle By Name(w2044) -> ("Interface.lvclass"=w2043:refnum<class "Interface.lvclass">)
          n744 = call "Read Camera Setup.vi"("Interface in"=w2043) -> ("Camera Setup"=w2042:T3)  [unwired: 8 in, 2 out]
          n745 = Unbundle By Name(w2042) -> ("ACQUISITION_MODE"=w2038:u8)
          n746 = Equal?(x=w2038, y=w2039) -> (x = y?=w2040:bool)
          n747 = case shown="True" w2040 {
            tunnel: [w2050 w2051] -> w2047
            tunnel: w2045 -> [w2050 w2052]
            frame False {
            }
            frame True {
              n748 = Increment(x=w2052) -> (x+1=w2051:i32)
            }
          }
        }
        frame 240 {
          n749 = Unbundle By Name(w2061) -> ("Interface.lvclass"=w2060:refnum<class "Interface.lvclass">)
          n750 = call "Read Camera Setup.vi"("Interface in"=w2060) -> ("Camera Setup"=w2054:T3)  [unwired: 8 in, 2 out]
          n751 = Unbundle By Name(w2054) -> ("SHUTTER_MODE"=w2053:u8)
          n752 = Number To Fractional String(number=w2053) -> (F-format string=w2055:string)  [unwired: 3 in]
          n753 = Concatenate Strings("SET SHUTTER_MODE " ("cmd"), w2055) -> (w2059:string)
          n754 = call-dynamic "Write cmd.vi"("error in (no error)"=w2063, "cmd"=w2059, "Device in"=w2061) -> ("error out"=w2062:errorcluster, "Device out"=w2064:refnum<class "Channel.lvclass">)  [unwired: 7 in]
          n755 = Increment(x=w2057) -> (x+1=w2058:i32)
        }
        frame 241 {
          n756 = call-dynamic "Read resp.vi"("error in (no error)"=w2072, "Device in"=w2073) -> ("error out"=w2066:errorcluster, "resp"=w2071:string, "Device out"=w2067:refnum<class "Channel.lvclass">)  [unwired: 7 in]
          n757 = Equal?(x=w2071, y="DONE") -> (x = y?=w2069:bool)
          n758 = case shown="True" w2069 {
            tunnel: [w2074 w2075] -> w2068
            tunnel: w2065 -> [w2074 w2076]
            frame False {
            }
            frame True {
              n759 = Increment(x=w2076) -> (x+1=w2075:i32)
            }
          }
        }
        frame 242 {
          n760 = call-dynamic "Write cmd.vi"("error in (no error)"=w2082, "cmd"="GET SHUTTER_MODE", "Device in"=w2080) -> ("error out"=w2081:errorcluster, "Device out"=w2083:refnum<class "Channel.lvclass">)  [unwired: 7 in]
          n761 = Increment(x=w2078) -> (x+1=w2079:i32)
        }
        frame 243 {
          n762 = call-dynamic "Read resp.vi"("error in (no error)"=w2094, "Device in"=w2095) -> ("error out"=w2092:errorcluster, "resp"=w2087:string, "Device out"=w2090:refnum<class "Channel.lvclass">)  [unwired: 7 in]
          n763 = Fract/Exp String To Number(string=w2087) -> (number=w2085:dbl)  [unwired: 3 in, 1 out]
          n764 = Unbundle By Name(w2090) -> ("Interface.lvclass"=w2089:refnum<class "Interface.lvclass">)
          n765 = call "Read Camera Setup.vi"("Interface in"=w2089) -> ("Camera Setup"=w2088:T3)  [unwired: 8 in, 2 out]
          n766 = Unbundle By Name(w2088) -> ("SHUTTER_MODE"=w2084:u8)
          n767 = Equal?(x=w2084, y=w2085) -> (x = y?=w2086:bool)
          n768 = case shown="True" w2086 {
            tunnel: [w2096 w2097] -> w2093
            tunnel: w2091 -> [w2096 w2098]
            frame False {
            }
            frame True {
              n769 = Increment(x=w2098) -> (x+1=w2097:i32)
            }
          }
        }
        frame 244 {
          n770 = Unbundle By Name(w2107) -> ("Interface.lvclass"=w2106:refnum<class "Interface.lvclass">)
          n771 = call "Read Camera Setup.vi"("Interface in"=w2106) -> ("Camera Setup"=w2100:T3)  [unwired: 8 in, 2 out]
          n772 = Unbundle By Name(w2100) -> ("SHUTTER_TTL"=w2099:u8)
          n773 = Number To Fractional String(number=w2099) -> (F-format string=w2101:string)  [unwired: 3 in]
          n774 = Concatenate Strings("SET SHUTTER_TTL " ("cmd"), w2101) -> (w2105:string)
          n775 = call-dynamic "Write cmd.vi"("error in (no error)"=w2109, "cmd"=w2105, "Device in"=w2107) -> ("error out"=w2108:errorcluster, "Device out"=w2110:refnum<class "Channel.lvclass">)  [unwired: 7 in]
          n776 = Increment(x=w2103) -> (x+1=w2104:i32)
        }
        frame 245 {
          n777 = call-dynamic "Read resp.vi"("error in (no error)"=w2118, "Device in"=w2119) -> ("error out"=w2112:errorcluster, "resp"=w2117:string, "Device out"=w2113:refnum<class "Channel.lvclass">)  [unwired: 7 in]
          n778 = Equal?(x=w2117, y="DONE") -> (x = y?=w2115:bool)
          n779 = case shown="True" w2115 {
            tunnel: [w2120 w2121] -> w2114
            tunnel: w2111 -> [w2120 w2122]
            frame False {
            }
            frame True {
              n780 = Increment(x=w2122) -> (x+1=w2121:i32)
            }
          }
        }
        frame 246 {
          n781 = call-dynamic "Write cmd.vi"("error in (no error)"=w2128, "cmd"="GET SHUTTER_TTL", "Device in"=w2126) -> ("error out"=w2127:errorcluster, "Device out"=w2129:refnum<class "Channel.lvclass">)  [unwired: 7 in]
          n782 = Increment(x=w2124) -> (x+1=w2125:i32)
        }
        frame 247 {
          n783 = call-dynamic "Read resp.vi"("error in (no error)"=w2140, "Device in"=w2141) -> ("error out"=w2138:errorcluster, "resp"=w2133:string, "Device out"=w2136:refnum<class "Channel.lvclass">)  [unwired: 7 in]
          n784 = Fract/Exp String To Number(string=w2133) -> (number=w2131:dbl)  [unwired: 3 in, 1 out]
          n785 = Unbundle By Name(w2136) -> ("Interface.lvclass"=w2135:refnum<class "Interface.lvclass">)
          n786 = call "Read Camera Setup.vi"("Interface in"=w2135) -> ("Camera Setup"=w2134:T3)  [unwired: 8 in, 2 out]
          n787 = Unbundle By Name(w2134) -> ("SHUTTER_TTL"=w2130:u8)
          n788 = Equal?(x=w2130, y=w2131) -> (x = y?=w2132:bool)
          n789 = case shown="True" w2132 {
            tunnel: [w2142 w2143] -> w2139
            tunnel: w2137 -> [w2142 w2144]
            frame False {
            }
            frame True {
              n790 = Increment(x=w2144) -> (x+1=w2143:i32)
            }
          }
        }
        frame 248 {
          n791 = Unbundle By Name(w2153) -> ("Interface.lvclass"=w2152:refnum<class "Interface.lvclass">)
          n792 = call "Read Camera Setup.vi"("Interface in"=w2152) -> ("Camera Setup"=w2146:T3)  [unwired: 8 in, 2 out]
          n793 = Unbundle By Name(w2146) -> ("SHUTTER_OPENNING_TIME"=w2145:u16)
          n794 = Number To Fractional String(number=w2145) -> (F-format string=w2147:string)  [unwired: 3 in]
          n795 = Concatenate Strings("SET SHUTTER_OPENNING_TIME " ("cmd"), w2147) -> (w2151:string)
          n796 = call-dynamic "Write cmd.vi"("error in (no error)"=w2155, "cmd"=w2151, "Device in"=w2153) -> ("error out"=w2154:errorcluster, "Device out"=w2156:refnum<class "Channel.lvclass">)  [unwired: 7 in]
          n797 = Increment(x=w2149) -> (x+1=w2150:i32)
        }
        frame 249 {
          n798 = call-dynamic "Read resp.vi"("error in (no error)"=w2164, "Device in"=w2165) -> ("error out"=w2158:errorcluster, "resp"=w2163:string, "Device out"=w2159:refnum<class "Channel.lvclass">)  [unwired: 7 in]
          n799 = Equal?(x=w2163, y="DONE") -> (x = y?=w2161:bool)
          n800 = case shown="True" w2161 {
            tunnel: [w2166 w2167] -> w2160
            tunnel: w2157 -> [w2166 w2168]
            frame False {
            }
            frame True {
              n801 = Increment(x=w2168) -> (x+1=w2167:i32)
            }
          }
        }
        frame 250 {
          n802 = call-dynamic "Write cmd.vi"("error in (no error)"=w2174, "cmd"="GET SHUTTER_OPENNING_TIME", "Device in"=w2172) -> ("error out"=w2173:errorcluster, "Device out"=w2175:refnum<class "Channel.lvclass">)  [unwired: 7 in]
          n803 = Increment(x=w2170) -> (x+1=w2171:i32)
        }
        frame 251 {
          n804 = call-dynamic "Read resp.vi"("error in (no error)"=w2186, "Device in"=w2187) -> ("error out"=w2184:errorcluster, "resp"=w2179:string, "Device out"=w2182:refnum<class "Channel.lvclass">)  [unwired: 7 in]
          n805 = Fract/Exp String To Number(string=w2179) -> (number=w2177:dbl)  [unwired: 3 in, 1 out]
          n806 = Unbundle By Name(w2182) -> ("Interface.lvclass"=w2181:refnum<class "Interface.lvclass">)
          n807 = call "Read Camera Setup.vi"("Interface in"=w2181) -> ("Camera Setup"=w2180:T3)  [unwired: 8 in, 2 out]
          n808 = Unbundle By Name(w2180) -> ("SHUTTER_OPENNING_TIME"=w2176:u16)
          n809 = Equal?(x=w2176, y=w2177) -> (x = y?=w2178:bool)
          n810 = case shown="True" w2178 {
            tunnel: [w2188 w2189] -> w2185
            tunnel: w2183 -> [w2188 w2190]
            frame False {
            }
            frame True {
              n811 = Increment(x=w2190) -> (x+1=w2189:i32)
            }
          }
        }
        frame 252 {
          n812 = Unbundle By Name(w2199) -> ("Interface.lvclass"=w2198:refnum<class "Interface.lvclass">)
          n813 = call "Read Camera Setup.vi"("Interface in"=w2198) -> ("Camera Setup"=w2192:T3)  [unwired: 8 in, 2 out]
          n814 = Unbundle By Name(w2192) -> ("SHUTTER_CLOSING_TIME"=w2191:u16)
          n815 = Number To Fractional String(number=w2191) -> (F-format string=w2193:string)  [unwired: 3 in]
          n816 = Concatenate Strings("SET SHUTTER_CLOSING_TIME " ("cmd"), w2193) -> (w2197:string)
          n817 = call-dynamic "Write cmd.vi"("error in (no error)"=w2201, "cmd"=w2197, "Device in"=w2199) -> ("error out"=w2200:errorcluster, "Device out"=w2202:refnum<class "Channel.lvclass">)  [unwired: 7 in]
          n818 = Increment(x=w2195) -> (x+1=w2196:i32)
        }
        frame 253 {
          n819 = call-dynamic "Read resp.vi"("error in (no error)"=w2210, "Device in"=w2211) -> ("error out"=w2204:errorcluster, "resp"=w2209:string, "Device out"=w2205:refnum<class "Channel.lvclass">)  [unwired: 7 in]
          n820 = Equal?(x=w2209, y="DONE") -> (x = y?=w2207:bool)
          n821 = case shown="True" w2207 {
            tunnel: [w2212 w2213] -> w2206
            tunnel: w2203 -> [w2212 w2214]
            frame False {
            }
            frame True {
              n822 = Increment(x=w2214) -> (x+1=w2213:i32)
            }
          }
        }
        frame 254 {
          n823 = call-dynamic "Write cmd.vi"("error in (no error)"=w2220, "cmd"="GET SHUTTER_CLOSING_TIME", "Device in"=w2218) -> ("error out"=w2219:errorcluster, "Device out"=w2221:refnum<class "Channel.lvclass">)  [unwired: 7 in]
          n824 = Increment(x=w2216) -> (x+1=w2217:i32)
        }
        frame 255 {
          n825 = call-dynamic "Read resp.vi"("error in (no error)"=w2232, "Device in"=w2233) -> ("error out"=w2230:errorcluster, "resp"=w2225:string, "Device out"=w2228:refnum<class "Channel.lvclass">)  [unwired: 7 in]
          n826 = Fract/Exp String To Number(string=w2225) -> (number=w2223:dbl)  [unwired: 3 in, 1 out]
          n827 = Unbundle By Name(w2228) -> ("Interface.lvclass"=w2227:refnum<class "Interface.lvclass">)
          n828 = call "Read Camera Setup.vi"("Interface in"=w2227) -> ("Camera Setup"=w2226:T3)  [unwired: 8 in, 2 out]
          n829 = Unbundle By Name(w2226) -> ("SHUTTER_CLOSING_TIME"=w2222:u16)
          n830 = Equal?(x=w2222, y=w2223) -> (x = y?=w2224:bool)
          n831 = case shown="True" w2224 {
            tunnel: [w2234 w2235] -> w2231
            tunnel: w2229 -> [w2234 w2236]
            frame False {
            }
            frame True {
              n832 = Increment(x=w2236) -> (x+1=w2235:i32)
            }
          }
        }
        frame 256 {
          n833 = Unbundle By Name(w2245) -> ("Interface.lvclass"=w2244:refnum<class "Interface.lvclass">)
          n834 = call "Read Camera Setup.vi"("Interface in"=w2244) -> ("Camera Setup"=w2238:T3)  [unwired: 8 in, 2 out]
          n835 = Unbundle By Name(w2238) -> ("HBIN"=w2237:u16)
          n836 = Number To Fractional String(number=w2237) -> (F-format string=w2239:string)  [unwired: 3 in]
          n837 = Concatenate Strings("SET HBIN " ("cmd"), w2239) -> (w2243:string)
          n838 = call-dynamic "Write cmd.vi"("error in (no error)"=w2247, "cmd"=w2243, "Device in"=w2245) -> ("error out"=w2246:errorcluster, "Device out"=w2248:refnum<class "Channel.lvclass">)  [unwired: 7 in]
          n839 = Increment(x=w2241) -> (x+1=w2242:i32)
        }
        frame 257 {
          n840 = call-dynamic "Read resp.vi"("error in (no error)"=w2256, "Device in"=w2257) -> ("error out"=w2250:errorcluster, "resp"=w2255:string, "Device out"=w2251:refnum<class "Channel.lvclass">)  [unwired: 7 in]
          n841 = Equal?(x=w2255, y="DONE") -> (x = y?=w2253:bool)
          n842 = case shown="True" w2253 {
            tunnel: [w2258 w2259] -> w2252
            tunnel: w2249 -> [w2258 w2260]
            frame False {
            }
            frame True {
              n843 = Increment(x=w2260) -> (x+1=w2259:i32)
            }
          }
        }
        frame 258 {
          n844 = call-dynamic "Write cmd.vi"("error in (no error)"=w2266, "cmd"="GET HBIN", "Device in"=w2264) -> ("error out"=w2265:errorcluster, "Device out"=w2267:refnum<class "Channel.lvclass">)  [unwired: 7 in]
          n845 = Increment(x=w2262) -> (x+1=w2263:i32)
        }
        frame 259 {
          n846 = call-dynamic "Read resp.vi"("error in (no error)"=w2278, "Device in"=w2279) -> ("error out"=w2276:errorcluster, "resp"=w2271:string, "Device out"=w2274:refnum<class "Channel.lvclass">)  [unwired: 7 in]
          n847 = Fract/Exp String To Number(string=w2271) -> (number=w2269:dbl)  [unwired: 3 in, 1 out]
          n848 = Unbundle By Name(w2274) -> ("Interface.lvclass"=w2273:refnum<class "Interface.lvclass">)
          n849 = call "Read Camera Setup.vi"("Interface in"=w2273) -> ("Camera Setup"=w2272:T3)  [unwired: 8 in, 2 out]
          n850 = Unbundle By Name(w2272) -> ("HBIN"=w2268:u16)
          n851 = Equal?(x=w2268, y=w2269) -> (x = y?=w2270:bool)
          n852 = case shown="True" w2270 {
            tunnel: [w2280 w2281] -> w2277
            tunnel: w2275 -> [w2280 w2282]
            frame False {
            }
            frame True {
              n853 = Increment(x=w2282) -> (x+1=w2281:i32)
            }
          }
        }
        frame 260 {
          n854 = Unbundle By Name(w2291) -> ("Interface.lvclass"=w2290:refnum<class "Interface.lvclass">)
          n855 = call "Read Camera Setup.vi"("Interface in"=w2290) -> ("Camera Setup"=w2284:T3)  [unwired: 8 in, 2 out]
          n856 = Unbundle By Name(w2284) -> ("VBIN"=w2283:u16)
          n857 = Number To Fractional String(number=w2283) -> (F-format string=w2285:string)  [unwired: 3 in]
          n858 = Concatenate Strings("SET VBIN " ("cmd"), w2285) -> (w2289:string)
          n859 = call-dynamic "Write cmd.vi"("error in (no error)"=w2293, "cmd"=w2289, "Device in"=w2291) -> ("error out"=w2292:errorcluster, "Device out"=w2294:refnum<class "Channel.lvclass">)  [unwired: 7 in]
          n860 = Increment(x=w2287) -> (x+1=w2288:i32)
        }
        frame 261 {
          n861 = call-dynamic "Read resp.vi"("error in (no error)"=w2302, "Device in"=w2303) -> ("error out"=w2296:errorcluster, "resp"=w2301:string, "Device out"=w2297:refnum<class "Channel.lvclass">)  [unwired: 7 in]
          n862 = Equal?(x=w2301, y="DONE") -> (x = y?=w2299:bool)
          n863 = case shown="True" w2299 {
            tunnel: [w2304 w2305] -> w2298
            tunnel: w2295 -> [w2304 w2306]
            frame False {
            }
            frame True {
              n864 = Increment(x=w2306) -> (x+1=w2305:i32)
            }
          }
        }
        frame 262 {
          n865 = call-dynamic "Write cmd.vi"("error in (no error)"=w2312, "cmd"="GET VBIN", "Device in"=w2310) -> ("error out"=w2311:errorcluster, "Device out"=w2313:refnum<class "Channel.lvclass">)  [unwired: 7 in]
          n866 = Increment(x=w2308) -> (x+1=w2309:i32)
        }
        frame 263 {
          n867 = call-dynamic "Read resp.vi"("error in (no error)"=w2324, "Device in"=w2325) -> ("error out"=w2322:errorcluster, "resp"=w2317:string, "Device out"=w2320:refnum<class "Channel.lvclass">)  [unwired: 7 in]
          n868 = Fract/Exp String To Number(string=w2317) -> (number=w2315:dbl)  [unwired: 3 in, 1 out]
          n869 = Unbundle By Name(w2320) -> ("Interface.lvclass"=w2319:refnum<class "Interface.lvclass">)
          n870 = call "Read Camera Setup.vi"("Interface in"=w2319) -> ("Camera Setup"=w2318:T3)  [unwired: 8 in, 2 out]
          n871 = Unbundle By Name(w2318) -> ("VBIN"=w2314:u16)
          n872 = Equal?(x=w2314, y=w2315) -> (x = y?=w2316:bool)
          n873 = case shown="True" w2316 {
            tunnel: [w2326 w2327] -> w2323
            tunnel: w2321 -> [w2326 w2328]
            frame False {
            }
            frame True {
              n874 = Increment(x=w2328) -> (x+1=w2327:i32)
            }
          }
        }
        frame 264 {
          n875 = Unbundle By Name(w2337) -> ("Interface.lvclass"=w2336:refnum<class "Interface.lvclass">)
          n876 = call "Read Camera Setup.vi"("Interface in"=w2336) -> ("Camera Setup"=w2330:T3)  [unwired: 8 in, 2 out]
          n877 = Unbundle By Name(w2330) -> ("INITIAL_LINE"=w2329:u16)
          n878 = Number To Fractional String(number=w2329) -> (F-format string=w2331:string)  [unwired: 3 in]
          n879 = Concatenate Strings("SET INITIAL_LINE " ("cmd"), w2331) -> (w2335:string)
          n880 = call-dynamic "Write cmd.vi"("error in (no error)"=w2339, "cmd"=w2335, "Device in"=w2337) -> ("error out"=w2338:errorcluster, "Device out"=w2340:refnum<class "Channel.lvclass">)  [unwired: 7 in]
          n881 = Increment(x=w2333) -> (x+1=w2334:i32)
        }
        frame 265 {
          n882 = call-dynamic "Read resp.vi"("error in (no error)"=w2348, "Device in"=w2349) -> ("error out"=w2342:errorcluster, "resp"=w2347:string, "Device out"=w2343:refnum<class "Channel.lvclass">)  [unwired: 7 in]
          n883 = Equal?(x=w2347, y="DONE") -> (x = y?=w2345:bool)
          n884 = case shown="True" w2345 {
            tunnel: [w2350 w2351] -> w2344
            tunnel: w2341 -> [w2350 w2352]
            frame False {
            }
            frame True {
              n885 = Increment(x=w2352) -> (x+1=w2351:i32)
            }
          }
        }
        frame 266 {
          n886 = call-dynamic "Write cmd.vi"("error in (no error)"=w2358, "cmd"="GET INITIAL_LINE", "Device in"=w2356) -> ("error out"=w2357:errorcluster, "Device out"=w2359:refnum<class "Channel.lvclass">)  [unwired: 7 in]
          n887 = Increment(x=w2354) -> (x+1=w2355:i32)
        }
        frame 267 {
          n888 = call-dynamic "Read resp.vi"("error in (no error)"=w2370, "Device in"=w2371) -> ("error out"=w2368:errorcluster, "resp"=w2363:string, "Device out"=w2366:refnum<class "Channel.lvclass">)  [unwired: 7 in]
          n889 = Fract/Exp String To Number(string=w2363) -> (number=w2361:dbl)  [unwired: 3 in, 1 out]
          n890 = Unbundle By Name(w2366) -> ("Interface.lvclass"=w2365:refnum<class "Interface.lvclass">)
          n891 = call "Read Camera Setup.vi"("Interface in"=w2365) -> ("Camera Setup"=w2364:T3)  [unwired: 8 in, 2 out]
          n892 = Unbundle By Name(w2364) -> ("INITIAL_LINE"=w2360:u16)
          n893 = Equal?(x=w2360, y=w2361) -> (x = y?=w2362:bool)
          n894 = case shown="True" w2362 {
            tunnel: [w2372 w2373] -> w2369
            tunnel: w2367 -> [w2372 w2374]
            frame False {
            }
            frame True {
              n895 = Increment(x=w2374) -> (x+1=w2373:i32)
            }
          }
        }
        frame 268 {
          n896 = Unbundle By Name(w2383) -> ("Interface.lvclass"=w2382:refnum<class "Interface.lvclass">)
          n897 = call "Read Camera Setup.vi"("Interface in"=w2382) -> ("Camera Setup"=w2376:T3)  [unwired: 8 in, 2 out]
          n898 = Unbundle By Name(w2376) -> ("INITIAL_COLUMN"=w2375:u16)
          n899 = Number To Fractional String(number=w2375) -> (F-format string=w2377:string)  [unwired: 3 in]
          n900 = Concatenate Strings("SET INITIAL_COLUMN " ("cmd"), w2377) -> (w2381:string)
          n901 = call-dynamic "Write cmd.vi"("error in (no error)"=w2385, "cmd"=w2381, "Device in"=w2383) -> ("error out"=w2384:errorcluster, "Device out"=w2386:refnum<class "Channel.lvclass">)  [unwired: 7 in]
          n902 = Increment(x=w2379) -> (x+1=w2380:i32)
        }
        frame 269 {
          n903 = call-dynamic "Read resp.vi"("error in (no error)"=w2394, "Device in"=w2395) -> ("error out"=w2388:errorcluster, "resp"=w2393:string, "Device out"=w2389:refnum<class "Channel.lvclass">)  [unwired: 7 in]
          n904 = Equal?(x=w2393, y="DONE") -> (x = y?=w2391:bool)
          n905 = case shown="True" w2391 {
            tunnel: [w2396 w2397] -> w2390
            tunnel: w2387 -> [w2396 w2398]
            frame False {
            }
            frame True {
              n906 = Increment(x=w2398) -> (x+1=w2397:i32)
            }
          }
        }
        frame 270 {
          n907 = call-dynamic "Write cmd.vi"("error in (no error)"=w2404, "cmd"="GET INITIAL_COLUMN", "Device in"=w2402) -> ("error out"=w2403:errorcluster, "Device out"=w2405:refnum<class "Channel.lvclass">)  [unwired: 7 in]
          n908 = Increment(x=w2400) -> (x+1=w2401:i32)
        }
        frame 271 {
          n909 = call-dynamic "Read resp.vi"("error in (no error)"=w2416, "Device in"=w2417) -> ("error out"=w2414:errorcluster, "resp"=w2409:string, "Device out"=w2412:refnum<class "Channel.lvclass">)  [unwired: 7 in]
          n910 = Fract/Exp String To Number(string=w2409) -> (number=w2407:dbl)  [unwired: 3 in, 1 out]
          n911 = Unbundle By Name(w2412) -> ("Interface.lvclass"=w2411:refnum<class "Interface.lvclass">)
          n912 = call "Read Camera Setup.vi"("Interface in"=w2411) -> ("Camera Setup"=w2410:T3)  [unwired: 8 in, 2 out]
          n913 = Unbundle By Name(w2410) -> ("INITIAL_COLUMN"=w2406:u16)
          n914 = Equal?(x=w2406, y=w2407) -> (x = y?=w2408:bool)
          n915 = case shown="True" w2408 {
            tunnel: [w2418 w2419] -> w2415
            tunnel: w2413 -> [w2418 w2420]
            frame False {
            }
            frame True {
              n916 = Increment(x=w2420) -> (x+1=w2419:i32)
            }
          }
        }
        frame 272 {
          n917 = Unbundle By Name(w2429) -> ("Interface.lvclass"=w2428:refnum<class "Interface.lvclass">)
          n918 = call "Read Camera Setup.vi"("Interface in"=w2428) -> ("Camera Setup"=w2422:T3)  [unwired: 8 in, 2 out]
          n919 = Unbundle By Name(w2422) -> ("FINAL_LINE"=w2421:u16)
          n920 = Number To Fractional String(number=w2421) -> (F-format string=w2423:string)  [unwired: 3 in]
          n921 = Concatenate Strings("SET FINAL_LINE " ("cmd"), w2423) -> (w2427:string)
          n922 = call-dynamic "Write cmd.vi"("error in (no error)"=w2431, "cmd"=w2427, "Device in"=w2429) -> ("error out"=w2430:errorcluster, "Device out"=w2432:refnum<class "Channel.lvclass">)  [unwired: 7 in]
          n923 = Increment(x=w2425) -> (x+1=w2426:i32)
        }
        frame 273 {
          n924 = call-dynamic "Read resp.vi"("error in (no error)"=w2440, "Device in"=w2441) -> ("error out"=w2434:errorcluster, "resp"=w2439:string, "Device out"=w2435:refnum<class "Channel.lvclass">)  [unwired: 7 in]
          n925 = Equal?(x=w2439, y="DONE") -> (x = y?=w2437:bool)
          n926 = case shown="True" w2437 {
            tunnel: [w2442 w2443] -> w2436
            tunnel: w2433 -> [w2442 w2444]
            frame False {
            }
            frame True {
              n927 = Increment(x=w2444) -> (x+1=w2443:i32)
            }
          }
        }
        frame 274 {
          n928 = call-dynamic "Write cmd.vi"("error in (no error)"=w2450, "cmd"="GET FINAL_LINE", "Device in"=w2448) -> ("error out"=w2449:errorcluster, "Device out"=w2451:refnum<class "Channel.lvclass">)  [unwired: 7 in]
          n929 = Increment(x=w2446) -> (x+1=w2447:i32)
        }
        frame 275 {
          n930 = call-dynamic "Read resp.vi"("error in (no error)"=w2462, "Device in"=w2463) -> ("error out"=w2460:errorcluster, "resp"=w2455:string, "Device out"=w2458:refnum<class "Channel.lvclass">)  [unwired: 7 in]
          n931 = Fract/Exp String To Number(string=w2455) -> (number=w2453:dbl)  [unwired: 3 in, 1 out]
          n932 = Unbundle By Name(w2458) -> ("Interface.lvclass"=w2457:refnum<class "Interface.lvclass">)
          n933 = call "Read Camera Setup.vi"("Interface in"=w2457) -> ("Camera Setup"=w2456:T3)  [unwired: 8 in, 2 out]
          n934 = Unbundle By Name(w2456) -> ("FINAL_LINE"=w2452:u16)
          n935 = Equal?(x=w2452, y=w2453) -> (x = y?=w2454:bool)
          n936 = case shown="True" w2454 {
            tunnel: [w2464 w2465] -> w2461
            tunnel: w2459 -> [w2464 w2466]
            frame False {
            }
            frame True {
              n937 = Increment(x=w2466) -> (x+1=w2465:i32)
            }
          }
        }
        frame 276 {
          n938 = Unbundle By Name(w2475) -> ("Interface.lvclass"=w2474:refnum<class "Interface.lvclass">)
          n939 = call "Read Camera Setup.vi"("Interface in"=w2474) -> ("Camera Setup"=w2468:T3)  [unwired: 8 in, 2 out]
          n940 = Unbundle By Name(w2468) -> ("FINAL_COLUMN"=w2467:u16)
          n941 = Number To Fractional String(number=w2467) -> (F-format string=w2469:string)  [unwired: 3 in]
          n942 = Concatenate Strings("SET FINAL_COLUMN " ("cmd"), w2469) -> (w2473:string)
          n943 = call-dynamic "Write cmd.vi"("error in (no error)"=w2477, "cmd"=w2473, "Device in"=w2475) -> ("error out"=w2476:errorcluster, "Device out"=w2478:refnum<class "Channel.lvclass">)  [unwired: 7 in]
          n944 = Increment(x=w2471) -> (x+1=w2472:i32)
        }
        frame 277 {
          n945 = call-dynamic "Read resp.vi"("error in (no error)"=w2486, "Device in"=w2487) -> ("error out"=w2480:errorcluster, "resp"=w2485:string, "Device out"=w2481:refnum<class "Channel.lvclass">)  [unwired: 7 in]
          n946 = Equal?(x=w2485, y="DONE") -> (x = y?=w2483:bool)
          n947 = case shown="True" w2483 {
            tunnel: [w2488 w2489] -> w2482
            tunnel: w2479 -> [w2488 w2490]
            frame False {
            }
            frame True {
              n948 = Increment(x=w2490) -> (x+1=w2489:i32)
            }
          }
        }
        frame 278 {
          n949 = call-dynamic "Write cmd.vi"("error in (no error)"=w2496, "cmd"="GET FINAL_COLUMN", "Device in"=w2494) -> ("error out"=w2495:errorcluster, "Device out"=w2497:refnum<class "Channel.lvclass">)  [unwired: 7 in]
          n950 = Increment(x=w2492) -> (x+1=w2493:i32)
        }
        frame 279 {
          n951 = call-dynamic "Read resp.vi"("error in (no error)"=w2508, "Device in"=w2509) -> ("error out"=w2506:errorcluster, "resp"=w2501:string, "Device out"=w2504:refnum<class "Channel.lvclass">)  [unwired: 7 in]
          n952 = Fract/Exp String To Number(string=w2501) -> (number=w2499:dbl)  [unwired: 3 in, 1 out]
          n953 = Unbundle By Name(w2504) -> ("Interface.lvclass"=w2503:refnum<class "Interface.lvclass">)
          n954 = call "Read Camera Setup.vi"("Interface in"=w2503) -> ("Camera Setup"=w2502:T3)  [unwired: 8 in, 2 out]
          n955 = Unbundle By Name(w2502) -> ("FINAL_COLUMN"=w2498:u16)
          n956 = Equal?(x=w2498, y=w2499) -> (x = y?=w2500:bool)
          n957 = disable-structure shown="Enabled" {
            disable-tunnel: [w2512 0 ("State")] -> w2507
            disable-tunnel: w2505 -> [w2511 _]
            disable-tunnel: w2500 -> [w2510 _]
            frame Disabled {
              n958 = case shown="True" w2510 {
                tunnel: [w2513 w2514] -> w2512
                tunnel: w2511 -> [w2513 w2515]
                frame False {
                }
                frame True {
                  n959 = Increment(x=w2515) -> (x+1=w2514:i32)
                }
              }
            }
            frame Enabled {
            }
          }
        }
        frame 280 {
          n960 = Unbundle By Name(w2525) -> ("Interface.lvclass"=w2524:refnum<class "Interface.lvclass">)
          n961 = call "Read Camera Setup.vi"("Interface in"=w2524) -> ("Camera Setup"=w2518:T3)  [unwired: 8 in, 2 out]
          n962 = Unbundle By Name(w2518) -> ("VERTICAL_CLOCK_VOLTAGE"=w2517:u8)
          n963 = Number To Fractional String(number=w2517) -> (F-format string=w2519:string)  [unwired: 3 in]
          n964 = Concatenate Strings("SET VERTICAL_CLOCK_VOLTAGE " ("cmd"), w2519) -> (w2523:string)
          n965 = call-dynamic "Write cmd.vi"("error in (no error)"=w2527, "cmd"=w2523, "Device in"=w2525) -> ("error out"=w2526:errorcluster, "Device out"=w2528:refnum<class "Channel.lvclass">)  [unwired: 7 in]
          n966 = Increment(x=w2521) -> (x+1=w2522:i32)
        }
        frame 281 {
          n967 = call-dynamic "Read resp.vi"("error in (no error)"=w2536, "Device in"=w2537) -> ("error out"=w2530:errorcluster, "resp"=w2535:string, "Device out"=w2531:refnum<class "Channel.lvclass">)  [unwired: 7 in]
          n968 = Equal?(x=w2535, y="DONE") -> (x = y?=w2533:bool)
          n969 = case shown="True" w2533 {
            tunnel: [w2538 w2539] -> w2532
            tunnel: w2529 -> [w2538 w2540]
            frame False {
            }
            frame True {
              n970 = Increment(x=w2540) -> (x+1=w2539:i32)
            }
          }
        }
        frame 282 {
          n971 = call-dynamic "Write cmd.vi"("error in (no error)"=w2546, "cmd"="GET VERTICAL_CLOCK_VOLTAGE", "Device in"=w2544) -> ("error out"=w2545:errorcluster, "Device out"=w2547:refnum<class "Channel.lvclass">)  [unwired: 7 in]
          n972 = Increment(x=w2542) -> (x+1=w2543:i32)
        }
        frame 283 {
          n973 = call-dynamic "Read resp.vi"("error in (no error)"=w2558, "Device in"=w2559) -> ("error out"=w2556:errorcluster, "resp"=w2551:string, "Device out"=w2554:refnum<class "Channel.lvclass">)  [unwired: 7 in]
          n974 = Fract/Exp String To Number(string=w2551) -> (number=w2549:dbl)  [unwired: 3 in, 1 out]
          n975 = Unbundle By Name(w2554) -> ("Interface.lvclass"=w2553:refnum<class "Interface.lvclass">)
          n976 = call "Read Camera Setup.vi"("Interface in"=w2553) -> ("Camera Setup"=w2552:T3)  [unwired: 8 in, 2 out]
          n977 = Unbundle By Name(w2552) -> ("VERTICAL_CLOCK_VOLTAGE"=w2548:u8)
          n978 = Equal?(x=w2548, y=w2549) -> (x = y?=w2550:bool)
          n979 = case shown="True" w2550 {
            tunnel: [w2560 w2561] -> w2557
            tunnel: w2555 -> [w2560 w2562]
            frame False {
            }
            frame True {
              n980 = Increment(x=w2562) -> (x+1=w2561:i32)
            }
          }
        }
        frame 284 {
          n981 = Unbundle By Name(w2571) -> ("Interface.lvclass"=w2570:refnum<class "Interface.lvclass">)
          n982 = call "Read Camera Setup.vi"("Interface in"=w2570) -> ("Camera Setup"=w2565:T3)  [unwired: 8 in, 2 out]
          n983 = Unbundle By Name(w2565) -> ("FRAME_TRANSFER"=w2564:bool)
          n984 = case shown="True" w2564 {
            tunnel: ["T" ("cmd") "F" ("cmd")] -> w2563
            frame True {
            }
            frame False {
            }
          }
          n985 = Concatenate Strings("SET FRAME_TRANSFER " ("cmd"), w2563) -> (w2569:string)
          n986 = call-dynamic "Write cmd.vi"("error in (no error)"=w2573, "cmd"=w2569, "Device in"=w2571) -> ("error out"=w2572:errorcluster, "Device out"=w2574:refnum<class "Channel.lvclass">)  [unwired: 7 in]
          n987 = Increment(x=w2567) -> (x+1=w2568:i32)
        }
        frame 285 {
          n988 = call-dynamic "Read resp.vi"("error in (no error)"=w2584, "Device in"=w2585) -> ("error out"=w2578:errorcluster, "resp"=w2583:string, "Device out"=w2579:refnum<class "Channel.lvclass">)  [unwired: 7 in]
          n989 = Equal?(x=w2583, y="DONE") -> (x = y?=w2581:bool)
          n990 = case shown="True" w2581 {
            tunnel: [w2586 w2587] -> w2580
            tunnel: w2577 -> [w2586 w2588]
            frame False {
            }
            frame True {
              n991 = Increment(x=w2588) -> (x+1=w2587:i32)
            }
          }
        }
        frame 286 {
          n992 = call-dynamic "Write cmd.vi"("error in (no error)"=w2594, "cmd"="GET FRAME_TRANSFER", "Device in"=w2592) -> ("error out"=w2593:errorcluster, "Device out"=w2595:refnum<class "Channel.lvclass">)  [unwired: 7 in]
          n993 = Increment(x=w2590) -> (x+1=w2591:i32)
        }
        frame 287 {
          n994 = call-dynamic "Read resp.vi"("error in (no error)"=w2606, "Device in"=w2607) -> ("error out"=w2604:errorcluster, "resp"=w2598:string, "Device out"=w2602:refnum<class "Channel.lvclass">)  [unwired: 7 in]
          n995 = Unbundle By Name(w2602) -> ("Interface.lvclass"=w2601:refnum<class "Interface.lvclass">)
          n996 = call "Read Camera Setup.vi"("Interface in"=w2601) -> ("Camera Setup"=w2600:T3)  [unwired: 8 in, 2 out]
          n997 = Unbundle By Name(w2600) -> ("FRAME_TRANSFER"=w2597:bool)
          n998 = case shown="True" w2597 {
            tunnel: ["T" "F"] -> w2596
            frame True {
            }
            frame False {
            }
          }
          n999 = Equal?(x=w2596, y=w2598) -> (x = y?=w2599:bool)
          n1000 = case shown="True" w2599 {
            tunnel: [w2610 w2611] -> w2605
            tunnel: w2603 -> [w2610 w2612]
            frame False {
            }
            frame True {
              n1001 = Increment(x=w2612) -> (x+1=w2611:i32)
            }
          }
        }
        frame 288 {
          n1002 = Unbundle By Name(w2621) -> ("Interface.lvclass"=w2620:refnum<class "Interface.lvclass">)
          n1003 = call "Read Camera Setup.vi"("Interface in"=w2620) -> ("Camera Setup"=w2614:T3)  [unwired: 8 in, 2 out]
          n1004 = Unbundle By Name(w2614) -> ("AD_CHANNEL"=w2613:u32)
          n1005 = Number To Fractional String(number=w2613) -> (F-format string=w2615:string)  [unwired: 3 in]
          n1006 = Concatenate Strings("SET AD_CHANNEL " ("cmd"), w2615) -> (w2619:string)
          n1007 = call-dynamic "Write cmd.vi"("error in (no error)"=w2623, "cmd"=w2619, "Device in"=w2621) -> ("error out"=w2622:errorcluster, "Device out"=w2624:refnum<class "Channel.lvclass">)  [unwired: 7 in]
          n1008 = Increment(x=w2617) -> (x+1=w2618:i32)
        }
        frame 289 {
          n1009 = call-dynamic "Read resp.vi"("error in (no error)"=w2632, "Device in"=w2633) -> ("error out"=w2626:errorcluster, "resp"=w2631:string, "Device out"=w2627:refnum<class "Channel.lvclass">)  [unwired: 7 in]
          n1010 = Equal?(x=w2631, y="DONE") -> (x = y?=w2629:bool)
          n1011 = case shown="True" w2629 {
            tunnel: [w2634 w2635] -> w2628
            tunnel: w2625 -> [w2634 w2636]
            frame False {
            }
            frame True {
              n1012 = Increment(x=w2636) -> (x+1=w2635:i32)
            }
          }
        }
        frame 290 {
          n1013 = call-dynamic "Write cmd.vi"("error in (no error)"=w2642, "cmd"="GET AD_CHANNEL", "Device in"=w2640) -> ("error out"=w2641:errorcluster, "Device out"=w2643:refnum<class "Channel.lvclass">)  [unwired: 7 in]
          n1014 = Increment(x=w2638) -> (x+1=w2639:i32)
        }
        frame 291 {
          n1015 = call-dynamic "Read resp.vi"("error in (no error)"=w2654, "Device in"=w2655) -> ("error out"=w2652:errorcluster, "resp"=w2647:string, "Device out"=w2650:refnum<class "Channel.lvclass">)  [unwired: 7 in]
          n1016 = Fract/Exp String To Number(string=w2647) -> (number=w2645:dbl)  [unwired: 3 in, 1 out]
          n1017 = Unbundle By Name(w2650) -> ("Interface.lvclass"=w2649:refnum<class "Interface.lvclass">)
          n1018 = call "Read Camera Setup.vi"("Interface in"=w2649) -> ("Camera Setup"=w2648:T3)  [unwired: 8 in, 2 out]
          n1019 = Unbundle By Name(w2648) -> ("AD_CHANNEL"=w2644:u32)
          n1020 = Equal?(x=w2644, y=w2645) -> (x = y?=w2646:bool)
          n1021 = case shown="True" w2646 {
            tunnel: [w2656 w2657] -> w2653
            tunnel: w2651 -> [w2656 w2658]
            frame False {
            }
            frame True {
              n1022 = Increment(x=w2658) -> (x+1=w2657:i32)
            }
          }
        }
        frame 300 {
          # "Carrega timeout de 50 ciclos\npara resposta do ACS"
          n1023 = call-dynamic "Write Timer.vi"("error in (no error)"=w2666, "Timer"=u32 50, "State Machine in"=w2665) -> ("error out"=w2668:errorcluster, "State Machine out"=w2670:refnum<class "State Machine.lvclass">)  [unwired: 7 in]
          n1024 = call-dynamic "Write State Machine.vi"("error in (no error)"=w2668, "State Machine.lvclass"=w2670, "Device in"=w2667) -> ("error out"=w2661:errorcluster, "Device out"=w2660:refnum<class "Channel.lvclass">)  [unwired: 7 in]
          n1025 = Unbundle By Name(w2660) -> ("TCS mode"=w2659:string)
          n1026 = Concatenate Strings("SET TCSMODE " ("cmd"), w2659) -> (w2662:string)
          n1027 = call-dynamic "Write cmd.vi"("error in (no error)"=w2661, "cmd"=w2662, "Device in"=w2660) -> ("error out"=w2672:errorcluster, "Device out"=w2673:refnum<class "Channel.lvclass">)  [unwired: 7 in]
          n1028 = Increment(x=w2664) -> (x+1=w2671:i32)
        }
        frame 301 {
          n1029 = call "Verify Timer.vi"("error in (no error)"=w2678, "State Machine in"=w2679) -> ("error out"=w2683:errorcluster, "timeout"=w2675:bool, "State Machine out"=w2684:refnum<class "State Machine.lvclass">)  [unwired: 7 in]
          n1030 = call-dynamic "Write State Machine.vi"("error in (no error)"=w2683, "State Machine.lvclass"=w2684, "Device in"=w2682) -> ("error out"=w2680:errorcluster, "Device out"=w2681:refnum<class "Channel.lvclass">)  [unwired: 7 in]
          n1031 = call-dynamic "Read resp.vi"("error in (no error)"=w2680, "Device in"=w2681) -> ("error out"=w2685:errorcluster, "resp"=w2688:string, "Device out"=w2686:refnum<class "Channel.lvclass">)  [unwired: 7 in]
          n1032 = Equal?(x=w2688, y="DONE") -> (x = y?=w2674:bool)
          n1033 = case shown="False" w2675 {
            tunnel: [w2690 0] -> w2677
            tunnel: w2676 -> [w2691 _]
            tunnel: w2674 -> [w2689 _]
            frame False {
              n1034 = case shown="True" w2689 {
                tunnel: [w2692 w2693] -> w2690
                tunnel: w2691 -> [w2692 w2694]
                frame False {
                }
                frame True {
                  n1035 = Increment(x=w2694) -> (x+1=w2693:i32)
                }
              }
            }
            frame True {
            }
          }
        }
        frame 302 {
          # "Carrega timeout de 50 ciclos\npara resposta do ACS"
          n1036 = call-dynamic "Write Timer.vi"("error in (no error)"=w2703, "Timer"=u32 50, "State Machine in"=w2702) -> ("error out"=w2705:errorcluster, "State Machine out"=w2707:refnum<class "State Machine.lvclass">)  [unwired: 7 in]
          n1037 = call-dynamic "Write State Machine.vi"("error in (no error)"=w2705, "State Machine.lvclass"=w2707, "Device in"=w2704) -> ("error out"=w2698:errorcluster, "Device out"=w2697:refnum<class "Channel.lvclass">)  [unwired: 7 in]
          n1038 = Unbundle By Name(w2697) -> ("ICS mode"=w2696:string)
          n1039 = Concatenate Strings("SET ICSMODE " ("cmd"), w2696) -> (w2699:string)
          n1040 = call-dynamic "Write cmd.vi"("error in (no error)"=w2698, "cmd"=w2699, "Device in"=w2697) -> ("error out"=w2709:errorcluster, "Device out"=w2710:refnum<class "Channel.lvclass">)  [unwired: 7 in]
          n1041 = Increment(x=w2701) -> (x+1=w2708:i32)
        }
        frame 303 {
          n1042 = call "Verify Timer.vi"("error in (no error)"=w2715, "State Machine in"=w2716) -> ("error out"=w2720:errorcluster, "timeout"=w2712:bool, "State Machine out"=w2721:refnum<class "State Machine.lvclass">)  [unwired: 7 in]
          n1043 = call-dynamic "Write State Machine.vi"("error in (no error)"=w2720, "State Machine.lvclass"=w2721, "Device in"=w2719) -> ("error out"=w2717:errorcluster, "Device out"=w2718:refnum<class "Channel.lvclass">)  [unwired: 7 in]
          n1044 = call-dynamic "Read resp.vi"("error in (no error)"=w2717, "Device in"=w2718) -> ("error out"=w2722:errorcluster, "resp"=w2725:string, "Device out"=w2723:refnum<class "Channel.lvclass">)  [unwired: 7 in]
          n1045 = Equal?(x=w2725, y="DONE") -> (x = y?=w2711:bool)
          n1046 = case shown="False" w2712 {
            tunnel: [w2727 0] -> w2714
            tunnel: w2713 -> [w2728 _]
            tunnel: w2711 -> [w2726 _]
            frame False {
              n1047 = case shown="True" w2726 {
                tunnel: [w2729 0 ("State")] -> w2727
                tunnel: w2728 -> [w2729 _]
                frame False {
                }
                frame True {
                }
              }
            }
            frame True {
            }
          }
        }
      }
      n1048 = call-dynamic "Read State Machine.vi"("error in (no error)"=w7, "Device in"=w14) -> ("error out"=w10:errorcluster, "State Machine.lvclass"=w13:refnum<class "State Machine.lvclass">, "Device out"=w12:refnum<class "Channel.lvclass">)  [unwired: 7 in]
      n1049 = call "Next State.vi"("error in (no error)"=w10, "New_State"=w8, "State Machine in"=w13) -> ("error out"=w9:errorcluster, "State Machine out"=w15:refnum<class "State Machine.lvclass">)  [unwired: 7 in]
      n1050 = call-dynamic "Write State Machine.vi"("error in (no error)"=w9, "State Machine.lvclass"=w15, "Device in"=w12) -> ("error out"=w6:errorcluster, "Device out"=w11:refnum<class "Channel.lvclass">)  [unwired: 7 in]
    }
    frame Error {
    }
  }
  "error out" <- w3
  "Channel out" <- w1
